vi "COD主界面（列队使用）.vi"() -> (8 "多列列表框":i32(listbox))   [LabVIEW 2016, in "斯坦道CODMn.lvlib"]
uses:
  <vilib>/Analysis/6fits.llb/Curve Fitting Criteria.ctl
  <vilib>/Utility/miscctls.llb/LVPointTypeDef.ctl
  <vilib>/Utility/config.llb/Read Key (I32).vi
  <vilib>/Utility/config.llb/Read Key (Double).vi
  <vilib>/Utility/config.llb/Read Key (Boolean).vi
  <vilib>/Utility/config.llb/Write Key (I32).vi
  <vilib>/Utility/config.llb/Write Key (Double).vi
  <vilib>/Utility/config.llb/Write Key (Boolean).vi
  <vilib>/Waveform/WDTFileIO.llb/Read Waveform from File.vi
  <vilib>/ptbypt/NI_PtbyPt.lvlib
  <vilib>/Utility/config.llb/NI_LVConfig.lvlib
  <vilib>/Analysis/NI_AALPro.lvlib
panel:
  in  "温度曲线":bool
  out "温度波形时间":timestamp
  in  "历史波形 2":bool
  out "时间-温度":u16[](array[numeric]) caption="数组"
  in  "关闭 4":bool
  out "时间温度曲线":u16[](graph)
  in  "加标回收量程：":enum32{"H", "L", "AUTO"}(ring)=enum."AUTO"
  in  "定时设置":cluster{"启动":bool, "控制命令":T1, "测量参数":T2}(xcontrol)
  out "氢氧化钠":dbl
  in  "序列号变更":bool
  out "模块版本号":string
  in  "更新程序":bool
  out "进样无液体告警":bool
  out "校准内容显示":string
  out "60分钟超时报警":bool
  in  "远程校准量程":enum16{"L", "H"}(ring)
  in  "远程自动校准浓度":dbl
  in  "仪器参数":bool
  out "CODMn序列号":string
  out "CODMn软件版本：":string
  in  "标样核查量程选择":enum32{"H", "L", "AUTO"}(ring)=enum."AUTO"
  in  "标样浓度":dbl
  in  "零点核查量程选择":enum32{"H", "L", "AUTO"}(ring)=enum."AUTO"
  in  "零点核查浓度":dbl
  out "序列号":string
  in  "采水泵排液时间/s:":i32
  in  "采水泵润洗时间/s:":i32
  in  "采水泵沉淀时间/s:":i32
  in  "采水泵进样时间/s:":i32
  in  "常规版/认证版":enum16{"常规版-酸性", "常规版-碱性", "认证版", "浮台版"}(ring)
  in  "释放串口":bool
  in  "打开串口":bool
  in  "保存参数":dbl[](array[numeric])
  out "报警数字":i16
  out "CODMn工作状态":T3(ring)
  out "ORP-K":string
  out "ORP-B":string
  out "ORP-A":string
  out "x = y?":bool
  out "稀释倍数解释":string
  in  "跨度量程选择":enum32{"H", "L", "AUTO"}(ring)=enum."AUTO"
  in  "跨度液浓度":dbl
  in  "水样：":dbl
  in  "蒸馏水：":dbl
  in  "标液：":dbl
  in  "零点核查样：":dbl
  in  "加标回收样：":dbl
  in  "草酸钠":dbl
  in  "高锰酸钾":dbl
  in  "硫酸":dbl
  out "量程解释说明":string
  in  "高切低阈值:":dbl
  in  "低切高阈值:":dbl
  in  "水样量程选择:":enum16{"L", "H", "自动切换测一次", "自动切换测两次"}(ring)
  in  "氢氧化钠：":dbl
  in  "标准液浓度":dbl
  in  "温度":dbl
  in  "恒温时间":dbl
  in  "当前量程：":enum16{"L", "H"}(ring)
  in  "CODMn零点核查选择":enum16{"零点核查走纯水管", "零点核查走零漂管"}(ring)
  in  "锁定按钮":bool
  in  "低量程稀释倍数:":i8=1
  in  "高量程稀释倍数:":i8=2
  in  "一键写入":bool
  in  "测量模式(公式)":u16(ring)=1 items=["水样测试"=1, "标样核查"=2, "零点核查"=3, "跨度核查"=4, "空白测试"=5, "平行样"=6, "加标回收"=7]
  out "基本量程(显示)":string
  out "测量模式(显示)":string
  out "数据时间":string
  out "断电排液标记":bool
  out "COM":string
  in  "启用5":bool
  in  "校准5":bool
  in  "泵滴定数5":dbl
  in  "浓度5":dbl
  in  "启用4":bool
  in  "校准4":bool
  in  "泵滴定数4":dbl
  in  "浓度4":dbl
  out "波形时间":timestamp
  in  "历史波形":bool
  out "滴定数-ORP值":u16[](array[numeric]) caption="数组"
  in  "关闭 3":bool
  in  "滴定曲线":bool
  out "ORP滴定曲线":u16[](graph)
  out "空白测试标记":bool
  out "跨度核查标记":bool
  in  "量程选择":enum16{"低量程", "高量程", "0-2量程"}(ring)
  in  "手动控制":bool
  in  "选用水样":enum16{"葡萄糖", "草酸钠"}(ring)
  in  "方程系数":cluster{"K":dbl, "b":dbl, "X^2":dbl} {"X^2" format="%#.6g"; "b" format="%#.6g"; "K" format="%#.6g"}
  out "多项式系数":dbl[](array[numeric])
  out "XY图":cluster{"X Values":dbl[], "Y Values":dbl[]}[](graph)
  in  "模型":enum32{"线性", "多项式"}(ring)
  out "启动时间":timestamp format="%<%Y/%m/%d %H:%M:%S>T"
  in  "关闭 2":bool
  out "r^2":dbl format="%.8g"
  out "拟合公式":string
  out "b":dbl format="%#.4g"
  out "K":dbl format="%#.4f"
  in  "启用3":bool
  in  "启用2":bool
  in  "启用1":bool
  in  "校准3":bool
  in  "校准2":bool
  in  "校准1":bool
  in  "泵滴定数3":dbl
  in  "泵滴定数2":dbl
  in  "泵滴定数1":dbl
  in  "浓度3":dbl
  in  "浓度2":dbl
  in  "浓度1":dbl
  in  "写入":bool
  out "零点核查标记":bool
  out "排液故障":bool
  out "进水样超量程":bool
  out "标样核查标记":bool
  out "平行样测量":bool
  out "加标回收测量":bool
  out "质控样测量":bool
  out "待机":bool
  out "校标错误":bool
  out "校零错误":bool
  out "测量错误":bool
  out "草酸钠报警":bool
  out "高锰酸钾报警":bool
  out "加热故障":bool
  out "温控器故障":bool
  out "ORP故障":bool
  out "排液标记":bool
  out "故障标记":bool
  out "校标标记":bool
  out "校零标记":bool
  out "通讯状态":bool
  out "水样测量":bool
  in  "读取":bool
  in  "返回":bool
  in  "校准配置":bool
  in  "零点泵计量数 2":dbl
  in  "标度泵计量数 2":dbl
  out "标度滴定值":dbl
  out "零点滴定值":dbl
  in  "保存":bool
  in  "关闭":bool
  out "仪器时间":timestamp format="%<%Y/%m/%d %H:%M:%S>T"
  out "秒":u16
  out "分":u16
  out "COD浓度（mg/L)":dbl format="%.2g"
  out "进样管":dbl
  out "高锰酸钾":dbl
  out "草酸钠":dbl
  out "硫酸":dbl
  out "实时ORP":dbl
  out "温度℃":dbl
  out "加热":bool
  out "搅拌":bool
  out "进硫酸":bool
  out "进加标回收样":bool
  out "进零点核查样":bool
  out "进标液":bool
  out "进蒸馏水":bool
  out "进水样":bool
  out "进草酸钠":bool
  out "进高锰酸钾":bool
  in  "启动":bool
  in  "故障清除":bool
  in  "参数配置":bool
  in  "停止":bool
  in  "单步启动":bool
  out "系统时间":timestamp
  in  "时间校准":bool
  out "模式（受控）":u16
  # "测试时长："
  # "注：遇到加热故障和排液故障时仪器不能正常启动，\n必须排查故障并点击报警清除按钮方可运行。"
  # "mg/L"
  # "基本参数设置"
  # "校零校标结果"
  # "泵计量参数设置"
  # "校零结果："
  # "校零滴定值："
  # "高锰酸钾："
  # "加热恒温温度(℃):"
  # "草酸钠："
  # "校标结果："
  # "标度滴定值："
  # "恒温时间(分钟):"
  # "零点泵计量值："
  # "硫酸："
  # "标准液浓度(mg/L):"
  # "标度泵计量值："
  # "跨度核查浓度："
  # "跨度核查量程："
  # "零点核查浓度："
  # "标样浓度："
  # "零点核查量程："
  # "标样核查量程："
  # "远程校准配置区"
  # "公式读取写入区"
  # "mg/L"
  # "是否启用"
  # "泵滴定数"
  # "浓度"
  # "辅\n助\n计\n算\n区"
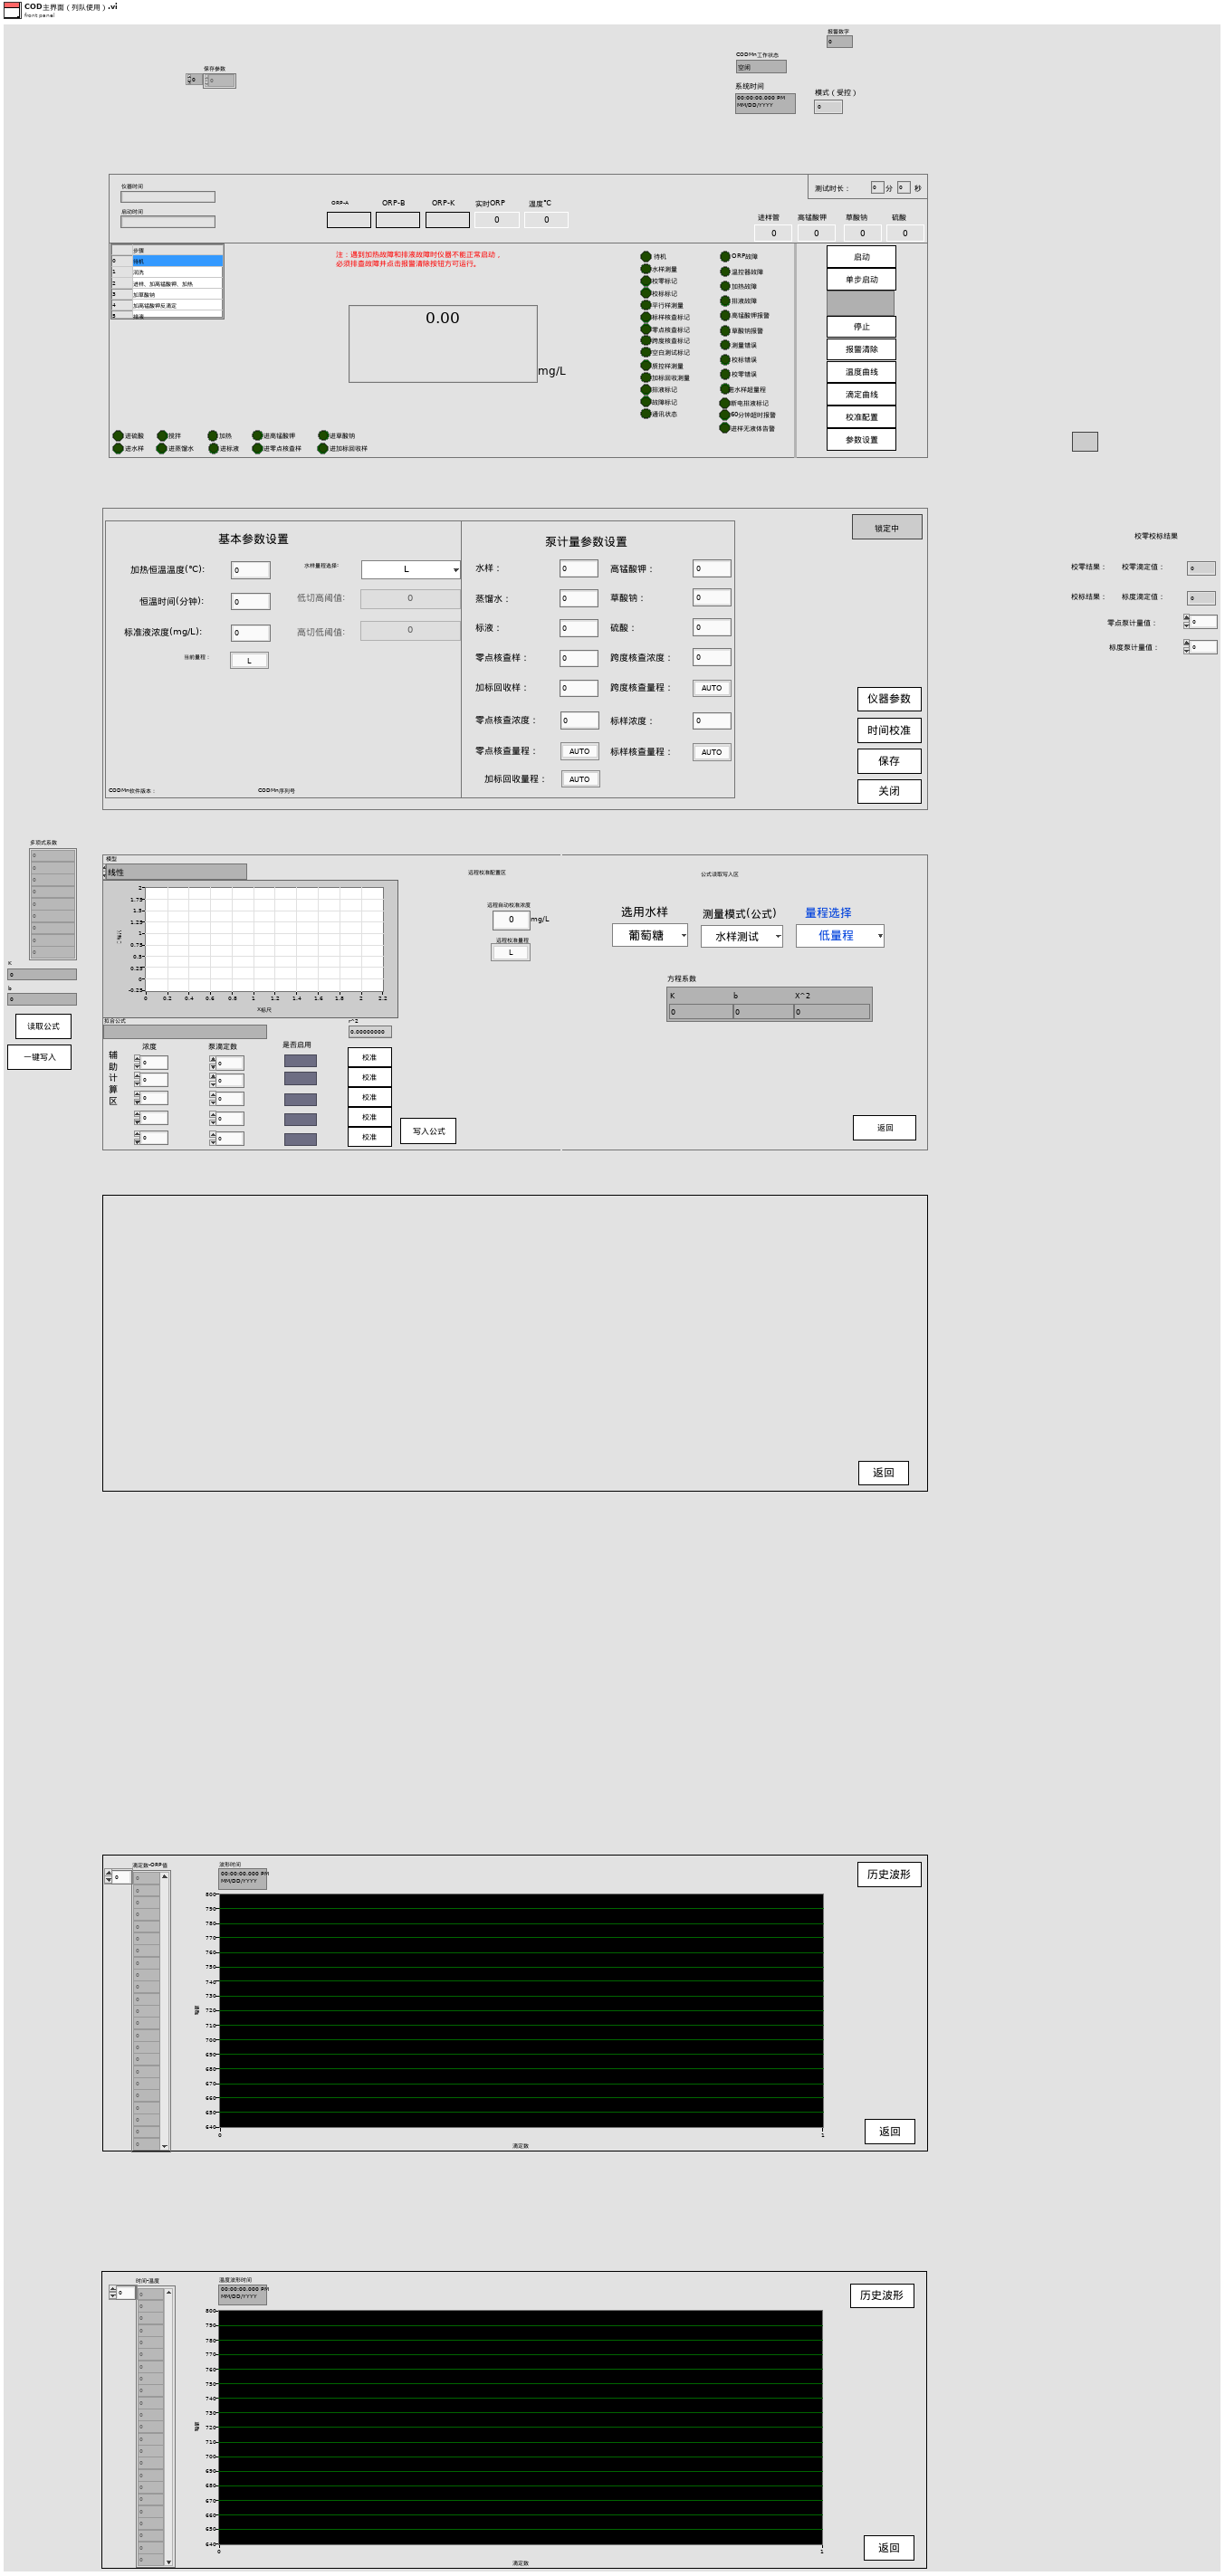
[diagram p1: front panel]
types:
  T1 = typedef "定时设置.xctl/国标控制命令.ctl" = enum16{"启动测量", "标样核查", "零点核查", "跨度核查", "空白测试", "平行样测试", "加标回收", "空白校准", "标样校准", "初始化（清洗）", "停止测试", "仪器重启", "校时", "模式设置", "测量间隔设置"}
  T2 = typedef "定时设置.xctl/测量参数.ctl" = u16
  T3 = enum16{"空闲", "水样测试", "标样核查", "零点核查", "跨度核查", "空白测试", "平行样测试", "质控样", "空白校准", "标样校准", "加标回收"}
  T4 = typedef "LVPointTypeDef.ctl" = cluster{"Horizontal":i16, "Vertical":i16}
  T5 = cluster{"Major":u16, "Minor":u16, "Fix":u16, "Build":u16}
  T6 = typedef "NI_LVConfig.lvlib/Config Data RefNum.ctl" = refnum<k1>
  T7 = cluster{"时间源选择":enum16{"系统时间源", "仪器时间源"}, "外部时间源":timestamp}
  T8 = enum32{"Bad", "Idle", "Run top level", "Running"}
  T9 = enum8{"Enabled", "Disabled", "Disabled and Grayed Out"}
  T10 = cluster{"时间":timestamp, "测量模式":string, "数据类型":string, "检测值":sgl, "单位":string, "数据标识":string, "因子编码":string, "标样参考值":sgl, "ORP-A":sgl, "ORP-B":sgl, "ORP-K":sgl, "COD滴定值":sgl, "高锰酸钾滴定数":sgl, "温度":sgl, "量程":sgl, "LastTime":timestamp, "序列号:":string}
  T11 = cluster{"因子编码":u32, "单位":u16, "标样参考值":sgl, "水样数据时间":timestamp, "水样实测值":sgl, "水样数据标识":string, "标样数据时间":timestamp, "标样实测值":sgl, "标样数据标识":string, "空白数据时间":timestamp, "空白实测值":sgl, "空白数据标识":string, "零点核查数据时间":timestamp, "零点核查实测值":sgl, "零点核查数据标识":string, "跨度核查数据时间":timestamp, "跨度核查实测值":sgl, "跨度核查数据标识":string, "加标回收数据时间":timestamp, "加标回收实测值":sgl, "加标回收数据标识":string, "平行样数据时间":timestamp, "平行样实测值":sgl, "平行样数据标识":string}
  T12 = cluster{"运行模式":enum16{"维护模式", "常规模式", "应急模式", "质控模式"}, "质控频次":enum16{"关闭", "每天", "星期一", "星期二", "星期三", "星期四", "星期五", "星期六", "星期日"}, "空白核查时间":u16, "跨度核查时间":u16, "24H周期设置":bool[]}
  T13 = cluster{"数组 2[0]":sgl, "数组 2[1]":sgl, "数组 2[2]":sgl, "数组 2[3]":sgl, "数组 2[4]":sgl, "数组 2[5]":sgl, "数组 2[6]":sgl, "数组 2[7]":sgl, "数组 2[8]":sgl, "数组 2[9]":sgl, "数组 2[10]":sgl, "数组 2[11]":sgl, "数组 2[12]":sgl, "数组 2[13]":sgl, "数组 2[14]":sgl, "数组 2[15]":sgl, "数组 2[16]":sgl, "数组 2[17]":sgl, "数组 2[18]":sgl, "数组 2[19]":sgl, "数组 2[20]":sgl, "数组 2[21]":sgl, "数组 2[22]":sgl, "数组 2[23]":sgl, "数组 2[24]":sgl, "数组 2[25]":sgl, "数组 2[26]":sgl, "数组 2[27]":sgl, "数组 2[28]":sgl, "数组 2[29]":sgl, "数组 2[30]":sgl, "数组 2[31]":sgl, "数组 2[32]":sgl, "数组 2[33]":sgl, "数组 2[34]":sgl, "数组 2[35]":sgl, "数组 2[36]":sgl, "数组 2[37]":sgl, "数组 2[38]":sgl, "数组 2[39]":sgl, "数组 2[40]":sgl, "数组 2[41]":sgl}
  T14 = cluster{"ORP故障":bool, "温控器故障":bool, "加热故障":bool, "高锰酸钾报警":bool, "草酸钠报警":bool, "测量错误":bool, "校零错误":bool, "校标错误":bool, " 进水样超量程":bool, "排液阀故障":bool, "60分钟超时报警":bool, "进样无液体报警":bool}
  T15 = cluster{"时间标识":timestamp, "参数":string, "日志信息":string, "流程参数":string}
  T16 = cluster{"测量量程":dbl, "测量精度":dbl, "测量间隔":dbl, "消解温度":dbl, "消解时长":dbl, "空白校准时间":timestamp, "曲线截距":dbl, "曲线斜率":dbl, "测量检出限":dbl, "测量信号值":dbl, "线性相关系数":dbl, "二次多项式系数":dbl, "标样校准时间":timestamp, "稀释倍数":dbl, "三项式系数":dbl, "空白标定系数":dbl, "量程系数":dbl, "F0/ORPA":dbl, "F1/ORPB":dbl, "F2/ORPK":dbl, "F3":dbl, "F4":dbl, "F5":dbl, "F6":dbl, "F7":dbl, "X0/滴定数":dbl, "量程":dbl}
  T17 = cluster{"确定":bool, "测量量程":dbl, "测量精度":dbl, "测量间隔":dbl, "消解温度":dbl, "消解时长":dbl, "空白校准时间":timestamp, "曲线截距":dbl, "曲线斜率":dbl, "测量检出限":dbl, "测量信号值":dbl, "线性相关系数":dbl, "二次多项式系数":dbl, "标样校准时间":timestamp, "稀释倍数":dbl, "三项式系数":dbl, "空白标定系数":dbl, "量程系数":dbl, "F0/ORPA":dbl, "F1/ORPB":dbl, "F2/ORPK":dbl, "F3":dbl, "F4":dbl, "F5":dbl, "F6":dbl, "F7":dbl, "X0/滴定数":dbl, "量程":dbl}
  T18 = enum16{"Left Button", "Center Button", "Right Button", "Window Close"}
  T19 = cluster{"时间标识":timestamp, "设备":string, "日志信息":string, "流程参数":string}
  T20 = typedef "NI_AALPro.lvlib/Curve Fitting Criteria.ctl" = u16
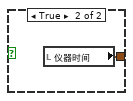
[diagram p2: hidden frame]
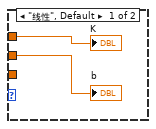
[diagram p8: hidden frame]
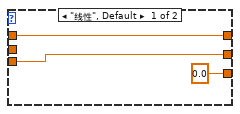
[diagram p10: hidden frame]
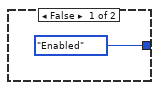
[diagram p11: hidden frame]
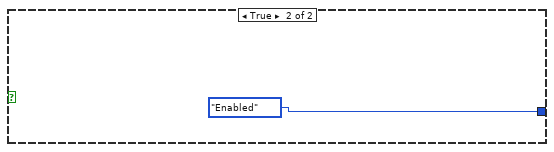
[diagram p12: hidden frame]
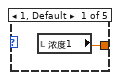
[diagram p17: hidden frame]
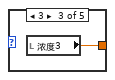
[diagram p18: hidden frame]
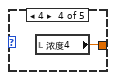
[diagram p19: hidden frame]
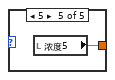
[diagram p20: hidden frame]
diagram:
  n1 = flat-sequence {
    tunnel: w3 -> [_]
    frame #0 {
      w29 = u16 1 items=["水样测试"=1, "标样核查"=2, "零点核查"=3, "跨度核查"=4, "空白测试"=5, "平行样"=6, "加标回收"=7] ("测量模式(公式)")
      n2 = vi-ref "斯坦道CODMn.lvlib:待机状态数据存储写入和切换量程(子VI).vi"() -> (w65:refnum<vi>)
      n3 = vi-ref "斯坦道CODMn.lvlib:日志报警状态存储 (子VI).vi"() -> (w58:refnum<vi>)
      n4 = vi-ref "斯坦道CODMn.lvlib:高锰酸钾-ORP滴定曲线(子VI).vi"() -> (w45:refnum<vi>)
      n5 = property class="VI"(reference=w58, error in=errorcluster {"status"=FALSE, "code"=0, "source"=""} ("错误输出")) -> ("Name"=w57:string)  [unwired: 2 out]
      n6 = property class="VI"(reference=w45, error in=errorcluster {"status"=FALSE, "code"=0, "source"=""} ("错误输出")) -> ("Name"=w46:string)  [unwired: 2 out]
      n7 = property class="VI"(reference=w65, error in=errorcluster {"status"=FALSE, "code"=0, "source"=""} ("错误输出")) -> ("Name"=w64:string)  [unwired: 2 out]
      n8 = Open VI Reference(type specifier VI Refnum (for type only)=refnum<vi> refnum, vi path=w57, options=128 ("选项")) -> (vi reference=w41:refnum<vi>, error out=w55:errorcluster)  [unwired: 3 in]
      n9 = Open VI Reference(type specifier VI Refnum (for type only)=refnum<vi> refnum, vi path=w46, options=128 ("选项")) -> (vi reference=w44:refnum<vi>, error out=w48:errorcluster)  [unwired: 3 in]
      n10 = call-by-ref "?"(reference=w41, error in=w55) -> (reference out=w53:refnum<vi>, error out=w54:errorcluster)  [unwired: 12 in]
      n11 = call-by-ref "?"(reference=w44, error in=w48) -> (reference out=w50:refnum<vi>, error out=w49:errorcluster)  [unwired: 12 in]
      n12 = Open VI Reference(type specifier VI Refnum (for type only)=refnum<vi> refnum, vi path=w64, options=128 ("选项")) -> (vi reference=w39:refnum<vi>, error out=w62:errorcluster)  [unwired: 3 in]
      n13 = Close Reference(reference=w53, error in (no error)=w54) -> ()  [unwired: 1 out]
      n14 = call-by-ref "?"(reference=w39, error in=w62) -> (reference out=w60:refnum<vi>, error out=w61:errorcluster)  [unwired: 12 in]
      n15 = Close Reference(reference=w50, error in (no error)=w49) -> ()  [unwired: 1 out]
      n16 = Close Reference(reference=w60, error in (no error)=w61) -> ()  [unwired: 1 out]
      n17 = vi-ref "斯坦道CODMn.lvlib:时间-温度曲线(子VI).vi"() -> (w24:refnum<vi>)
      n18 = vi-ref "斯坦道CODMn.lvlib:关键参数交互.vi"() -> (w36:refnum<vi>)
      n19 = property class="VI"(reference=w36, error in=errorcluster {"status"=FALSE, "code"=0, "source"=""} ("错误输出")) -> ("Name"=w35:string)  [unwired: 2 out]
      n20 = property class="VI"(reference=w24, error in=errorcluster {"status"=FALSE, "code"=0, "source"=""} ("错误输出")) -> ("Name"=w23:string)  [unwired: 2 out]
      n21 = Open VI Reference(type specifier VI Refnum (for type only)=refnum<vi> refnum, vi path=w35, options=128 ("选项")) -> (vi reference=w37:refnum<vi>, error out=w33:errorcluster)  [unwired: 3 in]
      n22 = call-by-ref "?"(reference=w37, error in=w33, "量程选择"=enum16{"低量程", "高量程", "0-2量程"}."低量程", "测量模式(公式)"=w29, "模型"=enum32{"线性", "多项式"}."线性") -> (reference out=w31:refnum<vi>, error out=w32:errorcluster)  [unwired: 9 in]
      n23 = Open VI Reference(type specifier VI Refnum (for type only)=refnum<vi> refnum, vi path=w23, options=128 ("选项")) -> (vi reference=w25:refnum<vi>, error out=w21:errorcluster)  [unwired: 3 in]
      n24 = call-by-ref "?"(reference=w25, error in=w21) -> (reference out=w19:refnum<vi>, error out=w20:errorcluster)  [unwired: 12 in]
      n25 = Close Reference(reference=w31, error in (no error)=w32) -> ()  [unwired: 1 out]
      n26 = Close Reference(reference=w19, error in (no error)=w20) -> ()  [unwired: 1 out]
    }
  }
  n27 = property on="定时设置" class="定时设置 (严格)"("引用参数"="CODMn") -> (error out=w1:errorcluster)  [unwired: 2 in, 1 out]
  n28 = flat-sequence {
    tunnel: [w68] -> w5
    tunnel: [errorcluster {"status"=FALSE, "code"=0, "source"=""} ("错误输出")] -> w3
    tunnel: [w70] -> w4
    frame #0 {
      w92 = "192.168.1.100" ("名称")
      n29 = global write "COD内部交互全局.vi" "量程切换次数"(u8 0 ("量程切换次数")) -> ()
      n30 = global write "COD内部交互全局.vi" "切换量程连续测两次"(FALSE ("切换量程连续测两次")) -> ()
      n31 = global read "COD内部交互全局.vi" "序列号:"() -> (w99:string)
      n32 = property on="窗格" class="Pane"("Origin"=T4 {"Horizontal"=0, "Vertical"=0} ("原点")) -> ()  [unwired: 2 in, 2 out]
      n33 = Empty String/Path?(string/path=w99) -> (empty?=w67:bool)
      n34 = case shown="真" w67 {
        tunnel: w99 -> [w114 _]
        tunnel: [w113 "data\\CODMnSet.ini" ("名称或相对路径")] -> w80
        frame False {
          # "与生产用上位机交互"
          n35 = Concatenate Strings("data\\" ("字符串"), "序列号" ("字符串"), w114, "Set.ini" ("名称或相对路径")) -> (w113:string)
        }
        frame True {
        }
      }
      n36 = String To IP(1:w92) -> (0:w85:u32)
      n37 = IP To String(2:w85) -> (0:w88:string)  [unwired: 1 in]
      n38 = Not Equal?(x=w92, y=w88) -> (x != y?=w93:bool)
      n39 = Concatenate Strings("\\\\" ("字符串"), w88) -> (w87:string)
      n40 = global write "CODMN外部API.vi" "ping"(w93) -> ()
      n41 = String To Path(string=w87) -> (path=w94:path)
      n42 = Build Path(base path=w94, name or relative path=w80) -> (appended path=w89:path)
      n43 = local write "量程选择"(enum16{"低量程", "高量程", "0-2量程"}."低量程" ("量程选择")) -> ()
      n44 = local write "选用水样"(enum16{"葡萄糖", "草酸钠"}."葡萄糖" ("选用水样")) -> ()
      n45 = global write "COD内部交互全局.vi" "配置文件ini"(w80) -> ()
      n46 = case shown="真" w93 {
        tunnel: w89 -> [w104 w108]
        tunnel: [w104 w107] -> w90
        tunnel: [FALSE w106] -> w91
        frame False {
        }
        frame True {
          n47 = call <vilib>:"Check if File or Folder Exists.vi"("path"=w108) -> ("file or folder exists?"=w106:bool, "dup path"=w107:path)  [unwired: 8 in, 1 out]
        }
      }
      n48 = control-ref of="本VI"() -> (w79:refnum<vi>)
      n49 = case shown="假" w91 {
        tunnel: w90 -> [_ w112]
        tunnel: [w110 w112] -> w71
        tunnel: w80 -> [w109 _]
        frame False {
          # "本地文件地址"
          n50 = call <vilib>:"Application Directory.vi"() -> ("Application Directory"=w111:path)
          n51 = Build Path(base path=w111, name or relative path=w109) -> (appended path=w110:path)
        }
        frame True {
          # "网络共享地址"
        }
      }
      n52 = property class="VI"(reference=w79) -> ("Library.Version"=w78:T5)  [unwired: 1 in, 2 out]
      n53 = Unbundle By Name(w78) -> ("Major"=w76:u16, "Minor"=w75:u16, "Fix"=w74:u16, "Build"=w73:u16)
      n54 = Format Into String(format string="模块版本号：%d.%d.%d.%d" ("格式字符串"), w76, w75, w74, w73) -> (resulting string=→"模块版本号":string)  [unwired: 2 in, 1 out]
      n55 = global write "CODMN外部API.vi" "配置文件 path"(w71) -> ()
      n56 = call <vilib>:"Open Config Data.vi"("configuration file path"=w71) -> ("error out"=w81:errorcluster, "refnum"=w82:T6)  [unwired: 8 in, 1 out]
      n57 = vi-ref "斯坦道CODMn.lvlib:CODMn断电保存全局变量.vi"() -> (w95:refnum<vi>)
      n58 = call <userlib>:"Read Panel from INI__ogtk.vi"("error in (no error)"=w81, "VI ref"=w95, "refnum"=w82) -> ("error out"=w83:errorcluster, "refnum out"=w84:T6)  [unwired: 7 in]
      n59 = call <vilib>:"Close Config Data.vi"("error in (no error)"=w83, "refnum"=w84) -> ("error out"=w69:errorcluster)  [unwired: 8 in, 1 out]
      n60 = call <vilib>:"Clear Errors.vi"("error in (no error)"=w69) -> ("error out"=w66:errorcluster)  [unwired: 5 in, 1 out]
      n61 = Read from Text File(file (use dialog)=w71, error in=w66) -> (text=w70:string, error out=w68:errorcluster)  [unwired: 2 in, 2 out]
      "稀释倍数解释" <- "稀释倍数解释：\n稀释倍数选择1，表示不稀释\n默认低量程系数倍数1，高量程系数倍数2\n则低量程为0~8，高量程为0~16" ("稀释倍数解释")
    }
  }
  n62 = while {
    tunnel: w1 -> [_]
    stop <- FALSE stop-if-true
    n63 = Wait (ms)(milliseconds to wait=u32 500 ("等待时间（毫秒）")) -> ()  [unwired: 1 out]
    n64 = global read "COD测量模式全局.vi" "CODMn工作状态"() -> (w125:T3)
    n65 = local read "通讯状态"() -> (w119:bool)
    n66 = case shown="假" w119 {
      tunnel: [w135 w136] -> w123
      frame False {
        n67 = Get Date/Time In Seconds() -> (seconds since 1Jan1904=w135:timestamp)
      }
      frame True {
        n68 = local read "仪器时间"() -> (w136:timestamp)
      }
    }
    n69 = vi-ref "斯坦道CODMn.lvlib:CODMn测量流程.vi"() -> (w132:refnum<vi>)
    n70 = Bundle By Name(cluster=T7 {"时间源选择"=enum."系统时间源", "外部时间源"=timestamp(0 s since 1904-01-01)} ("时间源"), "时间源选择"=enum16{"系统时间源", "仪器时间源"}."仪器时间源", "外部时间源"=w123) -> (w121:T7)
    n71 = property class="VI"(reference=w132) -> ("Exec.State"=w130:T8, "Name"=w131:string)  [unwired: 1 in, 2 out]
    n72 = Not Equal?(x=w125, y=T3."空闲") -> (x != y?=w120:bool)
    n73 = property on="定时设置" class="定时设置 (严格)"("仪器状态"=w120, "时间源"=w121) -> ()  [unwired: 2 in, 2 out]
    n74 = Unbundle By Name("定时设置") -> ("启动"=w128:bool, "控制命令"=w129:T1)
    n75 = case shown="真" w128 {
      tunnel: w131 -> [_ w139]
      tunnel: w129 -> [_ w138]
      tunnel: w130 -> [_ w137]
      frame False {
      }
      frame True {
        n76 = case shown="\"Idle\"" w137 {
          tunnel: w139 -> [_ w143]
          tunnel: w138 -> [_ w140]
          frame "Bad", Default {
          }
          frame "Idle" {
            n77 = Open VI Reference(type specifier VI Refnum (for type only)=refnum<vi> refnum, vi path=w143, options=128 ("选项")) -> (vi reference=w144:refnum<vi>, error out=w145:errorcluster)  [unwired: 3 in]
            n78 = call-by-ref "开始异步调用"(reference=w144, error in=w145, "控制命令"=w140) -> (reference out=w146:refnum<vi>, error out=w147:errorcluster)  [unwired: 11 in]
            n79 = Close Reference(reference=w146, error in (no error)=w147) -> ()  [unwired: 1 out]
          }
        }
      }
    }
  }
  n80 = Obtain Queue(name (unnamed)="CODMn" ("名称（未命名）"), element data type=cluster{"命令":string} {"命令"="启用模块"} ("元素")) -> (queue out=w15:refnum<queue>, error out=w14:errorcluster)  [unwired: 3 in, 1 out]
  n81 = while {
    tunnel: [w154] -> _
    shift-right: [w152] -> _
    shift-left: w4 -> [w151]
    tunnel: w5 -> [_]
    stop <- FALSE stop-if-true
    n82 = global read "CODMN外部API.vi" "配置文件 path"() -> (w148:path)
    n83 = Wait (ms)(milliseconds to wait=u32 1000 ("等待时间（毫秒）")) -> ()  [unwired: 1 out]
    n84 = Read from Text File(file (use dialog)=w148) -> (text=w152:string, error out=w149:errorcluster)  [unwired: 3 in, 2 out]
    n85 = Not Equal?(x=w152, y=w151) -> (x != y?=w150:bool)
    n86 = case shown="真" w150 {
      tunnel: [w156 w163] -> w154
      tunnel: w148 -> [_ w157]
      tunnel: w149 -> [w156 _]
      frame False {
      }
      frame True {
        # "文件发生改变进行更新，远端和本地都更新"
        n87 = vi-ref "斯坦道CODMn.lvlib:CODMn断电保存全局变量.vi"() -> (w158:refnum<vi>)
        n88 = call <vilib>:"Open Config Data.vi"("configuration file path"=w157) -> ("error out"=w162:errorcluster, "refnum"=w161:T6)  [unwired: 8 in, 1 out]
        n89 = call <userlib>:"Read Panel from INI__ogtk.vi"("error in (no error)"=w162, "VI ref"=w158, "refnum"=w161) -> ("error out"=w160:errorcluster, "refnum out"=w159:T6)  [unwired: 7 in]
        n90 = call <vilib>:"Close Config Data.vi"("error in (no error)"=w160, "refnum"=w159) -> ("error out"=w163:errorcluster)  [unwired: 8 in, 1 out]
      }
    }
  }
  n91 = vi-ref "CODMn通讯.vi"() -> (w6:refnum<vi>)
  n92 = while {
    tunnel: w5 -> [_]
    stop <- FALSE stop-if-true
    # "赋值循环"
    n93 = flat-sequence {
      frame #0 {
        # "测量数据区"
        n94 = global read "COD内部交互全局.vi" "data"() -> (w408:T10)
        n95 = global read "COD测量模式全局.vi" "测量模式文字实时"() -> (w394:string)
        "测量模式(显示)" <- w394
        n96 = global read "CODMn断电保存全局变量.vi" "测量数据区"() -> (w403:T11)
        n97 = Unbundle By Name(w408) -> ("时间"=w407:timestamp, "检测值"=w406:sgl, "数据标识"=w405:string)
        n98 = case shown="\"水样测试\"" w394 {
          tunnel: w403 -> [w409 w414 w419 w424 w429 w434 w439 w444 w449 w454]
          tunnel: [w409 w413 w418 w420 w428 w433 w438 w443 w445 w453] -> w404
          tunnel: w407 -> [_ w412 w417 w423 w427 w432 w437 w442 w448 w452]
          tunnel: w406 -> [_ w411 w416 w422 w426 w431 w436 w441 w447 w451]
          tunnel: w405 -> [_ w410 w415 w421 w425 w430 w435 w440 w446 w450]
          frame "", Default {
          }
          frame "水样测试" {
            n99 = Bundle By Name(cluster=w414, "水样数据时间"=w412, "水样实测值"=w411, "水样数据标识"=w410) -> (w413:T11)
          }
          frame "标样核查" {
            n100 = Bundle By Name(cluster=w419, "标样数据时间"=w417, "标样实测值"=w416, "标样数据标识"=w415) -> (w418:T11)
          }
          frame "跨度核查" {
            n101 = Bundle By Name(cluster=w424, "跨度核查数据时间"=w423, "跨度核查实测值"=w422, "跨度核查数据标识"=w421) -> (w420:T11)
          }
          frame "零点核查" {
            n102 = Bundle By Name(cluster=w429, "零点核查数据时间"=w427, "零点核查实测值"=w426, "零点核查数据标识"=w425) -> (w428:T11)
          }
          frame "空白测试" {
            n103 = Bundle By Name(cluster=w434, "空白数据时间"=w432, "空白实测值"=w431, "空白数据标识"=w430) -> (w433:T11)
          }
          frame "加标回收" {
            n104 = Bundle By Name(cluster=w439, "加标回收数据时间"=w437, "加标回收实测值"=w436, "加标回收数据标识"=w435) -> (w438:T11)
          }
          frame "平行样" {
            n105 = Bundle By Name(cluster=w444, "平行样数据时间"=w442, "平行样实测值"=w441, "平行样数据标识"=w440) -> (w443:T11)
          }
          frame "校零" {
            n106 = Bundle By Name(cluster=w449, "空白数据时间"=w448, "空白实测值"=w447, "空白数据标识"=w446) -> (w445:T11)
          }
          frame "校标" {
            n107 = Bundle By Name(cluster=w454, "标样数据时间"=w452, "标样实测值"=w451, "标样数据标识"=w450) -> (w453:T11)
          }
        }
        n108 = Unbundle By Name(w403) -> ("水样实测值"=w400:sgl)
        n109 = feedback-in #1(w403) -> ()
        n110 = feedback #1(w403) -> (w402:T11)
        n111 = global read "CODMn断电保存全局变量.vi" "水样测试量程"() -> (w396:enum16{"L", "H"})
        n112 = Unbundle By Name(w402) -> ("水样实测值"=w401:sgl)
        n113 = feedback #2(w396) -> (w397:enum16{"L", "H"})
        n114 = feedback-in #2(w396) -> ()
        n115 = Not Equal?(x=w397, y=w396) -> (x != y?=w395:bool)
        n116 = Not Equal?(x=w400, y=w401) -> (x != y?=w399:bool)
        n117 = global write "CODMn断电保存全局变量.vi" "测量数据区"(w404) -> ()
        n118 = Or(x=w399, y=w395) -> (x .or. y?=w398:bool)
        n119 = case shown="真" w398 {
          frame False {
          }
          frame True {
            # "水样值发送改变存储本地"
            n120 = call "配置文件保存.vi"() -> ()  [unwired: 12 in]
          }
        }
      }
    }
    n121 = flat-sequence {
      frame #0 {
        # "局部变量给内部交互用全局变量"
        n122 = local read "COD浓度（mg/L)"() -> (w196:dbl)
        n123 = local read "CODMn工作状态"() -> (w199:T3)
        n124 = local read "多列列表框"() -> (w197:i32)
        n125 = local read "标准液浓度"() -> (w195:dbl)
        n126 = local read "温度℃"() -> (w190:dbl)
        n127 = local read "高锰酸钾报警"() -> (w193:bool)
        n128 = local read "断电排液标记"() -> (w192:bool)
        n129 = local read "实时ORP"() -> (w189:dbl)
        n130 = local read "故障标记"() -> (w198:bool)
        n131 = local read "高锰酸钾"() -> (w191:dbl)
        n132 = local read "待机"() -> (w194:bool)
        n133 = global write "COD内部交互全局.vi" "实时温度"(w190) -> ()
        n134 = global write "运行时序全局变量.vi" "多列列表框"(w197) -> ()
        n135 = global write "COD内部交互全局.vi" "故障标记"(w198) -> ()
        n136 = global write "COD内部交互全局.vi" "ORP显示"(w189) -> ()
        n137 = global write "COD浓度全局变量.vi" "标准液浓度"(w195) -> ()
        n138 = global write "COD内部交互全局.vi" "高锰酸钾"(w191) -> ()
        n139 = global write "COD内部交互全局.vi" "待机"(w194) -> ()
        n140 = global write "COD测量模式全局.vi" "CODMn工作状态"(w199) -> ()
        n141 = global write "COD内部交互全局.vi" "高锰酸钾报警"(w193) -> ()
        n142 = global write "COD内部交互全局.vi" "断电排液标记"(w192) -> ()
        n143 = global write "COD浓度全局变量.vi" "COD浓度（mg/L)"(w196) -> ()
      }
    }
    n144 = flat-sequence {
      frame #0 {
        # "断电保存全局给局部变量"
        n145 = global read "CODMn断电保存全局变量.vi" "高切低阈值:"() -> (w471:dbl)
        n146 = global read "CODMn断电保存全局变量.vi" "低切高阈值:"() -> (w470:dbl)
        n147 = global read "CODMn断电保存全局变量.vi" "跨度液浓度"() -> (w468:dbl)
        n148 = global read "COD内部交互全局.vi" "波形时间"() -> (→"波形时间":timestamp)
        n149 = global read "CODMn断电保存全局变量.vi" "启动时间"() -> (→"启动时间":timestamp)
        n150 = global read "CODMn断电保存全局变量.vi" "标样浓度"() -> (w466:dbl)
        n151 = global read "CODMn断电保存全局变量.vi" "CODMn跨度量程选择"() -> (w472:enum32{"H", "L", "AUTO"})
        n152 = global read "CODMn断电保存全局变量.vi" "标样核查量程选择"() -> (w463:enum32{"H", "L", "AUTO"})
        n153 = global read "CODMn断电保存全局变量.vi" "零点核查量程选择"() -> (w465:enum32{"H", "L", "AUTO"})
        n154 = global read "CODMn断电保存全局变量.vi" "加标回收量程选择"() -> (w458:enum32{"H", "L", "AUTO"})
        n155 = global read "COD内部交互全局.vi" "滴定数-ORP值"() -> (→"滴定数-ORP值":u16[])
        n156 = global read "CODMn断电保存全局变量.vi" "常规版/认证版"() -> (w467:enum16{"常规版-酸性", "常规版-碱性", "认证版", "浮台版"})
        n157 = global read "CODMn断电保存全局变量.vi" "自动切换量程:"() -> (w469:enum16{"L", "H", "自动切换测一次", "自动切换测两次"})
        n158 = global read "CODMn断电保存全局变量.vi" "零点核查浓度"() -> (w464:dbl)
        n159 = global read "CODMn断电保存全局变量.vi" "测量模式(公式)"() -> (w473:u16)
        n160 = local write "高切低阈值:"(w471) -> ()
        n161 = local write "跨度液浓度"(w468) -> ()
        n162 = local write "低切高阈值:"(w470) -> ()
        n163 = global read "COD内部交互全局.vi" "ORP滴定曲线"() -> (→"ORP滴定曲线":u16[])
        n164 = local write "标样浓度"(w466) -> ()
        n165 = local write "标样核查量程选择"(w463) -> ()
        n166 = local write "水样量程选择:"(w469) -> ()
        n167 = local write "常规版/认证版"(w467) -> ()
        n168 = local write "零点核查浓度"(w464) -> ()
        n169 = local write "零点核查量程选择"(w465) -> ()
        n170 = local write "加标回收量程："(w458) -> ()
        n171 = local write "测量模式(公式)"(w473) -> ()
        n172 = local write "跨度量程选择"(w472) -> ()
        n173 = global read "COD内部交互全局.vi" "温度波形时间"() -> (→"温度波形时间":timestamp)
        n174 = global read "COD内部交互全局.vi" "时间温度曲线"() -> (→"时间温度曲线":u16[])
        n175 = global read "COD内部交互全局.vi" "时间-温度"() -> (→"时间-温度":u16[])
      }
    }
    n176 = flat-sequence {
      frame #0 {
        # "保存参数赋值"
        n177 = Multiply(x="温度", y=10.0) -> (x*y=w174:dbl)
        n178 = Multiply(x="标准液浓度", y=100.0) -> (x*y=w171:dbl)
        n179 = Build Array(w174, "恒温时间", w171, "氢氧化钠：", "当前量程：", "水样：", "蒸馏水：", "标液：", "零点核查样：", "加标回收样：", "高锰酸钾", "草酸钠", "硫酸", "零点泵计量数 2", "标度泵计量数 2", "高量程稀释倍数:", "低量程稀释倍数:", "CODMn零点核查选择") -> (w168:dbl[])
        n180 = local write "保存参数"(w168) -> ()
      }
    }
    n181 = flat-sequence {
      frame #0 {
        # "显示量程说明"
        n182 = global read "COD内部交互全局.vi" "通讯状态"() -> (→"通讯状态":bool)
        n183 = global read "CODMn断电保存全局变量.vi" "MB通信方式选择"() -> (w474:enum16{"串口", "TCP"})
        n184 = local read "低量程稀释倍数:"() -> (w488:i8)
        n185 = local read "高量程稀释倍数:"() -> (w478:i8)
        n186 = case shown="\"TCP\"" w474 {
          tunnel: [w491 w492] -> w479
          frame "串口", Default {
            n187 = global read "CODMn断电保存全局变量.vi" "VISA resource name"() -> (w491:refnum<visa-resource-name>)
          }
          frame "TCP" {
            n188 = global read "CODMn断电保存全局变量.vi" "IP"() -> (w492:string)
          }
        }
        "COM" <- w479
        n189 = Multiply(x=w488, y=i8 8) -> (x*y=w480:i8)
        n190 = Multiply(x=w478, y=i8 8) -> (x*y=w476:i8)
        n191 = Number To Decimal String(number=w480) -> (decimal integer string=w485:string)  [unwired: 1 in]
        n192 = Number To Decimal String(number=w476) -> (decimal integer string=w483:string)  [unwired: 1 in]
        n193 = Concatenate Strings("L低量程范围:0~" ("量程解释说明"), w485, "(mg/L)\n\nH高量程范围:" ("量程解释说明"), "0" ("字符串"), "~" ("量程解释说明"), w483, "(mg/L)" ("量程解释说明")) -> (→"量程解释说明":string)
      }
    }
    n194 = flat-sequence {
      frame #0 {
        # "参数赋值（只在读取参数时候改变一次）"
        n195 = global read "COD内部交互全局.vi" "读取浮台参数显示"() -> (w201:bool)
        n196 = global read "COD内部交互全局.vi" "读取浮台参数"() -> (w200:u16[])
        n197 = global read "COD内部交互全局.vi" "读取参数显示"() -> (w202:bool)
        n198 = global read "COD内部交互全局.vi" "读取参数"() -> (w203:u16[])
        n199 = case shown="真" w201 {
          tunnel: w200 -> [_ w209]
          frame False {
          }
          frame True {
            n200 = Index Array(array=w209) -> (element #1=w208:u16, element #2=w207:u16, element #3=w206:u16, element #4=w205:u16)  [unwired: 4 in]
            n201 = global write "COD内部交互全局.vi" "读取浮台参数显示"(FALSE ("读取参数显示")) -> ()
            n202 = local write "采水泵进样时间/s:"(w208) -> ()
            n203 = local write "采水泵润洗时间/s:"(w207) -> ()
            n204 = local write "采水泵沉淀时间/s:"(w206) -> ()
            n205 = local write "采水泵排液时间/s:"(w205) -> ()
          }
        }
        n206 = case shown="真" w202 {
          tunnel: w203 -> [_ w227]
          frame False {
          }
          frame True {
            n207 = Index Array(array=w227) -> (element #1=w236:u16, element #2=w248:u16, element #3=w232:u16, element #4=w210:u16, element #5=w235:u16, element #6=w234:u16, element #7=w247:u16, element #8=w246:u16, element #9=w245:u16, element #10=w244:u16, element #11=w243:u16, element #12=w242:u16, element #13=w241:u16, element #14=w240:u16, element #15=w239:u16, element #16=w230:u16, element #17=w229:u16, element #18=w228:u16, element #19=w225:u16, element #20=w224:u16, element #21=w223:u16, element #22=w222:u16, element #23=w221:u16, element #27=w217:u16, element #28=w216:u16, element #29=w215:u16, element #30=w214:u16, element #31=w213:u16)  [unwired: 31 in, 3 out]
            n208 = global write "COD内部交互全局.vi" "读取参数显示"(FALSE ("读取参数显示")) -> ()
            n209 = local write "水样："(w234) -> ()
            n210 = local write "标液："(w246) -> ()
            n211 = local write "硫酸"(w241) -> ()
            n212 = local write "零点核查样："(w245) -> ()
            n213 = local write "加标回收样："(w244) -> ()
            n214 = local write "当前量程："(w235) -> ()
            n215 = local write "蒸馏水："(w247) -> ()
            n216 = local write "恒温时间"(w248) -> ()
            n217 = local write "高锰酸钾"(w243) -> ()
            n218 = local write "草酸钠"(w242) -> ()
            n219 = local write "零点泵计量数 2"(w240) -> ()
            n220 = local write "标度泵计量数 2"(w239) -> ()
            n221 = local write "高量程稀释倍数:"(w230) -> ()
            n222 = local write "低量程稀释倍数:"(w229) -> ()
            n223 = local write "CODMn零点核查选择"(w228) -> ()
            n224 = Build Array(w225, w224, w223, w222, w221) -> (w220:u16[])
            n225 = Build Array(w217, w216, w215, w214, w213) -> (w212:u16[])
            n226 = Divide(x=w236, y=u16 10) -> (x/y=w237:dbl)
            n227 = Divide(x=w232, y=u16 100) -> (x/y=w231:dbl)
            n228 = local write "氢氧化钠："(w210) -> ()
            n229 = local write "温度"(w237) -> ()
            n230 = local write "标准液浓度"(w231) -> ()
            n231 = call "HexToString.vi"("数组"=w212) -> ("字符串"=w211:string)  [unwired: 10 in]
            "CODMn序列号" <- w211
            "序列号" <- w211
            n232 = call "FATEK_HexToString.vi"("数组"=w220) -> ("STRING"=w219:string[])  [unwired: 10 in]
            n233 = Index Array(array=w219) -> (element=→"CODMn软件版本：":string)  [unwired: 1 in]
            n234 = global write "COD内部交互全局.vi" "序列号:"(w211) -> ()
          }
        }
      }
    }
    n235 = flat-sequence {
      frame #0 {
        # "权限隐藏和显示功能"
        n236 = local read "x = y?"() -> (w497:bool)
        n237 = global read "CODMn断电保存全局变量.vi" "CODMn系统周期测试?"() -> (w494:bool)
        n238 = global read "CODMn断电保存全局变量.vi" "运行周期"() -> (w495:T12)
        n239 = property on="更新程序" class="Bool (严格)"("Visible"=w497) -> ()  [unwired: 2 in, 2 out]
        n240 = property on="释放串口" class="Bool"("Visible"=w497) -> ()  [unwired: 2 in, 2 out]
        n241 = property on="打开串口" class="Bool"("Visible"=w497) -> ()  [unwired: 2 in, 2 out]
        n242 = case shown="假" w494 {
          tunnel: w495 -> [_ w521]
          tunnel: [T9."Enabled" ("禁用") w519] -> w493
          frame False {
          }
          frame True {
            n243 = Unbundle By Name(w521) -> ("运行模式"=w520:enum16{"维护模式", "常规模式", "应急模式", "质控模式"})
            n244 = case shown="\"维护模式\", 默认" w520 {
              tunnel: [T9."Enabled" ("禁用") T9."Disabled and Grayed Out" ("禁用") T9."Disabled and Grayed Out" ("禁用") T9."Disabled and Grayed Out" ("禁用")] -> w519
              frame "维护模式", Default {
              }
              frame "常规模式" {
              }
              frame "应急模式" {
              }
              frame "质控模式" {
              }
            }
          }
        }
        n245 = property on="序列号变更" class="Bool"("Visible"=w497) -> ()  [unwired: 2 in, 2 out]
        n246 = property on="常规版/认证版" class="Enum (严格)"("Visible"=w497) -> ()  [unwired: 2 in, 2 out]
        n247 = property on="CODMn零点核查选择" class="Enum (严格)"("Visible"=w497) -> ()  [unwired: 2 in, 2 out]
        n248 = property on="低量程稀释倍数:" class="DigNum (严格)"("Visible"=w497) -> ()  [unwired: 2 in, 2 out]
        n249 = property on="稀释倍数解释" class="Str"("Visible"=w497) -> ()  [unwired: 2 in, 2 out]
        n250 = property on="高量程稀释倍数:" class="DigNum (严格)"("Visible"=w497) -> ()  [unwired: 2 in, 2 out]
        n251 = control-ref of="水样："() -> (w507:refnum<vi>)
        n252 = control-ref of="蒸馏水："() -> (w506:refnum<vi>)
        n253 = control-ref of="标液："() -> (w505:refnum<vi>)
        n254 = control-ref of="零点核查样："() -> (w504:refnum<vi>)
        n255 = control-ref of="加标回收样："() -> (w503:refnum<vi>)
        n256 = local read "水样量程选择:"() -> (w514:enum16{"L", "H", "自动切换测一次", "自动切换测两次"})
        n257 = control-ref of="量程解释说明"() -> (w501:refnum<vi>)
        n258 = control-ref of="氢氧化钠："() -> (w502:refnum<vi>)
        n259 = property on="定时设置" class="定时设置 (严格)"("DisabledEnum"=w493) -> ()  [unwired: 2 in, 2 out]
        n260 = local read "常规版/认证版"() -> (w512:enum16{"常规版-酸性", "常规版-碱性", "认证版", "浮台版"})
        n261 = Not Equal To 0?(x=w514) -> (x != 0?=w513:bool)
        n262 = control-ref of="进样管"() -> (w499:refnum<vi>)
        n263 = case shown="\"浮台版\"" w512 {
          tunnel: [T9."Enabled" ("禁用") T9."Enabled" ("禁用") T9."Disabled and Grayed Out" ("禁用") T9."Enabled" ("禁用")] -> w511
          tunnel: [i32[] [2] ("禁用项[]") i32[] [2] ("禁用项[]") i32[] [] ("禁用项[]") i32[] [2] ("禁用项[]")] -> w510
          tunnel: [w529 w534 T9."Disabled and Grayed Out" ("禁用") w545] -> w509
          tunnel: [w528 FALSE FALSE TRUE] -> w508
          tunnel: [w529 w534 T9."Disabled and Grayed Out" ("禁用") w545] -> w498
          tunnel: [w528 TRUE FALSE FALSE] -> w496
          frame "常规版-酸性", Default {
            w528 = FALSE
            w529 = T9."Enabled" ("禁用")
          }
          frame "常规版-碱性" {
            w534 = T9."Enabled" ("禁用")
          }
          frame "认证版" {
            w540 = u16 1 items=["水样测试"=1, "标样核查"=2, "零点核查"=3, "跨度核查"=4, "空白测试"=5, "平行样"=6, "加标回收"=7] ("测量模式(公式)")
            n264 = global write "CODMn断电保存全局变量.vi" "测量模式(公式)"(w540) -> ()
          }
          frame "浮台版" {
            w545 = T9."Enabled" ("禁用")
          }
        }
        n265 = Build Array(w507, w506, w505, w504, w503, w501, w502, w499) -> (w500:refnum<vi>[])
        n266 = Select(t=T9."Enabled" ("禁用"), s=w513, f=T9."Disabled and Grayed Out" ("禁用")) -> (s? t:f=w515:T9)
        n267 = for {
          tunnel: w500 -> [w527] mode=indexing
          tunnel: w498 -> [w526]
          n268 = property class="Ctl"(reference=w527, "DisabledEnum"=w526) -> ()  [unwired: 1 in, 2 out]
        }
        n269 = property on="低切高阈值:" class="DigNum (严格)"("DisabledEnum"=w515) -> ()  [unwired: 2 in, 2 out]
        n270 = property on="高切低阈值:" class="DigNum (严格)"("DisabledEnum"=w515) -> ()  [unwired: 2 in, 2 out]
        n271 = property on="采水泵润洗时间/s:" class="DigNum (严格)"("Visible"=w508) -> ()  [unwired: 2 in, 2 out]
        n272 = property on="采水泵沉淀时间/s:" class="DigNum (严格)"("Visible"=w508) -> ()  [unwired: 2 in, 2 out]
        n273 = property on="采水泵排液时间/s:" class="DigNum (严格)"("Visible"=w508) -> ()  [unwired: 2 in, 2 out]
        n274 = property on="采水泵进样时间/s:" class="DigNum (严格)"("Visible"=w508) -> ()  [unwired: 2 in, 2 out]
        n275 = property on="一键写入" class="Bool (严格)"("DisabledEnum"=w509) -> ()  [unwired: 2 in, 2 out]
        n276 = property on="量程选择" class="Enum (严格)"("Disabled Items []"=w510) -> ()  [unwired: 2 in, 2 out]
        n277 = property on="测量模式(公式)" class="Ring (严格)"("DisabledEnum"=w511) -> ()  [unwired: 2 in, 2 out]
        n278 = property on="氢氧化钠：" class="DigNum (严格)"("Visible"=w496) -> ()  [unwired: 2 in, 2 out]
        n279 = property on="氢氧化钠" class="DigNum (严格)"("Visible"=w496) -> ()  [unwired: 2 in, 2 out]
      }
    }
    n280 = flat-sequence {
      frame #0 {
        # "公式读取显示（只在读取公式的时候改变一次）"
        n281 = global read "COD内部交互全局.vi" "读取公式显示"() -> (w249:bool)
        n282 = case shown="真" w249 {
          frame False {
          }
          frame True {
            n283 = global write "COD内部交互全局.vi" "读取公式显示"(FALSE ("读取参数显示")) -> ()
            n284 = global read "COD内部交互全局.vi" "读取公式"() -> (w259:u16[])
            n285 = Array Subset(array=w259, index=10 ("索引"), length=84 ("长度")) -> (w254:u16[])
            n286 = One Button Dialog(message="公式读取成功！" ("消息")) -> ()  [unwired: 1 in, 1 out]
            n287 = local read "测量模式(公式)"() -> (w257:u16)
            n288 = call "浮点CDAB转换COD.vi"("数组"=w254) -> ("数组 2"=w255:sgl[])  [unwired: 10 in]
            n289 = Array To Cluster(array=w255) -> (cluster=w258:T13)
            n290 = case shown="6" w257 {
              tunnel: [cluster{"X":dbl, "b":dbl, "X^2":dbl} {"X"=999.0, "b"=999.0, "X^2"=999.0} ("方程系数") w262 w281 w300 w319 w338 w357 w376] -> w256
              tunnel: w258 -> [_ w261 w280 w299 w318 w337 w356 w375]
              frame 0, Default {
              }
              frame 1 {
                n291 = local read "量程选择"() -> (w264:enum16{"低量程", "高量程", "0-2量程"})
                n292 = case shown="\"低量程\", 默认" w264 {
                  tunnel: w261 -> [w271 w275 w279]
                  tunnel: [w270 w274 w278] -> w267
                  tunnel: [w269 w273 w277] -> w266
                  tunnel: [w268 w272 w276] -> w265
                  frame "低量程", Default {
                    n293 = Unbundle By Name(w271) -> ("数组 2[0]"=w270:sgl, "数组 2[1]"=w269:sgl, "数组 2[2]"=w268:sgl)
                  }
                  frame "高量程" {
                    n294 = Unbundle By Name(w275) -> ("数组 2[3]"=w274:sgl, "数组 2[4]"=w273:sgl, "数组 2[5]"=w272:sgl)
                  }
                  frame "0-2量程" {
                    n295 = Unbundle By Name(w279) -> ("数组 2[6]"=w278:sgl, "数组 2[7]"=w277:sgl, "数组 2[8]"=w276:sgl)
                  }
                }
                n296 = Bundle By Name(cluster=cluster{"X":dbl, "b":dbl, "X^2":dbl} {"X"=0.0, "b"=0.0, "X^2"=0.0} ("方程系数"), "X"=w267, "b"=w266, "X^2"=w265) -> (w262:cluster{"X":dbl, "b":dbl, "X^2":dbl})
              }
              frame 2 {
                n297 = local read "量程选择"() -> (w283:enum16{"低量程", "高量程", "0-2量程"})
                n298 = case shown="\"高量程\"" w283 {
                  tunnel: w280 -> [w290 w294 w298]
                  tunnel: [w289 w293 w297] -> w286
                  tunnel: [w288 w292 w296] -> w285
                  tunnel: [w287 w291 w295] -> w284
                  frame "低量程", Default {
                    n299 = Unbundle By Name(w290) -> ("数组 2[6]"=w289:sgl, "数组 2[7]"=w288:sgl, "数组 2[8]"=w287:sgl)
                  }
                  frame "高量程" {
                    n300 = Unbundle By Name(w294) -> ("数组 2[9]"=w293:sgl, "数组 2[10]"=w292:sgl, "数组 2[11]"=w291:sgl)
                  }
                  frame "0-2量程" {
                    n301 = Unbundle By Name(w298) -> ("数组 2[6]"=w297:sgl, "数组 2[7]"=w296:sgl, "数组 2[8]"=w295:sgl)
                  }
                }
                n302 = Bundle By Name(cluster=cluster{"X":dbl, "b":dbl, "X^2":dbl} {"X"=0.0, "b"=0.0, "X^2"=0.0} ("方程系数"), "X"=w286, "b"=w285, "X^2"=w284) -> (w281:cluster{"X":dbl, "b":dbl, "X^2":dbl})
              }
              frame 3 {
                n303 = local read "量程选择"() -> (w302:enum16{"低量程", "高量程", "0-2量程"})
                n304 = case shown="\"高量程\"" w302 {
                  tunnel: w299 -> [w309 w313 w317]
                  tunnel: [w308 w312 w316] -> w305
                  tunnel: [w307 w311 w315] -> w304
                  tunnel: [w306 w310 w314] -> w303
                  frame "低量程", Default {
                    n305 = Unbundle By Name(w309) -> ("数组 2[12]"=w308:sgl, "数组 2[13]"=w307:sgl, "数组 2[14]"=w306:sgl)
                  }
                  frame "高量程" {
                    n306 = Unbundle By Name(w313) -> ("数组 2[15]"=w312:sgl, "数组 2[16]"=w311:sgl, "数组 2[17]"=w310:sgl)
                  }
                  frame "0-2量程" {
                    n307 = Unbundle By Name(w317) -> ("数组 2[6]"=w316:sgl, "数组 2[7]"=w315:sgl, "数组 2[8]"=w314:sgl)
                  }
                }
                n308 = Bundle By Name(cluster=cluster{"X":dbl, "b":dbl, "X^2":dbl} {"X"=0.0, "b"=0.0, "X^2"=0.0} ("方程系数"), "X"=w305, "b"=w304, "X^2"=w303) -> (w300:cluster{"X":dbl, "b":dbl, "X^2":dbl})
              }
              frame 4 {
                n309 = local read "量程选择"() -> (w321:enum16{"低量程", "高量程", "0-2量程"})
                n310 = case shown="\"高量程\"" w321 {
                  tunnel: w318 -> [w328 w332 w336]
                  tunnel: [w327 w331 w335] -> w324
                  tunnel: [w326 w330 w334] -> w323
                  tunnel: [w325 w329 w333] -> w322
                  frame "低量程", Default {
                    n311 = Unbundle By Name(w328) -> ("数组 2[18]"=w327:sgl, "数组 2[19]"=w326:sgl, "数组 2[20]"=w325:sgl)
                  }
                  frame "高量程" {
                    n312 = Unbundle By Name(w332) -> ("数组 2[21]"=w331:sgl, "数组 2[22]"=w330:sgl, "数组 2[23]"=w329:sgl)
                  }
                  frame "0-2量程" {
                    n313 = Unbundle By Name(w336) -> ("数组 2[6]"=w335:sgl, "数组 2[7]"=w334:sgl, "数组 2[8]"=w333:sgl)
                  }
                }
                n314 = Bundle By Name(cluster=cluster{"X":dbl, "b":dbl, "X^2":dbl} {"X"=0.0, "b"=0.0, "X^2"=0.0} ("方程系数"), "X"=w324, "b"=w323, "X^2"=w322) -> (w319:cluster{"X":dbl, "b":dbl, "X^2":dbl})
              }
              frame 5 {
                n315 = local read "量程选择"() -> (w340:enum16{"低量程", "高量程", "0-2量程"})
                n316 = case shown="\"高量程\"" w340 {
                  tunnel: w337 -> [w347 w351 w355]
                  tunnel: [w346 w350 w354] -> w343
                  tunnel: [w345 w349 w353] -> w342
                  tunnel: [w344 w348 w352] -> w341
                  frame "低量程", Default {
                    n317 = Unbundle By Name(w347) -> ("数组 2[24]"=w346:sgl, "数组 2[25]"=w345:sgl, "数组 2[26]"=w344:sgl)
                  }
                  frame "高量程" {
                    n318 = Unbundle By Name(w351) -> ("数组 2[27]"=w350:sgl, "数组 2[28]"=w349:sgl, "数组 2[29]"=w348:sgl)
                  }
                  frame "0-2量程" {
                    n319 = Unbundle By Name(w355) -> ("数组 2[6]"=w354:sgl, "数组 2[7]"=w353:sgl, "数组 2[8]"=w352:sgl)
                  }
                }
                n320 = Bundle By Name(cluster=cluster{"X":dbl, "b":dbl, "X^2":dbl} {"X"=0.0, "b"=0.0, "X^2"=0.0} ("方程系数"), "X"=w343, "b"=w342, "X^2"=w341) -> (w338:cluster{"X":dbl, "b":dbl, "X^2":dbl})
              }
              frame 6 {
                n321 = local read "量程选择"() -> (w359:enum16{"低量程", "高量程", "0-2量程"})
                n322 = case shown="\"高量程\"" w359 {
                  tunnel: w356 -> [w366 w370 w374]
                  tunnel: [w365 w369 w373] -> w362
                  tunnel: [w364 w368 w372] -> w361
                  tunnel: [w363 w367 w371] -> w360
                  frame "低量程", Default {
                    n323 = Unbundle By Name(w366) -> ("数组 2[30]"=w365:sgl, "数组 2[31]"=w364:sgl, "数组 2[32]"=w363:sgl)
                  }
                  frame "高量程" {
                    n324 = Unbundle By Name(w370) -> ("数组 2[33]"=w369:sgl, "数组 2[34]"=w368:sgl, "数组 2[35]"=w367:sgl)
                  }
                  frame "0-2量程" {
                    n325 = Unbundle By Name(w374) -> ("数组 2[6]"=w373:sgl, "数组 2[7]"=w372:sgl, "数组 2[8]"=w371:sgl)
                  }
                }
                n326 = Bundle By Name(cluster=cluster{"X":dbl, "b":dbl, "X^2":dbl} {"X"=0.0, "b"=0.0, "X^2"=0.0} ("方程系数"), "X"=w362, "b"=w361, "X^2"=w360) -> (w357:cluster{"X":dbl, "b":dbl, "X^2":dbl})
              }
              frame 7 {
                n327 = local read "量程选择"() -> (w378:enum16{"低量程", "高量程", "0-2量程"})
                n328 = case shown="\"高量程\"" w378 {
                  tunnel: w375 -> [w385 w389 w393]
                  tunnel: [w384 w388 w392] -> w381
                  tunnel: [w383 w387 w391] -> w380
                  tunnel: [w382 w386 w390] -> w379
                  frame "低量程", Default {
                    n329 = Unbundle By Name(w385) -> ("数组 2[36]"=w384:sgl, "数组 2[37]"=w383:sgl, "数组 2[38]"=w382:sgl)
                  }
                  frame "高量程" {
                    n330 = Unbundle By Name(w389) -> ("数组 2[39]"=w388:sgl, "数组 2[40]"=w387:sgl, "数组 2[41]"=w386:sgl)
                  }
                  frame "0-2量程" {
                    n331 = Unbundle By Name(w393) -> ("数组 2[6]"=w392:sgl, "数组 2[7]"=w391:sgl, "数组 2[8]"=w390:sgl)
                  }
                }
                n332 = Bundle By Name(cluster=cluster{"X":dbl, "b":dbl, "X^2":dbl} {"X"=0.0, "b"=0.0, "X^2"=0.0} ("方程系数"), "X"=w381, "b"=w380, "X^2"=w379) -> (w376:cluster{"X":dbl, "b":dbl, "X^2":dbl})
              }
            }
            n333 = local write "方程系数"(w256) -> ()
          }
        }
      }
    }
    n334 = Wait (ms)(milliseconds to wait=u32 1000 ("等待时间（毫秒）")) -> ()  [unwired: 1 out]
  }
  n335 = while {
    tunnel: w15 -> [w558]
    tunnel: w14 -> [w557]
    tunnel: w5 -> [_]
    stop <- FALSE stop-if-true
    # "主循环界面显示"
    n336 = flat-sequence {
      frame #0 {
        # "A，B，K"
        # "CODMn读取状态"
        n337 = global read "COD内部交互全局.vi" "ORP、时间"() -> (w687:u16[])
        n338 = To Word Integer(number=w687) -> (16bit integer=w708:i16[])
        n339 = Split 1D Array(array=w708, index=3 ("索引")) -> (first subarray=w689:i16[], second subarray=w707:i16[])
        n340 = Index Array(array=w689) -> (element #1=w693:i16, element #2=w692:i16, element #3=w691:i16)  [unwired: 3 in]
        n341 = Index Array(array=w707) -> (element #1=w702:i16, element #2=w706:i16, element #3=w705:i16, element #4=w704:i16)  [unwired: 4 in]
        n342 = To Single Precision Float(number=w704) -> (single precision float=w695:sgl)
        n343 = Build Array(w693, w692, w691) -> (w690:i16[])
        n344 = To Single Precision Float(number=w702) -> (single precision float=w701:sgl)
        n345 = To Single Precision Float(number=w706) -> (single precision float=w700:sgl)
        n346 = To Single Precision Float(number=w705) -> (single precision float=w696:sgl)
        n347 = call "HexToDate.vi"("数组"=w690) -> ("DATE"=w694:timestamp[])  [unwired: 10 in]
        n348 = Number To Decimal String(number=w700) -> (decimal integer string=→"ORP-A":string)  [unwired: 1 in]
        n349 = Number To Decimal String(number=w696) -> (decimal integer string=→"ORP-B":string)  [unwired: 1 in]
        n350 = Number To Decimal String(number=w695) -> (decimal integer string=→"ORP-K":string)  [unwired: 1 in]
        n351 = Divide(x=w701, y=sgl 100.0) -> (x/y=→"COD浓度（mg/L)":sgl)
        n352 = Index Array(array=w694) -> (element=w688:timestamp)  [unwired: 1 in]
        n353 = Format Date/Time String(seconds (now)=w688) -> (date/time string=→"数据时间":string)  [unwired: 2 in]
      }
    }
    n354 = flat-sequence {
      frame #0 {
        # "测量状态显示"
        n355 = global read "COD内部交互全局.vi" "测量状态"() -> (w607:u16[])
        n356 = To Word Integer(number=w607) -> (16bit integer=w617:i16[])
        n357 = Index Array(array=w617, index #1=0 ("索引"), index #4=3 ("索引"), index #14=13 ("索引"), index #15=14 ("索引"), index #21=20 ("索引"), index #32=31 ("索引")) -> (element #1=w621:i16, element #2=w620:i16, element #3=w619:i16, element #4=w603:i16, element #5=→"模式（受控）":i16, element #6=→"进样管":i16, element #7=→"高锰酸钾":i16, element #8=→"草酸钠":i16, element #9=→"硫酸":i16, element #10=w616:i16, element #11=w636:i16, element #12=w612:i16, element #13=→"报警数字":i16, element #14=w642:i16, element #15=w627:i16, element #16=→"多列列表框":i16, element #20=→"氢氧化钠":i16, element #21=w600:i16, element #33=→"分":i16, element #34=→"秒":i16)  [unwired: 28 in, 14 out]
        "CODMn工作状态" <- w603
        n358 = global write "COD内部交互全局.vi" "基本量程实时读取"(w600) -> ()
        n359 = Build Array(w621, w620, w619) -> (w622:i16[])
        n360 = To Single Precision Float(number=w616) -> (single precision float=→"实时ORP":sgl)
        n361 = Number To Decimal String(number=w600) -> (decimal integer string=→"基本量程(显示)":string)  [unwired: 1 in]
        n362 = Equal?(x=w612, y=u16 1) -> (x = y?=→"排液标记":bool)
        n363 = Equal?(x=w612, y=u16 2) -> (x = y?=→"断电排液标记":bool)
        n364 = Divide(x=w636, y=u16 10) -> (x/y=→"温度℃":dbl)
        n365 = Divide(x=w642, y=u16 1000) -> (x/y=→"零点滴定值":dbl)
        n366 = Divide(x=w627, y=u16 1000) -> (x/y=→"标度滴定值":dbl)
        n367 = Equal?(x=w603, y=T3."水样测试" ("CODMn工作状态")) -> (x = y?=w601:bool)
        n368 = call "HexToDate.vi"("数组"=w622) -> ("DATE"=w618:timestamp[])  [unwired: 10 in]
        n369 = case shown="真" w601 {
          tunnel: w600 -> [_ w645]
          frame False {
          }
          frame True {
            n370 = global write "CODMn断电保存全局变量.vi" "水样测试量程"(w645) -> ()
          }
        }
        n371 = Index Array(array=w618) -> (element=→"仪器时间":timestamp)  [unwired: 1 in]
      }
    }
    n372 = flat-sequence {
      frame #0 {
        # "报警状态显示"
        n373 = global read "COD内部交互全局.vi" "报警点位"() -> (w660:bool[])
        n374 = Index Array(array=w660, index #1=0 ("索引")) -> (element #1=w657:bool, element #2=w656:bool, element #3=w655:bool, element #4=w654:bool, element #5=w653:bool, element #6=w652:bool, element #7=w651:bool, element #8=w650:bool, element #9=w649:bool, element #11=w648:bool, element #13=w647:bool, element #14=w646:bool)  [unwired: 13 in, 2 out]
        "ORP故障" <- w657
        "温控器故障" <- w656
        "加热故障" <- w649
        "高锰酸钾报警" <- w651
        "草酸钠报警" <- w650
        "测量错误" <- w655
        "校零错误" <- w654
        "校标错误" <- w653
        "进水样超量程" <- w652
        "排液故障" <- w648
        "60分钟超时报警" <- w647
        "进样无液体告警" <- w646
        n375 = Compound Arithmetic op=OR ("复合运算")(w657, w656, w649, w651, w650, w655, w653, w654, w652, w648, w647) -> (→"故障标记":bool)
        n376 = Bundle By Name(cluster=T14 {"ORP故障"=FALSE, "温控器故障"=FALSE, "加热故障"=FALSE, "高锰酸钾报警"=FALSE, "草酸钠报警"=FALSE, "测量错误"=FALSE, "校零错误"=FALSE, "校标错误"=FALSE, " 进水样超量程"=FALSE, "排液阀故障"=FALSE, "60分钟超时报警"=FALSE, "进样无液体报警"=FALSE} ("报警簇"), "ORP故障"=w657, "温控器故障"=w656, "加热故障"=w649, "高锰酸钾报警"=w651, "草酸钠报警"=w650, "测量错误"=w655, "校零错误"=w654, "校标错误"=w653, "进水样超量程"=w652, "排液阀故障"=w648, "60分钟超时报警"=w647, "进样无液体报警"=w646) -> (w658:T14)
        n377 = global write "COD内部交互全局.vi" "报警簇"(w658) -> ()
      }
    }
    n378 = flat-sequence {
      frame #0 {
        # "CODMn读取状态"
        n379 = global read "COD内部交互全局.vi" "温度"() -> (w684:bool[])
        n380 = global read "COD内部交互全局.vi" "M输出点"() -> (w683:bool[])
        n381 = Index Array(array=w684) -> (element=→"加热":bool)  [unwired: 1 in]
        n382 = Index Array(array=w683) -> (element #1=→"搅拌":bool, element #4=→"进水样":bool, element #5=→"进蒸馏水":bool, element #6=→"进标液":bool, element #7=→"进零点核查样":bool, element #8=→"进加标回收样":bool, element #9=→"进高锰酸钾":bool, element #10=→"进草酸钠":bool, element #11=→"进硫酸":bool)  [unwired: 11 in, 2 out]
      }
    }
    n383 = flat-sequence {
      frame #0 {
        # "工作状态显示"
        n384 = local read "CODMn工作状态"() -> (w568:T3)
        n385 = case shown="\"标样校准\"" w568 {
          tunnel: [_ u16 0 ("y") u16 1 ("y") u16 2 ("y") u16 3 ("y") u16 4 ("y") u16 6 ("y") _ u16 7 ("y") u16 8 ("y") u16 5 ("y")] -> w567
          frame "空闲", Default {
          }
          frame "水样测试" {
          }
          frame "标样核查" {
          }
          frame "零点核查" {
          }
          frame "跨度核查" {
          }
          frame "空白测试" {
          }
          frame "平行样测试" {
          }
          frame "质控样" {
          }
          frame "空白校准" {
          }
          frame "标样校准" {
          }
          frame "加标回收" {
          }
        }
        n386 = Equal?(x=w568, y=u16 8) -> (x = y?=→"校零标记":bool)
        n387 = Equal?(x=w568, y=u16 4) -> (x = y?=→"跨度核查标记":bool)
        n388 = Equal?(x=w568, y=u16 0) -> (x = y?=→"待机":bool)
        n389 = Equal?(x=w568, y=u16 3) -> (x = y?=→"零点核查标记":bool)
        n390 = Equal?(x=w568, y=u16 7) -> (x = y?=→"质控样测量":bool)
        n391 = Equal?(x=w568, y=u16 1) -> (x = y?=→"水样测量":bool)
        n392 = Equal?(x=w568, y=u16 2) -> (x = y?=→"标样核查标记":bool)
        n393 = Equal?(x=w568, y=u16 6) -> (x = y?=→"平行样测量":bool)
        n394 = Equal?(x=w568, y=u16 9) -> (x = y?=→"校标标记":bool)
        n395 = Equal?(x=w568, y=u16 5) -> (x = y?=→"空白测试标记":bool)
        n396 = Equal?(x=w568, y=u16 10) -> (x = y?=→"加标回收测量":bool)
        n397 = global write "COD内部交互全局.vi" "测量模式数字"(w567) -> ()
      }
    }
    n398 = Get Date/Time In Seconds() -> (seconds since 1Jan1904=→"系统时间":timestamp)
    n399 = First Call?() -> (First Call?: T/F=w556:bool)
    n400 = Wait (ms)(milliseconds to wait=u32 1000 ("等待时间（毫秒）")) -> ()  [unwired: 1 out]
    n401 = case shown="真" w556 {
      tunnel: w558 -> [w664 w669]
      tunnel: w557 -> [w663 w668]
      tunnel: [w664 w667] -> w554
      tunnel: [w663 w666] -> w553
      frame False {
      }
      frame True {
        n402 = Bundle By Name(cluster=cluster{"命令":string} {"命令"=""} ("元素"), "命令"="CODMn读取参数" ("名称（未命名）")) -> (w672:cluster{"命令":string})
        n403 = Enqueue Element(queue=w669, element=w672, timeout in ms (-1)=1000 ("超时毫秒(-1)"), error in (no error)=w668) -> (queue out=w667:refnum<queue>, error out=w666:errorcluster)  [unwired: 1 out]
      }
    }
    n404 = Get Queue Status(queue=w554, error in (no error)=w553) -> (queue out=w550:refnum<queue>, error out=w549:errorcluster, # elements in queue=w552:i32)  [unwired: 1 in, 5 out]
    n405 = Equal To 0?(x=w552) -> (x = 0?=w551:bool)
    n406 = case shown="真" w551 {
      tunnel: w550 -> [_ w562]
      tunnel: w549 -> [_ w561]
      frame False {
      }
      frame True {
        n407 = Bundle By Name(cluster=cluster{"命令":string} {"命令"=""} ("元素"), "命令"="CODMn读取" ("名称（未命名）")) -> (w564:cluster{"命令":string})
        n408 = Enqueue Element(queue=w562, element=w564, timeout in ms (-1)=1000 ("超时毫秒(-1)"), error in (no error)=w561) -> ()  [unwired: 3 out]
      }
    }
  }
  n409 = while {
    tunnel: w15 -> [w711]
    tunnel: w14 -> [w710]
    stop <- FALSE stop-if-true
    # "主线事件"
    n410 = event shown="[27] \"滴定曲线\", \"温度曲线\": 值改变" {
      selector: _ -> [_ _ _ _ _ _ _ _ _ _ _ _ _ _ _ _ _ _ _ _ _ _ _ _ _ _ _ _ _ _ _ _ _ _]
      dyn-events: _ -> [_ _ _ _ _ _ _ _ _ _ _ _ _ _ _ _ _ _ _ _ _ _ _ _ _ _ _ _ _ _ _ _ _ _]
      timeout: _ -> [_ _ _ _ _ _ _ _ _ _ _ _ _ _ _ _ _ _ _ _ _ _ _ _ _ _ _ _ _ _ _ _ _ _]
      tunnel: w711 -> [_ _ _ _ _ w802 _ _ w835 w940 w1037 _ _ _ _ _ _ _ w1246 _ w1263 _ _ _ w1475 _ _ _ _ w1916 w1923 w1945 w1988 _]
      tunnel: w710 -> [_ _ _ _ _ w801 _ _ w834 w939 w1036 _ _ _ _ _ _ _ w1245 _ w1260 _ _ _ w1474 _ _ _ _ w1915 w1922 w1944 w1987 _]
      event "单步启动": Value Change {
        n411 = event-data() -> ()  [unwired: 1 in, 6 out]
        n412 = call "CODMn手动控制框.vi"() -> ()  [unwired: 12 in]
      }
      event "启动": Mouse Down {
        n413 = event-data() -> ()  [unwired: 1 in, 8 out]
        n414 = global read "COD内部交互全局.vi" "基本量程实时读取"() -> (w715:enum16{"L", "H", "AUTO"})
        n415 = call "启动测量模式选择对话框.vi"("量程选择"=w715) -> ("标样浓度输出"=w713:dbl, "量程选择输出"=w714:enum16{"L", "H", "AUTO"}, "启动选择输出"=w719:u16)  [unwired: 8 in]
        n416 = Not Equal?(x=w719, y=u16 8) -> (x != y?=w716:bool)
        n417 = Not Equal?(x=w719, y=u16 7) -> (x != y?=w717:bool)
        n418 = And(x=w717, y=w716) -> (x .and. y?=w721:bool)
        n419 = case shown="真" w721 {
          tunnel: w719 -> [_ w736]
          tunnel: w714 -> [_ w727]
          tunnel: w713 -> [_ w726]
          frame False {
            n420 = One Button Dialog(message="请到校准配置里面进行校准操作！" ("消息")) -> ()  [unwired: 1 in, 1 out]
          }
          frame True {
            n421 = Not Equal?(x=w736, y=u16 9) -> (x != y?=w731:bool)
            n422 = case shown="\"H\"" w727 {
              tunnel: [w737 w741 errorcluster {"status"=FALSE, "code"=0, "source"=""} ("error out")] -> w725
              frame "L", Default {
                n423 = call "CODMnMB_api.vi"("STEP"=enum16{"open", "read", "write", "close"}."write", "values"=u16[] [0], "starting address"=u16 4276) -> ("error out"=w737:errorcluster)  [unwired: 6 in, 2 out]
              }
              frame "H" {
                n424 = call "CODMnMB_api.vi"("STEP"=enum16{"open", "read", "write", "close"}."write", "values"=u16[] [1], "starting address"=u16 4276) -> ("error out"=w741:errorcluster)  [unwired: 6 in, 2 out]
              }
              frame "AUTO" {
              }
            }
            n425 = global write "CODMN外部API.vi" "手动启动CODMn"(w731) -> ()
            n426 = call "单步测试一键复位.vi"("Error in"=w725) -> ("error out"=w724:errorcluster)  [unwired: 10 in]
            n427 = call <vilib>:"Clear Errors.vi"("error in (no error)"=w724) -> ("error out"=w723:errorcluster)  [unwired: 5 in, 1 out]
            n428 = case shown="0" w736 {
              tunnel: [u16 4608 ("address") u16 4608 ("address") u16 4608 ("address") u16 4608 ("address") u16 4608 ("address") u16 4608 ("address") u16 4608 ("address") u16 4608 ("address") u16 4608 ("address") u16 4608 ("address")] -> w729
              tunnel: [u16 1 ("address") u16 2 ("address") u16 3 ("address") u16 4 ("address") u16 5 ("address") u16 7 ("address") u16 6 ("address") u16 8 ("address") u16 9 ("address") u16 0 ("address")] -> w733
              tunnel: w726 -> [_ w749 _ _ _ _ _ _ _ _]
              frame 0 {
              }
              frame 1 {
                n429 = property on="标样浓度" class="DigNum (严格)"("Val(Sgnl)"=w749) -> ()  [unwired: 2 in, 2 out]
              }
              frame 2 {
              }
              frame 3 {
              }
              frame 4 {
              }
              frame 5 {
              }
              frame 6 {
              }
              frame 7 {
              }
              frame 8 {
              }
              frame 9, Default {
              }
            }
            n430 = Insert Into Array(array=u16[] [] ("values"), index=0 ("索引"), new element=w733) -> (w728:u16[])
            n431 = call "CODMnMB_api.vi"("STEP"=enum16{"open", "read", "write", "close"}."write", "Error in"=w723, "values"=w728, "starting address"=w729) -> ()  [unwired: 5 in, 3 out]
          }
        }
      }
      event "停止": Value Change {
        n432 = event-data() -> ()  [unwired: 1 in, 6 out]
        n433 = Two Button Dialog(message="确认是否停止？" ("消息"), 1:"否" ("F按钮名称（“取消”）"), 2:"是" ("T按钮名称（“确定”）")) -> (T button?=w769:bool)
        n434 = case shown="真" w769 {
          frame False {
          }
          frame True {
            n435 = Obtain Notifier(name (unnamed)="CODMn" ("名称（未命名）"), notification data type=FALSE) -> (notifier out=w775:refnum<notifier>, error out=w773:errorcluster)  [unwired: 2 in, 1 out]
            n436 = Send Notification(notification=TRUE ("通知"), notifier=w775, error in (no error)=w773) -> (notifier out=w772:refnum<notifier>, error out=w771:errorcluster)
            n437 = Release Notifier(notifier=w772, error in (no error)=w771) -> ()  [unwired: 1 in, 3 out]
            n438 = call "CODMnMB_api.vi"("STEP"=enum16{"open", "read", "write", "close"}."write", "values"=u16[] [11], "starting address"=u16 4608) -> ()  [unwired: 6 in, 3 out]
          }
        }
      }
      event "手动控制": Value Change {
        n439 = event-data() -> ()  [unwired: 1 in, 6 out]
        n440 = call "数字密码键盘.vi"() -> ("NewNumber"=w781:sgl)  [unwired: 1 in]
        n441 = Equal?(x=w781, y=8.0) -> (x = y?=w782:bool)
        n442 = case shown="假" w782 {
          frame False {
            n443 = call "窗口弹出对话框(子VI).vi"("消息"="密码错误") -> ()  [unwired: 10 in, 1 out]
          }
          frame True {
          }
        }
      }
      event "锁定按钮": Mouse Down {
        n444 = event-data() -> ("CtlRef"=w787:refnum<vi>)  [unwired: 1 in, 7 out]
        n445 = property class="Bool (严格)"(reference=w787) -> ("Value"=w786:bool)  [unwired: 1 in, 2 out]
        n446 = case shown="真" w786 {
          selector: w786 -> [w788 _]
          tunnel: [w788 w792] -> w785
          frame False {
          }
          frame True {
            n447 = call "数字密码键盘.vi"() -> ("NewNumber"=w789:sgl)  [unwired: 1 in]
            n448 = Equal?(x=w789, y=23506.0) -> (x = y?=w793:bool)
            n449 = Equal?(x=w789, y=8.0) -> (x = y?=w790:bool)
            n450 = Or(x=w793, y=w790) -> (x .or. y?=w792:bool)
            n451 = case shown="假" w792 {
              selector: w792 -> [w796 _]
              frame False {
                n452 = local write "锁定按钮"(w796) -> ()
                n453 = One Button Dialog(message="密码错误!" ("消息")) -> ()  [unwired: 1 in, 1 out]
              }
              frame True {
                n454 = One Button Dialog(message="解锁成功!" ("消息")) -> ()  [unwired: 1 in, 1 out]
              }
            }
          }
        }
        "x = y?" <- w785
      }
      event "参数配置": Value Change {
        (unwired) u16 20 ("number of holding registers")
        (unwired) u16 4272 ("starting address")
        n455 = event-data() -> ()  [unwired: 1 in, 6 out]
        n456 = global read "CODMN外部API.vi" "ping"() -> (w800:bool)
        n457 = property on="窗格" class="Pane"("Origin"=T4 {"Horizontal"=0, "Vertical"=650} ("原点")) -> ()  [unwired: 2 in, 2 out]
        n458 = case shown="假" w800 {
          tunnel: [w812 w815] -> w799
          frame False {
            n459 = global read "COD内部交互全局.vi" "配置文件ini"() -> (w814:string)
            n460 = call <vilib>:"Application Directory.vi"() -> ("Application Directory"=w813:path)
            n461 = Build Path(base path=w813, name or relative path=w814) -> (appended path=w812:path)
          }
          frame True {
            n462 = global read "CODMN外部API.vi" "配置文件 path"() -> (w815:path)
          }
        }
        n463 = Bundle By Name(cluster=cluster{"命令":string} {"命令"=""} ("元素"), "命令"="CODMn读取参数" ("名称（未命名）")) -> (w803:cluster{"命令":string})
        n464 = call <vilib>:"Open Config Data.vi"("configuration file path"=w799) -> ("error out"=w809:errorcluster, "refnum"=w806:T6)  [unwired: 8 in, 1 out]
        n465 = Enqueue Element(queue=w802, element=w803, error in (no error)=w801) -> ()  [unwired: 1 in, 3 out]
        n466 = vi-ref "斯坦道CODMn.lvlib:CODMn断电保存全局变量.vi"() -> (w807:refnum<vi>)
        n467 = call <userlib>:"Read Panel from INI__ogtk.vi"("error in (no error)"=w809, "VI ref"=w807, "refnum"=w806) -> ("error out"=w810:errorcluster, "refnum out"=w808:T6)  [unwired: 7 in]
        n468 = call <vilib>:"Close Config Data.vi"("error in (no error)"=w810, "refnum"=w808) -> ("error out"=w798:errorcluster)  [unwired: 8 in, 1 out]
        n469 = call <vilib>:"Clear Errors.vi"("error in (no error)"=w798) -> ()  [unwired: 5 in, 2 out]
      }
      event "保存": Mouse Down {
        n470 = event-data() -> ()  [unwired: 1 in, 8 out]
        n471 = local read "通讯状态"() -> (w816:bool)
        n472 = Two Button Dialog(message="确定保存参数，保存参数将会替换原有参数！" ("消息")) -> (T button?=w818:bool)  [unwired: 2 in]
        n473 = case shown="真" w818 {
          tunnel: w816 -> [_ w819]
          frame False {
          }
          frame True {
            n474 = case shown="真" w819 {
              frame False {
                n475 = One Button Dialog(message="保存失败，当前无通讯！" ("消息")) -> ()  [unwired: 1 in, 1 out]
              }
              frame True {
                n476 = One Button Dialog(message="参数保存成功！" ("消息")) -> ()  [unwired: 1 in, 1 out]
                n477 = Build Array("采水泵进样时间/s:", "采水泵润洗时间/s:", "采水泵沉淀时间/s:", "采水泵排液时间/s:") -> (w822:i32[])
                n478 = call "CODMnMB_api.vi"("STEP"=enum16{"open", "read", "write", "close"}."write", "values"="保存参数", "starting address"=u16 4272) -> ("error out"=w828:errorcluster)  [unwired: 6 in, 2 out]
                n479 = call "CODMnMB_api.vi"("STEP"=enum16{"open", "read", "write", "close"}."write", "Error in"=w828, "values"=w822, "starting address"=u16 5596) -> ()  [unwired: 5 in, 3 out]
              }
            }
          }
        }
      }
      event "常规版/认证版": Value Change {
        n480 = event-data() -> ()  [unwired: 1 in, 6 out]
        n481 = flat-sequence {
          frame #0 {
            n482 = global write "CODMn断电保存全局变量.vi" "常规版/认证版"("常规版/认证版") -> ()
          }
          frame #1 {
            n483 = call "配置文件保存.vi"() -> ()  [unwired: 12 in]
          }
        }
      }
      event "校准配置": Value Change {
        w848 = "量程选择" ("section")
        n484 = event-data() -> ()  [unwired: 1 in, 6 out]
        n485 = global read "CODMN外部API.vi" "ping"() -> (w852:bool)
        n486 = property on="窗格" class="Pane"("Origin"=T4 {"Horizontal"=0, "Vertical"=1300} ("原点")) -> ()  [unwired: 2 in, 2 out]
        n487 = case shown="假" w852 {
          tunnel: [w930 w933] -> w851
          frame False {
            n488 = global read "COD内部交互全局.vi" "配置文件ini"() -> (w932:string)
            n489 = call <vilib>:"Application Directory.vi"() -> ("Application Directory"=w931:path)
            n490 = Build Path(base path=w931, name or relative path=w932) -> (appended path=w930:path)
          }
          frame True {
            n491 = global read "CODMN外部API.vi" "配置文件 path"() -> (w933:path)
          }
        }
        n492 = Bundle By Name(cluster=cluster{"命令":string} {"命令"=""} ("元素"), "命令"="CODMn读取公式" ("名称（未命名）")) -> (w836:cluster{"命令":string})
        n493 = Enqueue Element(queue=w835, element=w836, error in (no error)=w834) -> ()  [unwired: 1 in, 3 out]
        n494 = call <vilib>:"Open Config Data.vi"("configuration file path"=w851) -> ("error out"=w869:errorcluster, "refnum"=w870:T6)  [unwired: 8 in, 1 out]
        n495 = call-poly <vilib>:"Read Key.vi"("section"="CODMn模型选择" ("key"), "error in (no error)"=w869, "key"="线性和多项式", "refnum"=w870) -> ("error out"=w866:errorcluster, "value"=w868:i32, "refnum out"=w867:T6)  [unwired: 4 in, 1 out]
        n496 = local write "模型"(w868) -> ()
        n497 = call-poly <vilib>:"Read Key.vi"("section"="标线选择", "error in (no error)"=w866, "key"="选用水样", "refnum"=w867) -> ("error out"=w849:errorcluster, "value"=w853:i32, "refnum out"=w850:T6)  [unwired: 4 in, 1 out]
        n498 = local write "选用水样"(w853) -> ()
        n499 = case shown="0, 默认" w853 {
          tunnel: ["葡萄糖标线" ("section") "草酸钠标线" ("section")] -> w875
          frame 0, Default {
          }
          frame 1 {
          }
        }
        n500 = call-poly <vilib>:"Read Key.vi"("section"=w848, "error in (no error)"=w849, "key"=w848, "refnum"=w850) -> ("error out"=w846:errorcluster, "value"=w845:i32, "refnum out"=w847:T6)  [unwired: 4 in, 1 out]
        n501 = local write "量程选择"(w845) -> ()
        n502 = case shown="2" w845 {
          tunnel: ["低量程" "高量程" "0-2量程"] -> w874
          frame 0, Default {
          }
          frame 1 {
          }
          frame 2 {
          }
        }
        n503 = Concatenate Strings(w875, w874) -> (w873:string)
        n504 = call-poly <vilib>:"Read Key.vi"("section"=w873, "error in (no error)"=w846, "key"="浓度1", "refnum"=w847) -> ("error out"=w900:errorcluster, "value"=w898:dbl, "refnum out"=w899:T6)  [unwired: 4 in, 1 out]
        n505 = local write "浓度1"(w898) -> ()
        n506 = call-poly <vilib>:"Read Key.vi"("section"=w873, "error in (no error)"=w900, "key"="浓度2", "refnum"=w899) -> ("error out"=w914:errorcluster, "value"=w901:dbl, "refnum out"=w913:T6)  [unwired: 4 in, 1 out]
        n507 = local write "浓度2"(w901) -> ()
        n508 = call-poly <vilib>:"Read Key.vi"("section"=w873, "error in (no error)"=w914, "key"="浓度3", "refnum"=w913) -> ("error out"=w915:errorcluster, "value"=w903:dbl, "refnum out"=w912:T6)  [unwired: 4 in, 1 out]
        n509 = local write "浓度3"(w903) -> ()
        n510 = call-poly <vilib>:"Read Key.vi"("section"=w873, "error in (no error)"=w915, "key"="泵滴定数1", "refnum"=w912) -> ("error out"=w916:errorcluster, "value"=w905:dbl, "refnum out"=w911:T6)  [unwired: 4 in, 1 out]
        n511 = local write "泵滴定数1"(w905) -> ()
        n512 = call-poly <vilib>:"Read Key.vi"("section"=w873, "error in (no error)"=w916, "key"="泵滴定数2", "refnum"=w911) -> ("error out"=w910:errorcluster, "value"=w908:dbl, "refnum out"=w917:T6)  [unwired: 4 in, 1 out]
        n513 = local write "泵滴定数2"(w908) -> ()
        n514 = call-poly <vilib>:"Read Key.vi"("section"=w873, "error in (no error)"=w910, "key"="泵滴定数3", "refnum"=w917) -> ("error out"=w922:errorcluster, "value"=w921:dbl, "refnum out"=w918:T6)  [unwired: 4 in, 1 out]
        n515 = local write "泵滴定数3"(w921) -> ()
        n516 = call-poly <vilib>:"Read Key.vi"("section"=w873, "error in (no error)"=w922, "key"="浓度4", "refnum"=w918) -> ("error out"=w923:errorcluster, "value"=w859:dbl, "refnum out"=w919:T6)  [unwired: 4 in, 1 out]
        n517 = local write "浓度4"(w859) -> ()
        n518 = call-poly <vilib>:"Read Key.vi"("section"=w873, "error in (no error)"=w923, "key"="浓度5", "refnum"=w919) -> ("error out"=w864:errorcluster, "value"=w858:dbl, "refnum out"=w865:T6)  [unwired: 4 in, 1 out]
        n519 = local write "浓度5"(w858) -> ()
        n520 = call-poly <vilib>:"Read Key.vi"("section"=w873, "error in (no error)"=w864, "key"="泵滴定数4", "refnum"=w865) -> ("error out"=w924:errorcluster, "value"=w857:dbl, "refnum out"=w920:T6)  [unwired: 4 in, 1 out]
        n521 = local write "泵滴定数4"(w857) -> ()
        n522 = call-poly <vilib>:"Read Key.vi"("section"=w873, "error in (no error)"=w924, "key"="泵滴定数5", "refnum"=w920) -> ("error out"=w862:errorcluster, "value"=w856:dbl, "refnum out"=w863:T6)  [unwired: 4 in, 1 out]
        n523 = local write "泵滴定数5"(w856) -> ()
        n524 = call-poly <vilib>:"Read Key.vi"("section"=w873, "error in (no error)"=w862, "key"="当前选用的校准", "refnum"=w863) -> ("error out"=w894:errorcluster, "refnum out"=w895:T6)  [unwired: 4 in, 2 out]
        n525 = call-poly <vilib>:"Read Key.vi"("section"=w873, "error in (no error)"=w894, "key"="启用1", "refnum"=w895) -> ("error out"=w891:errorcluster, "value"=w880:bool, "refnum out"=w892:T6)  [unwired: 4 in, 1 out]
        n526 = local write "启用1"(w880) -> ()
        n527 = call-poly <vilib>:"Read Key.vi"("section"=w873, "error in (no error)"=w891, "key"="启用2", "refnum"=w892) -> ("error out"=w889:errorcluster, "value"=w879:bool, "refnum out"=w890:T6)  [unwired: 4 in, 1 out]
        n528 = local write "启用2"(w879) -> ()
        n529 = call-poly <vilib>:"Read Key.vi"("section"=w873, "error in (no error)"=w889, "key"="启用3", "refnum"=w890) -> ("error out"=w887:errorcluster, "value"=w878:bool, "refnum out"=w888:T6)  [unwired: 4 in, 1 out]
        n530 = local write "启用3"(w878) -> ()
        n531 = call-poly <vilib>:"Read Key.vi"("section"=w873, "error in (no error)"=w887, "key"="启用4", "refnum"=w888) -> ("error out"=w885:errorcluster, "value"=w855:bool, "refnum out"=w886:T6)  [unwired: 4 in, 1 out]
        n532 = local write "启用4"(w855) -> ()
        n533 = call-poly <vilib>:"Read Key.vi"("section"=w873, "error in (no error)"=w885, "key"="启用5", "refnum"=w886) -> ("error out"=w860:errorcluster, "value"=w854:bool, "refnum out"=w861:T6)  [unwired: 4 in, 1 out]
        n534 = local write "启用5"(w854) -> ()
        n535 = call <vilib>:"Close Config Data.vi"("error in (no error)"=w860, "refnum"=w861) -> ("error out"=w839:errorcluster, "file path"=w840:path)  [unwired: 8 in]
        n536 = Open/Create/Replace File(file path (use dialog)=w840, error in=w839) -> (refnum out=w842:refnum<file>, error out=w841:errorcluster)  [unwired: 4 in, 1 out]
        n537 = Flush File(refnum=w842, error in=w841) -> (refnum out=w843:refnum<file>, error out=w844:errorcluster)
        n538 = Close File(refnum=w843, error in=w844) -> ()  [unwired: 2 out]
      }
      event "选用水样": Value Change {
        (unwired) "浓度6" ("key")
        n539 = event-data() -> ()  [unwired: 1 in, 6 out]
        n540 = local read "量程选择"() -> (w972:enum16{"低量程", "高量程", "0-2量程"})
        n541 = property on="窗格" class="Pane"("Origin"=T4 {"Horizontal"=0, "Vertical"=1300} ("原点")) -> ()  [unwired: 2 in, 2 out]
        n542 = case shown="\"葡萄糖\", 默认" "选用水样" {
          tunnel: ["葡萄糖标线" ("section") "草酸钠标线" ("section")] -> w974
          frame "葡萄糖", Default {
          }
          frame "草酸钠" {
          }
        }
        n543 = global read "CODMN外部API.vi" "ping"() -> (w958:bool)
        n544 = case shown="\"0-2量程\"" w972 {
          tunnel: ["低量程" "高量程" "0-2量程"] -> w973
          frame "低量程", Default {
          }
          frame "高量程" {
          }
          frame "0-2量程" {
          }
        }
        n545 = case shown="假" w958 {
          tunnel: [w1027 w1030] -> w957
          frame False {
            n546 = global read "COD内部交互全局.vi" "配置文件ini"() -> (w1029:string)
            n547 = call <vilib>:"Application Directory.vi"() -> ("Application Directory"=w1028:path)
            n548 = Build Path(base path=w1028, name or relative path=w1029) -> (appended path=w1027:path)
          }
          frame True {
            n549 = global read "CODMN外部API.vi" "配置文件 path"() -> (w1030:path)
          }
        }
        n550 = Concatenate Strings(w974, w973) -> (w971:string)
        n551 = call <vilib>:"Open Config Data.vi"("configuration file path"=w957) -> ("error out"=w953:errorcluster, "refnum"=w954:T6)  [unwired: 8 in, 1 out]
        n552 = Bundle By Name(cluster=cluster{"命令":string} {"命令"=""} ("元素"), "命令"="CODMn读取公式" ("名称（未命名）")) -> (w941:cluster{"命令":string})
        n553 = call-poly <vilib>:"Write Key.vi"("section"="标线选择", "error in (no error)"=w953, "value"="选用水样", "key"="选用水样", "refnum"=w954) -> ("error out"=w950:errorcluster, "refnum out"=w951:T6)  [unwired: 4 in, 1 out]
        n554 = call-poly <vilib>:"Read Key.vi"("section"=w971, "error in (no error)"=w950, "key"="浓度1", "refnum"=w951) -> ("error out"=w997:errorcluster, "value"=w995:dbl, "refnum out"=w996:T6)  [unwired: 4 in, 1 out]
        n555 = Enqueue Element(queue=w940, element=w941, error in (no error)=w939) -> ()  [unwired: 1 in, 3 out]
        n556 = local write "浓度1"(w995) -> ()
        n557 = call-poly <vilib>:"Read Key.vi"("section"=w971, "error in (no error)"=w997, "key"="浓度2", "refnum"=w996) -> ("error out"=w1011:errorcluster, "value"=w998:dbl, "refnum out"=w1010:T6)  [unwired: 4 in, 1 out]
        n558 = local write "浓度2"(w998) -> ()
        n559 = call-poly <vilib>:"Read Key.vi"("section"=w971, "error in (no error)"=w1011, "key"="浓度3", "refnum"=w1010) -> ("error out"=w1012:errorcluster, "value"=w1000:dbl, "refnum out"=w1009:T6)  [unwired: 4 in, 1 out]
        n560 = local write "浓度3"(w1000) -> ()
        n561 = call-poly <vilib>:"Read Key.vi"("section"=w971, "error in (no error)"=w1012, "key"="泵滴定数1", "refnum"=w1009) -> ("error out"=w1013:errorcluster, "value"=w1002:dbl, "refnum out"=w1008:T6)  [unwired: 4 in, 1 out]
        n562 = local write "泵滴定数1"(w1002) -> ()
        n563 = call-poly <vilib>:"Read Key.vi"("section"=w971, "error in (no error)"=w1013, "key"="泵滴定数2", "refnum"=w1008) -> ("error out"=w1007:errorcluster, "value"=w1005:dbl, "refnum out"=w1014:T6)  [unwired: 4 in, 1 out]
        n564 = local write "泵滴定数2"(w1005) -> ()
        n565 = call-poly <vilib>:"Read Key.vi"("section"=w971, "error in (no error)"=w1007, "key"="泵滴定数3", "refnum"=w1014) -> ("error out"=w1019:errorcluster, "value"=w1018:dbl, "refnum out"=w1015:T6)  [unwired: 4 in, 1 out]
        n566 = local write "泵滴定数3"(w1018) -> ()
        n567 = call-poly <vilib>:"Read Key.vi"("section"=w971, "error in (no error)"=w1019, "key"="浓度4", "refnum"=w1015) -> ("error out"=w1020:errorcluster, "value"=w966:dbl, "refnum out"=w1016:T6)  [unwired: 4 in, 1 out]
        n568 = local write "浓度4"(w966) -> ()
        n569 = call-poly <vilib>:"Read Key.vi"("section"=w971, "error in (no error)"=w1020, "key"="浓度5", "refnum"=w1016) -> ("error out"=w969:errorcluster, "value"=w965:dbl, "refnum out"=w970:T6)  [unwired: 4 in, 1 out]
        n570 = local write "浓度5"(w965) -> ()
        n571 = call-poly <vilib>:"Read Key.vi"("section"=w971, "error in (no error)"=w969, "key"="泵滴定数4", "refnum"=w970) -> ("error out"=w1021:errorcluster, "value"=w964:dbl, "refnum out"=w1017:T6)  [unwired: 4 in, 1 out]
        n572 = local write "泵滴定数4"(w964) -> ()
        n573 = call-poly <vilib>:"Read Key.vi"("section"=w971, "error in (no error)"=w1021, "key"="泵滴定数5", "refnum"=w1017) -> ("error out"=w967:errorcluster, "value"=w963:dbl, "refnum out"=w968:T6)  [unwired: 4 in, 1 out]
        n574 = local write "泵滴定数5"(w963) -> ()
        n575 = call-poly <vilib>:"Read Key.vi"("section"=w971, "error in (no error)"=w967, "key"="当前选用的校准", "refnum"=w968) -> ("error out"=w991:errorcluster, "refnum out"=w992:T6)  [unwired: 4 in, 2 out]
        n576 = call-poly <vilib>:"Read Key.vi"("section"=w971, "error in (no error)"=w991, "key"="启用1", "refnum"=w992) -> ("error out"=w988:errorcluster, "value"=w977:bool, "refnum out"=w989:T6)  [unwired: 4 in, 1 out]
        n577 = local write "启用1"(w977) -> ()
        n578 = call-poly <vilib>:"Read Key.vi"("section"=w971, "error in (no error)"=w988, "key"="启用2", "refnum"=w989) -> ("error out"=w986:errorcluster, "value"=w976:bool, "refnum out"=w987:T6)  [unwired: 4 in, 1 out]
        n579 = local write "启用2"(w976) -> ()
        n580 = call-poly <vilib>:"Read Key.vi"("section"=w971, "error in (no error)"=w986, "key"="启用3", "refnum"=w987) -> ("error out"=w984:errorcluster, "value"=w975:bool, "refnum out"=w985:T6)  [unwired: 4 in, 1 out]
        n581 = local write "启用3"(w975) -> ()
        n582 = call-poly <vilib>:"Read Key.vi"("section"=w971, "error in (no error)"=w984, "key"="启用4", "refnum"=w985) -> ("error out"=w982:errorcluster, "value"=w960:bool, "refnum out"=w983:T6)  [unwired: 4 in, 1 out]
        n583 = local write "启用4"(w960) -> ()
        n584 = call-poly <vilib>:"Read Key.vi"("section"=w971, "error in (no error)"=w982, "key"="启用5", "refnum"=w983) -> ("error out"=w961:errorcluster, "value"=w959:bool, "refnum out"=w962:T6)  [unwired: 4 in, 1 out]
        n585 = local write "启用5"(w959) -> ()
        n586 = call <vilib>:"Close Config Data.vi"("error in (no error)"=w961, "refnum"=w962) -> ("error out"=w944:errorcluster, "file path"=w945:path)  [unwired: 8 in]
        n587 = Open/Create/Replace File(file path (use dialog)=w945, error in=w944) -> (refnum out=w947:refnum<file>, error out=w946:errorcluster)  [unwired: 4 in, 1 out]
        n588 = Flush File(refnum=w947, error in=w946) -> (refnum out=w948:refnum<file>, error out=w949:errorcluster)
        n589 = Close File(refnum=w948, error in=w949) -> ()  [unwired: 2 out]
      }
      event "量程选择": Value Change {
        w1052 = "量程选择" ("section")
        n590 = event-data() -> ()  [unwired: 1 in, 6 out]
        n591 = local read "选用水样"() -> (w1070:enum16{"葡萄糖", "草酸钠"})
        n592 = property on="窗格" class="Pane"("Origin"=T4 {"Horizontal"=0, "Vertical"=1300} ("原点")) -> ()  [unwired: 2 in, 2 out]
        n593 = Bundle By Name(cluster=cluster{"命令":string} {"命令"=""} ("元素"), "命令"="CODMn读取公式" ("名称（未命名）")) -> (w1038:cluster{"命令":string})
        n594 = case shown="\"葡萄糖\", 默认" w1070 {
          tunnel: ["葡萄糖标线" ("section") "草酸钠标线" ("section")] -> w1069
          frame "葡萄糖", Default {
          }
          frame "草酸钠" {
          }
        }
        n595 = global read "CODMN外部API.vi" "ping"() -> (w1054:bool)
        n596 = case shown="\"0-2量程\"" "量程选择" {
          tunnel: ["低量程" "高量程" "0-2量程"] -> w1067
          frame "低量程", Default {
          }
          frame "高量程" {
          }
          frame "0-2量程" {
          }
        }
        n597 = Enqueue Element(queue=w1037, element=w1038, error in (no error)=w1036) -> ()  [unwired: 1 in, 3 out]
        n598 = case shown="假" w1054 {
          tunnel: [w1123 w1126] -> w1053
          frame False {
            n599 = global read "COD内部交互全局.vi" "配置文件ini"() -> (w1125:string)
            n600 = call <vilib>:"Application Directory.vi"() -> ("Application Directory"=w1124:path)
            n601 = Build Path(base path=w1124, name or relative path=w1125) -> (appended path=w1123:path)
          }
          frame True {
            n602 = global read "CODMN外部API.vi" "配置文件 path"() -> (w1126:path)
          }
        }
        n603 = Concatenate Strings(w1069, w1067) -> (w1068:string)
        n604 = call <vilib>:"Open Config Data.vi"("configuration file path"=w1053) -> ("error out"=w1051:errorcluster, "refnum"=w1050:T6)  [unwired: 8 in, 1 out]
        n605 = call-poly <vilib>:"Write Key.vi"("section"=w1052, "error in (no error)"=w1051, "value"="量程选择", "key"=w1052, "refnum"=w1050) -> ("error out"=w1047:errorcluster, "refnum out"=w1049:T6)  [unwired: 4 in, 1 out]
        n606 = call-poly <vilib>:"Read Key.vi"("section"=w1068, "error in (no error)"=w1047, "key"="浓度1", "refnum"=w1049) -> ("error out"=w1093:errorcluster, "value"=w1091:dbl, "refnum out"=w1092:T6)  [unwired: 4 in, 1 out]
        n607 = local write "浓度1"(w1091) -> ()
        n608 = call-poly <vilib>:"Read Key.vi"("section"=w1068, "error in (no error)"=w1093, "key"="浓度2", "refnum"=w1092) -> ("error out"=w1107:errorcluster, "value"=w1094:dbl, "refnum out"=w1106:T6)  [unwired: 4 in, 1 out]
        n609 = local write "浓度2"(w1094) -> ()
        n610 = call-poly <vilib>:"Read Key.vi"("section"=w1068, "error in (no error)"=w1107, "key"="浓度3", "refnum"=w1106) -> ("error out"=w1108:errorcluster, "value"=w1096:dbl, "refnum out"=w1105:T6)  [unwired: 4 in, 1 out]
        n611 = local write "浓度3"(w1096) -> ()
        n612 = call-poly <vilib>:"Read Key.vi"("section"=w1068, "error in (no error)"=w1108, "key"="泵滴定数1", "refnum"=w1105) -> ("error out"=w1109:errorcluster, "value"=w1098:dbl, "refnum out"=w1104:T6)  [unwired: 4 in, 1 out]
        n613 = local write "泵滴定数1"(w1098) -> ()
        n614 = call-poly <vilib>:"Read Key.vi"("section"=w1068, "error in (no error)"=w1109, "key"="泵滴定数2", "refnum"=w1104) -> ("error out"=w1103:errorcluster, "value"=w1101:dbl, "refnum out"=w1110:T6)  [unwired: 4 in, 1 out]
        n615 = local write "泵滴定数2"(w1101) -> ()
        n616 = call-poly <vilib>:"Read Key.vi"("section"=w1068, "error in (no error)"=w1103, "key"="泵滴定数3", "refnum"=w1110) -> ("error out"=w1115:errorcluster, "value"=w1114:dbl, "refnum out"=w1111:T6)  [unwired: 4 in, 1 out]
        n617 = local write "泵滴定数3"(w1114) -> ()
        n618 = call-poly <vilib>:"Read Key.vi"("section"=w1068, "error in (no error)"=w1115, "key"="浓度4", "refnum"=w1111) -> ("error out"=w1116:errorcluster, "value"=w1058:dbl, "refnum out"=w1112:T6)  [unwired: 4 in, 1 out]
        n619 = local write "浓度4"(w1058) -> ()
        n620 = call-poly <vilib>:"Read Key.vi"("section"=w1068, "error in (no error)"=w1116, "key"="浓度5", "refnum"=w1112) -> ("error out"=w1065:errorcluster, "value"=w1057:dbl, "refnum out"=w1066:T6)  [unwired: 4 in, 1 out]
        n621 = local write "浓度5"(w1057) -> ()
        n622 = call-poly <vilib>:"Read Key.vi"("section"=w1068, "error in (no error)"=w1065, "key"="泵滴定数4", "refnum"=w1066) -> ("error out"=w1117:errorcluster, "value"=w1056:dbl, "refnum out"=w1113:T6)  [unwired: 4 in, 1 out]
        n623 = local write "泵滴定数4"(w1056) -> ()
        n624 = call-poly <vilib>:"Read Key.vi"("section"=w1068, "error in (no error)"=w1117, "key"="泵滴定数5", "refnum"=w1113) -> ("error out"=w1063:errorcluster, "value"=w1055:dbl, "refnum out"=w1064:T6)  [unwired: 4 in, 1 out]
        n625 = local write "泵滴定数5"(w1055) -> ()
        n626 = call-poly <vilib>:"Read Key.vi"("section"=w1068, "error in (no error)"=w1063, "key"="当前选用的校准", "refnum"=w1064) -> ("error out"=w1087:errorcluster, "refnum out"=w1088:T6)  [unwired: 4 in, 2 out]
        n627 = call-poly <vilib>:"Read Key.vi"("section"=w1068, "error in (no error)"=w1087, "key"="启用1", "refnum"=w1088) -> ("error out"=w1084:errorcluster, "value"=w1073:bool, "refnum out"=w1085:T6)  [unwired: 4 in, 1 out]
        n628 = local write "启用1"(w1073) -> ()
        n629 = call-poly <vilib>:"Read Key.vi"("section"=w1068, "error in (no error)"=w1084, "key"="启用2", "refnum"=w1085) -> ("error out"=w1082:errorcluster, "value"=w1072:bool, "refnum out"=w1083:T6)  [unwired: 4 in, 1 out]
        n630 = local write "启用2"(w1072) -> ()
        n631 = call-poly <vilib>:"Read Key.vi"("section"=w1068, "error in (no error)"=w1082, "key"="启用3", "refnum"=w1083) -> ("error out"=w1080:errorcluster, "value"=w1071:bool, "refnum out"=w1081:T6)  [unwired: 4 in, 1 out]
        n632 = local write "启用3"(w1071) -> ()
        n633 = call-poly <vilib>:"Read Key.vi"("section"=w1068, "error in (no error)"=w1080, "key"="启用4", "refnum"=w1081) -> ("error out"=w1078:errorcluster, "value"=w1060:bool, "refnum out"=w1079:T6)  [unwired: 4 in, 1 out]
        n634 = local write "启用4"(w1060) -> ()
        n635 = call-poly <vilib>:"Read Key.vi"("section"=w1068, "error in (no error)"=w1078, "key"="启用5", "refnum"=w1079) -> ("error out"=w1061:errorcluster, "value"=w1059:bool, "refnum out"=w1062:T6)  [unwired: 4 in, 1 out]
        n636 = local write "启用5"(w1059) -> ()
        n637 = call <vilib>:"Close Config Data.vi"("error in (no error)"=w1061, "refnum"=w1062) -> ("error out"=w1041:errorcluster, "file path"=w1042:path)  [unwired: 8 in]
        n638 = Open/Create/Replace File(file path (use dialog)=w1042, error in=w1041) -> (refnum out=w1044:refnum<file>, error out=w1043:errorcluster)  [unwired: 4 in, 1 out]
        n639 = Flush File(refnum=w1044, error in=w1043) -> (refnum out=w1045:refnum<file>, error out=w1046:errorcluster)
        n640 = Close File(refnum=w1045, error in=w1046) -> ()  [unwired: 2 out]
      }
      event "返回": Value Change {
        w1153 = "CODMn" ("section")
        n641 = event-data() -> ()  [unwired: 1 in, 6 out]
        n642 = property on="窗格" class="Pane"("Origin"=T4 {"Horizontal"=0, "Vertical"=0} ("原点")) -> ()  [unwired: 2 in, 2 out]
        n643 = global read "CODMN外部API.vi" "ping"() -> (w1139:bool)
        n644 = case shown="假" w1139 {
          tunnel: [w1204 w1207] -> w1138
          frame False {
            n645 = global read "COD内部交互全局.vi" "配置文件ini"() -> (w1206:string)
            n646 = call <vilib>:"Application Directory.vi"() -> ("Application Directory"=w1205:path)
            n647 = Build Path(base path=w1205, name or relative path=w1206) -> (appended path=w1204:path)
          }
          frame True {
            n648 = global read "CODMN外部API.vi" "配置文件 path"() -> (w1207:path)
          }
        }
        n649 = call <vilib>:"Open Config Data.vi"("configuration file path"=w1138) -> ("error out"=w1202:errorcluster, "refnum"=w1203:T6)  [unwired: 8 in, 1 out]
        n650 = local read "浓度1"() -> (w1200:dbl)
        n651 = call-poly <vilib>:"Write Key.vi"("section"=w1153, "error in (no error)"=w1202, "value"=w1200, "key"="浓度1", "refnum"=w1203) -> ("error out"=w1199:errorcluster, "refnum out"=w1198:T6)  [unwired: 4 in, 1 out]
        n652 = local read "浓度2"() -> (w1184:dbl)
        n653 = call-poly <vilib>:"Write Key.vi"("section"=w1153, "error in (no error)"=w1199, "value"=w1184, "key"="浓度2", "refnum"=w1198) -> ("error out"=w1197:errorcluster, "refnum out"=w1196:T6)  [unwired: 4 in, 1 out]
        n654 = local read "浓度3"() -> (w1180:dbl)
        n655 = local read "泵滴定数1"() -> (w1178:dbl)
        n656 = call-poly <vilib>:"Write Key.vi"("section"=w1153, "error in (no error)"=w1197, "value"=w1180, "key"="浓度3", "refnum"=w1196) -> ("error out"=w1195:errorcluster, "refnum out"=w1194:T6)  [unwired: 4 in, 1 out]
        n657 = local read "泵滴定数2"() -> (w1176:dbl)
        n658 = call-poly <vilib>:"Write Key.vi"("section"=w1153, "error in (no error)"=w1195, "value"=w1178, "key"="泵滴定数1", "refnum"=w1194) -> ("error out"=w1193:errorcluster, "refnum out"=w1192:T6)  [unwired: 4 in, 1 out]
        n659 = local read "泵滴定数3"() -> (w1174:dbl)
        n660 = call-poly <vilib>:"Write Key.vi"("section"=w1153, "error in (no error)"=w1193, "value"=w1176, "key"="泵滴定数2", "refnum"=w1192) -> ("error out"=w1191:errorcluster, "refnum out"=w1190:T6)  [unwired: 4 in, 1 out]
        n661 = call-poly <vilib>:"Write Key.vi"("section"=w1153, "error in (no error)"=w1191, "value"=w1174, "key"="泵滴定数3", "refnum"=w1190) -> ("error out"=w1189:errorcluster, "refnum out"=w1188:T6)  [unwired: 4 in, 1 out]
        n662 = local read "浓度4"() -> (w1141:dbl)
        n663 = call-poly <vilib>:"Write Key.vi"("section"=w1153, "error in (no error)"=w1189, "value"=w1141, "key"="浓度4", "refnum"=w1188) -> ("error out"=w1182:errorcluster, "refnum out"=w1183:T6)  [unwired: 4 in, 1 out]
        n664 = local read "浓度5"() -> (w1140:dbl)
        n665 = local read "泵滴定数4"() -> (w1142:dbl)
        n666 = call-poly <vilib>:"Write Key.vi"("section"=w1153, "error in (no error)"=w1182, "value"=w1140, "key"="浓度5", "refnum"=w1183) -> ("error out"=w1150:errorcluster, "refnum out"=w1151:T6)  [unwired: 4 in, 1 out]
        n667 = local read "泵滴定数5"() -> (w1143:dbl)
        n668 = call-poly <vilib>:"Write Key.vi"("section"=w1153, "error in (no error)"=w1150, "value"=w1142, "key"="泵滴定数4", "refnum"=w1151) -> ("error out"=w1187:errorcluster, "refnum out"=w1186:T6)  [unwired: 4 in, 1 out]
        n669 = call-poly <vilib>:"Write Key.vi"("section"=w1153, "error in (no error)"=w1187, "value"=w1143, "key"="泵滴定数5", "refnum"=w1186) -> ("error out"=w1148:errorcluster, "refnum out"=w1149:T6)  [unwired: 4 in, 1 out]
        n670 = local read "启用1"() -> (w1162:bool)
        n671 = call-poly <vilib>:"Write Key.vi"("section"=w1153, "error in (no error)"=w1148, "value"=w1162, "key"="启用1", "refnum"=w1149) -> ("error out"=w1158:errorcluster, "refnum out"=w1161:T6)  [unwired: 4 in, 1 out]
        n672 = local read "启用2"() -> (w1159:bool)
        n673 = call-poly <vilib>:"Write Key.vi"("section"=w1153, "error in (no error)"=w1158, "value"=w1159, "key"="启用2", "refnum"=w1161) -> ("error out"=w1169:errorcluster, "refnum out"=w1168:T6)  [unwired: 4 in, 1 out]
        n674 = local read "启用3"() -> (w1157:bool)
        n675 = call-poly <vilib>:"Write Key.vi"("section"=w1153, "error in (no error)"=w1169, "value"=w1157, "key"="启用3", "refnum"=w1168) -> ("error out"=w1167:errorcluster, "refnum out"=w1166:T6)  [unwired: 4 in, 1 out]
        n676 = local read "启用4"() -> (w1145:bool)
        n677 = call-poly <vilib>:"Write Key.vi"("section"=w1153, "error in (no error)"=w1167, "value"=w1145, "key"="启用4", "refnum"=w1166) -> ("error out"=w1165:errorcluster, "refnum out"=w1164:T6)  [unwired: 4 in, 1 out]
        n678 = local read "启用5"() -> (w1144:bool)
        n679 = call-poly <vilib>:"Write Key.vi"("section"=w1153, "error in (no error)"=w1165, "value"=w1144, "key"="启用5", "refnum"=w1164) -> ("error out"=w1146:errorcluster, "refnum out"=w1147:T6)  [unwired: 4 in, 1 out]
        n680 = call <vilib>:"Close Config Data.vi"("error in (no error)"=w1146, "refnum"=w1147) -> ("error out"=w1132:errorcluster, "file path"=w1133:path)  [unwired: 8 in]
        n681 = Open/Create/Replace File(file path (use dialog)=w1133, error in=w1132) -> (refnum out=w1135:refnum<file>, error out=w1134:errorcluster)  [unwired: 4 in, 1 out]
        n682 = Flush File(refnum=w1135, error in=w1134) -> (refnum out=w1136:refnum<file>, error out=w1137:errorcluster)
        n683 = Close File(refnum=w1136, error in=w1137) -> ()  [unwired: 2 out]
      }
      event "关闭", "关闭 2", "关闭 3", "关闭 4": Value Change {
        n684 = event-data() -> ()  [unwired: 1 in, 6 out]
        n685 = property on="窗格" class="Pane"("Origin"=T4 {"Horizontal"=0, "Vertical"=0} ("原点")) -> ()  [unwired: 2 in, 2 out]
      }
      event Application Instance Close {
        n686 = event-data() -> ()  [unwired: 1 in, 4 out]
      }
      event "时间校准": Value Change {
        n687 = event-data() -> ()  [unwired: 1 in, 6 out]
        n688 = Get Date/Time In Seconds() -> (seconds since 1Jan1904=w1217:timestamp)
        n689 = Build Array(w1217) -> (w1216:timestamp[])
        n690 = call "DateToHex.vi"("DATE"=w1216) -> ("数组"=w1214:u16[])  [unwired: 10 in]
        n691 = Insert Into Array(array=u16[] [1] ("values"), index=1 ("索引"), new element=w1214) -> (w1210:u16[])
        n692 = call "CODMnMB_api.vi"("STEP"=enum16{"open", "read", "write", "close"}."write", "values"=w1210, "starting address"=u16 4612) -> ("error out"=w1209:errorcluster)  [unwired: 6 in, 2 out]
        n693 = call <vilib>:"Clear Errors.vi"("error in (no error)"=w1209) -> ()  [unwired: 5 in, 2 out]
      }
      event "故障清除": Value Change {
        n694 = event-data() -> ()  [unwired: 1 in, 6 out]
        n695 = call "CODMnMB_api.vi"("STEP"=enum16{"open", "read", "write", "close"}."write", "values"=u16[] [1], "starting address"=u16 4611) -> ()  [unwired: 6 in, 3 out]
      }
      event "仪器参数": Value Change {
        n696 = event-data() -> ()  [unwired: 1 in, 6 out]
        n697 = global read "CODMn断电保存全局变量.vi" "CODMn仪器参数"() -> (w1221:T16)
        n698 = call "仪器参数设置.vi"("氨氮仪器参数"=w1221) -> ("仪器参数设置输出"=w1222:T17)  [unwired: 10 in]
        n699 = Unbundle By Name(w1222) -> ("确定"=w1223:bool)
        n700 = case shown="真" w1223 {
          tunnel: w1222 -> [_ w1225]
          tunnel: w1221 -> [_ w1224]
          frame False {
          }
          frame True {
            n701 = flat-sequence {
              tunnel: w1225 -> [w1242]
              tunnel: w1224 -> [w1241]
              frame #0 {
                n702 = Unbundle By Name(w1242) -> ("测量量程"=w1240:dbl, "测量精度"=w1239:dbl, "测量间隔"=w1238:dbl, "消解温度"=w1237:dbl, "消解时长"=w1236:dbl, "空白校准时间"=w1235:timestamp, "曲线截距"=w1234:dbl, "曲线斜率"=w1233:dbl, "测量检出限"=w1232:dbl, "测量信号值"=w1231:dbl, "线性相关系数"=w1230:dbl, "二次多项式系数"=w1229:dbl, "标样校准时间"=w1228:timestamp, "稀释倍数"=w1227:dbl)
                n703 = Bundle By Name(cluster=w1241, "测量量程"=w1240, "测量精度"=w1239, "测量间隔"=w1238, "消解温度"=w1237, "消解时长"=w1236, "空白校准时间"=w1235, "曲线截距"=w1234, "曲线斜率"=w1233, "测量检出限"=w1232, "测量信号值"=w1231, "线性相关系数"=w1230, "二次多项式系数"=w1229, "标样校准时间"=w1228, "稀释倍数"=w1227) -> (w1226:T16)
                n704 = global write "CODMn断电保存全局变量.vi" "CODMn仪器参数"(w1226) -> ()
              }
              frame #1 {
                n705 = call "配置文件保存.vi"() -> ()  [unwired: 12 in]
              }
            }
          }
        }
      }
      event "远程自动校准浓度", "远程校准量程": Value Change {
        n706 = event-data() -> ()  [unwired: 1 in, 6 out]
        n707 = flat-sequence {
          frame #0 {
            n708 = global write "CODMn断电保存全局变量.vi" "远程校准量程"("远程校准量程") -> ()
            n709 = global write "CODMn断电保存全局变量.vi" "远程自动校准浓度"("远程自动校准浓度") -> ()
          }
          frame #1 {
            n710 = call "配置文件保存.vi"() -> ()  [unwired: 12 in]
          }
        }
      }
      event "测量模式(公式)": Value Change {
        n711 = event-data() -> ()  [unwired: 1 in, 6 out]
        n712 = flat-sequence {
          tunnel: w1246 -> [w1248]
          tunnel: w1245 -> [w1247]
          frame #0 {
            n713 = Bundle By Name(cluster=cluster{"命令":string} {"命令"=""} ("元素"), "命令"="CODMn读取公式" ("名称（未命名）")) -> (w1249:cluster{"命令":string})
            n714 = global write "CODMn断电保存全局变量.vi" "测量模式(公式)"("测量模式(公式)") -> ()
            n715 = Enqueue Element(queue=w1248, element=w1249, error in (no error)=w1247) -> ()  [unwired: 1 in, 3 out]
          }
          frame #1 {
            n716 = call "配置文件保存.vi"() -> ()  [unwired: 12 in]
          }
        }
      }
      event "跨度量程选择", "跨度液浓度", "零点核查量程选择", "零点核查浓度", "标样浓度", "标样核查量程选择", "加标回收量程：": Value Change {
        n717 = event-data() -> ()  [unwired: 1 in, 6 out]
        n718 = flat-sequence {
          frame #0 {
            n719 = global write "CODMn断电保存全局变量.vi" "标样浓度"("标样浓度") -> ()
            n720 = global write "CODMn断电保存全局变量.vi" "零点核查浓度"("零点核查浓度") -> ()
            n721 = global write "CODMn断电保存全局变量.vi" "跨度液浓度"("跨度液浓度") -> ()
            n722 = global write "CODMn断电保存全局变量.vi" "CODMn跨度量程选择"("跨度量程选择") -> ()
            n723 = global write "CODMn断电保存全局变量.vi" "加标回收量程选择"("加标回收量程：") -> ()
            n724 = global write "CODMn断电保存全局变量.vi" "标样核查量程选择"("标样核查量程选择") -> ()
            n725 = global write "CODMn断电保存全局变量.vi" "零点核查量程选择"("零点核查量程选择") -> ()
          }
          frame #1 {
            n726 = call "配置文件保存.vi"() -> ()  [unwired: 12 in]
          }
        }
      }
      event "校准1", "校准2", "校准3", "校准4", "校准5": Value Change {
        n727 = event-data() -> ()  [unwired: 1 in, 6 out]
        n728 = flat-sequence {
          tunnel: w1263 -> [w1272]
          tunnel: [w1272] -> w1265
          tunnel: w1260 -> [w1271]
          tunnel: [w1271] -> w1262
          tunnel: w1265 -> [w1308]
          tunnel: [w1308] -> w1264
          tunnel: w1262 -> [w1307]
          tunnel: [w1307] -> w1261
          tunnel: w1264 -> [w1335]
          tunnel: w1261 -> [w1334]
          frame #0 {
            n729 = Build Array("校准1", "校准2", "校准3", "校准4", "校准5") -> (w1275:bool[])
            n730 = for {
              tunnel: w1275 -> [w1290] mode=indexing
              tunnel: [w1282] -> w1266
              i -> [w1283]
              n731 = case shown="4" w1283 {
                tunnel: ["浓度1" "浓度2" "浓度3" "浓度4" "浓度5"] -> w1286
                frame 0, Default {
                }
                frame 1 {
                }
                frame 2 {
                }
                frame 3 {
                }
                frame 4 {
                }
              }
              n732 = Multiply(x=w1286, y=100.0) -> (x*y=w1284:dbl)
              n733 = Insert Into Array(array=u16[] [] ("values"), index=0 ("索引"), new element=w1284) -> (w1287:u16[])
              n734 = case shown="真" w1290 {
                tunnel: w1287 -> [_ w1299]
                tunnel: w1283 -> [_ w1301]
                tunnel: [_ w1296] -> w1282
                frame False {
                }
                frame True {
                  n735 = Increment(x=w1301) -> (x+1=w1297:i32)
                  n736 = global write "COD内部交互全局.vi" "当前校准"(w1297) -> ()
                  n737 = call "CODMnMB_api.vi"("STEP"=enum16{"open", "read", "write", "close"}."write", "values"=w1299, "starting address"=u16 4274) -> ("error out"=w1296:errorcluster)  [unwired: 6 in, 2 out]
                }
              }
            }
            n738 = local read "量程选择"() -> (w1268:enum16{"低量程", "高量程", "0-2量程"})
            n739 = case shown="\"高量程\"" w1268 {
              tunnel: [u16[] [0] ("values") u16[] [1] ("values") u16[] [0] ("values")] -> w1267
              frame "低量程", Default {
              }
              frame "高量程" {
              }
              frame "0-2量程" {
              }
            }
            n740 = call "CODMnMB_api.vi"("STEP"=enum16{"open", "read", "write", "close"}."write", "Error in"=w1266, "values"=w1267, "starting address"=u16 4276) -> ()  [unwired: 5 in, 3 out]
          }
          frame #1 {
            n741 = global read "COD内部交互全局.vi" "当前校准"() -> (w1309:i32)
            n742 = case shown="5" w1309 {
              tunnel: [w1317 w1318 w1319 w1320 w1321] -> w1305
              frame 1, Default {
                n743 = local read "浓度1"() -> (w1317:dbl)
              }
              frame 2 {
                n744 = local read "浓度2"() -> (w1318:dbl)
              }
              frame 3 {
                n745 = local read "浓度3"() -> (w1319:dbl)
              }
              frame 4 {
                n746 = local read "浓度4"() -> (w1320:dbl)
              }
              frame 5 {
                n747 = local read "浓度5"() -> (w1321:dbl)
              }
            }
            n748 = Number To Decimal String(number=w1305) -> (decimal integer string=w1304:string)  [unwired: 1 in]
            n749 = Concatenate Strings("仪器校准中!\n当前校准浓度为:", w1304, "mg/L" ("字符串")) -> (w1302:string)
            n750 = Not Equal To 0?(x=w1305) -> (x != 0?=w1313:bool)
            n751 = global write "COD内部交互全局.vi" "校准内容显示"(w1302) -> ()
            n752 = case shown="真" w1313 {
              tunnel: [u16 8 ("address") u16 9 ("address")] -> w1316
              tunnel: ["校零" ("测量模式") "校标" ("测量模式")] -> _
              frame False {
              }
              frame True {
              }
            }
            n753 = Insert Into Array(array=u16[] [] ("values"), index=0 ("索引"), new element=w1316) -> (w1310:u16[])
            n754 = call "CODMnMB_api.vi"("STEP"=enum16{"open", "read", "write", "close"}."write", "values"=w1310, "starting address"=u16 4608 ("address")) -> ()  [unwired: 6 in, 3 out]
          }
          frame #2 {
            n755 = local read "选用水样"() -> (w1343:enum16{"葡萄糖", "草酸钠"})
            n756 = global read "CODMN外部API.vi" "ping"() -> (w1333:bool)
            n757 = case shown="假" w1333 {
              tunnel: [w1351 w1354] -> w1332
              frame False {
                n758 = global read "COD内部交互全局.vi" "配置文件ini"() -> (w1353:string)
                n759 = call <vilib>:"Application Directory.vi"() -> ("Application Directory"=w1352:path)
                n760 = Build Path(base path=w1352, name or relative path=w1353) -> (appended path=w1351:path)
              }
              frame True {
                n761 = global read "CODMN外部API.vi" "配置文件 path"() -> (w1354:path)
              }
            }
            n762 = local read "量程选择"() -> (w1342:enum16{"低量程", "高量程", "0-2量程"})
            n763 = case shown="\"葡萄糖\", 默认" w1343 {
              tunnel: ["葡萄糖标线" ("section") "草酸钠标线" ("section")] -> w1344
              frame "葡萄糖", Default {
              }
              frame "草酸钠" {
              }
            }
            n764 = Bundle By Name(cluster=cluster{"命令":string} {"命令"=""} ("元素"), "命令"="CODMn读取参数" ("名称（未命名）")) -> (w1339:cluster{"命令":string})
            n765 = case shown="\"0-2量程\"" w1342 {
              tunnel: ["低量程" "高量程" "0-2量程"] -> w1345
              frame "低量程", Default {
              }
              frame "高量程" {
              }
              frame "0-2量程" {
              }
            }
            n766 = global read "COD内部交互全局.vi" "当前校准"() -> (w1340:i32)
            n767 = Enqueue Element(queue=w1335, element=w1339, timeout in ms (-1)=1000 ("超时毫秒(-1)"), error in (no error)=w1334) -> ()  [unwired: 3 out]
            n768 = Concatenate Strings(w1344, w1345) -> (w1341:string)
            n769 = call <vilib>:"Open Config Data.vi"("configuration file path"=w1332) -> ("error out"=w1349:errorcluster, "refnum"=w1350:T6)  [unwired: 8 in, 1 out]
            n770 = call-poly <vilib>:"Write Key.vi"("section"=w1341, "error in (no error)"=w1349, "value"=w1340, "key"="当前选用的校准" ("section"), "refnum"=w1350) -> ("error out"=w1346:errorcluster, "refnum out"=w1347:T6)  [unwired: 4 in, 1 out]
            n771 = call <vilib>:"Close Config Data.vi"("error in (no error)"=w1346, "refnum"=w1347) -> ("error out"=w1326:errorcluster, "file path"=w1327:path)  [unwired: 8 in]
            n772 = Open/Create/Replace File(file path (use dialog)=w1327, error in=w1326) -> (refnum out=w1329:refnum<file>, error out=w1328:errorcluster)  [unwired: 4 in, 1 out]
            n773 = Flush File(refnum=w1329, error in=w1328) -> (refnum out=w1330:refnum<file>, error out=w1331:errorcluster)
            n774 = Close File(refnum=w1330, error in=w1331) -> ()  [unwired: 2 out]
          }
        }
      }
      event "水样量程选择:", "低切高阈值:", "高切低阈值:": Value Change {
        n775 = event-data() -> ()  [unwired: 1 in, 6 out]
        n776 = flat-sequence {
          frame #0 {
            n777 = global write "CODMn断电保存全局变量.vi" "高切低阈值:"("高切低阈值:") -> ()
            n778 = global write "CODMn断电保存全局变量.vi" "自动切换量程:"("水样量程选择:") -> ()
            n779 = global write "CODMn断电保存全局变量.vi" "低切高阈值:"("低切高阈值:") -> ()
          }
          frame #1 {
            n780 = call "配置文件保存.vi"() -> ()  [unwired: 12 in]
          }
        }
      }
      event "模型": Value Change {
        n781 = event-data() -> ()  [unwired: 1 in, 6 out]
        n782 = global read "CODMN外部API.vi" "ping"() -> (w1370:bool)
        n783 = case shown="假" w1370 {
          tunnel: [w1378 w1381] -> w1369
          frame False {
            n784 = global read "COD内部交互全局.vi" "配置文件ini"() -> (w1380:string)
            n785 = call <vilib>:"Application Directory.vi"() -> ("Application Directory"=w1379:path)
            n786 = Build Path(base path=w1379, name or relative path=w1380) -> (appended path=w1378:path)
          }
          frame True {
            n787 = global read "CODMN外部API.vi" "配置文件 path"() -> (w1381:path)
          }
        }
        n788 = call <vilib>:"Open Config Data.vi"("configuration file path"=w1369) -> ("error out"=w1376:errorcluster, "refnum"=w1377:T6)  [unwired: 8 in, 1 out]
        n789 = local read "模型"() -> (w1371:enum32{"线性", "多项式"})
        n790 = call-poly <vilib>:"Write Key.vi"("section"="CODMn模型选择" ("key"), "error in (no error)"=w1376, "value"=w1371, "key"="线性和多项式", "refnum"=w1377) -> ("error out"=w1372:errorcluster, "refnum out"=w1373:T6)  [unwired: 4 in, 1 out]
        n791 = call <vilib>:"Close Config Data.vi"("error in (no error)"=w1372, "refnum"=w1373) -> ("error out"=w1363:errorcluster, "file path"=w1364:path)  [unwired: 8 in]
        n792 = Open/Create/Replace File(file path (use dialog)=w1364, error in=w1363) -> (refnum out=w1366:refnum<file>, error out=w1365:errorcluster)  [unwired: 4 in, 1 out]
        n793 = Flush File(refnum=w1366, error in=w1365) -> (refnum out=w1367:refnum<file>, error out=w1368:errorcluster)
        n794 = Close File(refnum=w1367, error in=w1368) -> ()  [unwired: 2 out]
      }
      event "浓度1", "浓度2", "浓度3", "泵滴定数1", "泵滴定数2", "泵滴定数3", "启用1", "启用2", "启用3", "浓度4", "浓度5", "泵滴定数4", "泵滴定数5", "启用4", "启用5": Value Change {
        n795 = event-data() -> ()  [unwired: 1 in, 6 out]
        n796 = local read "选用水样"() -> (w1405:enum16{"葡萄糖", "草酸钠"})
        n797 = local read "量程选择"() -> (w1404:enum16{"低量程", "高量程", "0-2量程"})
        n798 = case shown="\"葡萄糖\", 默认" w1405 {
          tunnel: ["葡萄糖标线" ("section") "草酸钠标线" ("section")] -> w1411
          frame "葡萄糖", Default {
          }
          frame "草酸钠" {
          }
        }
        n799 = case shown="\"0-2量程\"" w1404 {
          tunnel: ["低量程" "高量程" "0-2量程"] -> w1402
          frame "低量程", Default {
          }
          frame "高量程" {
          }
          frame "0-2量程" {
          }
        }
        n800 = global read "CODMN外部API.vi" "ping"() -> (w1389:bool)
        n801 = case shown="假" w1389 {
          tunnel: [w1462 w1465] -> w1388
          frame False {
            n802 = global read "COD内部交互全局.vi" "配置文件ini"() -> (w1464:string)
            n803 = call <vilib>:"Application Directory.vi"() -> ("Application Directory"=w1463:path)
            n804 = Build Path(base path=w1463, name or relative path=w1464) -> (appended path=w1462:path)
          }
          frame True {
            n805 = global read "CODMN外部API.vi" "配置文件 path"() -> (w1465:path)
          }
        }
        n806 = Concatenate Strings(w1411, w1402) -> (w1403:string)
        n807 = call <vilib>:"Open Config Data.vi"("configuration file path"=w1388) -> ("error out"=w1460:errorcluster, "refnum"=w1461:T6)  [unwired: 8 in, 1 out]
        n808 = local read "浓度1"() -> (w1458:dbl)
        n809 = call-poly <vilib>:"Write Key.vi"("section"=w1403, "error in (no error)"=w1460, "value"=w1458, "key"="浓度1", "refnum"=w1461) -> ("error out"=w1457:errorcluster, "refnum out"=w1456:T6)  [unwired: 4 in, 1 out]
        n810 = local read "浓度2"() -> (w1442:dbl)
        n811 = call-poly <vilib>:"Write Key.vi"("section"=w1403, "error in (no error)"=w1457, "value"=w1442, "key"="浓度2", "refnum"=w1456) -> ("error out"=w1455:errorcluster, "refnum out"=w1454:T6)  [unwired: 4 in, 1 out]
        n812 = local read "浓度3"() -> (w1438:dbl)
        n813 = local read "泵滴定数1"() -> (w1436:dbl)
        n814 = call-poly <vilib>:"Write Key.vi"("section"=w1403, "error in (no error)"=w1455, "value"=w1438, "key"="浓度3", "refnum"=w1454) -> ("error out"=w1453:errorcluster, "refnum out"=w1452:T6)  [unwired: 4 in, 1 out]
        n815 = local read "泵滴定数2"() -> (w1434:dbl)
        n816 = call-poly <vilib>:"Write Key.vi"("section"=w1403, "error in (no error)"=w1453, "value"=w1436, "key"="泵滴定数1", "refnum"=w1452) -> ("error out"=w1451:errorcluster, "refnum out"=w1450:T6)  [unwired: 4 in, 1 out]
        n817 = local read "泵滴定数3"() -> (w1432:dbl)
        n818 = call-poly <vilib>:"Write Key.vi"("section"=w1403, "error in (no error)"=w1451, "value"=w1434, "key"="泵滴定数2", "refnum"=w1450) -> ("error out"=w1449:errorcluster, "refnum out"=w1448:T6)  [unwired: 4 in, 1 out]
        n819 = call-poly <vilib>:"Write Key.vi"("section"=w1403, "error in (no error)"=w1449, "value"=w1432, "key"="泵滴定数3", "refnum"=w1448) -> ("error out"=w1447:errorcluster, "refnum out"=w1446:T6)  [unwired: 4 in, 1 out]
        n820 = local read "浓度4"() -> (w1401:dbl)
        n821 = call-poly <vilib>:"Write Key.vi"("section"=w1403, "error in (no error)"=w1447, "value"=w1401, "key"="浓度4", "refnum"=w1446) -> ("error out"=w1440:errorcluster, "refnum out"=w1441:T6)  [unwired: 4 in, 1 out]
        n822 = local read "浓度5"() -> (w1400:dbl)
        n823 = local read "泵滴定数4"() -> (w1397:dbl)
        n824 = call-poly <vilib>:"Write Key.vi"("section"=w1403, "error in (no error)"=w1440, "value"=w1400, "key"="浓度5", "refnum"=w1441) -> ("error out"=w1398:errorcluster, "refnum out"=w1399:T6)  [unwired: 4 in, 1 out]
        n825 = local read "泵滴定数5"() -> (w1396:dbl)
        n826 = call-poly <vilib>:"Write Key.vi"("section"=w1403, "error in (no error)"=w1398, "value"=w1397, "key"="泵滴定数4", "refnum"=w1399) -> ("error out"=w1445:errorcluster, "refnum out"=w1444:T6)  [unwired: 4 in, 1 out]
        n827 = call-poly <vilib>:"Write Key.vi"("section"=w1403, "error in (no error)"=w1445, "value"=w1396, "key"="泵滴定数5", "refnum"=w1444) -> ("error out"=w1394:errorcluster, "refnum out"=w1395:T6)  [unwired: 4 in, 1 out]
        n828 = local read "启用1"() -> (w1420:bool)
        n829 = call-poly <vilib>:"Write Key.vi"("section"=w1403, "error in (no error)"=w1394, "value"=w1420, "key"="启用1", "refnum"=w1395) -> ("error out"=w1416:errorcluster, "refnum out"=w1419:T6)  [unwired: 4 in, 1 out]
        n830 = local read "启用2"() -> (w1417:bool)
        n831 = call-poly <vilib>:"Write Key.vi"("section"=w1403, "error in (no error)"=w1416, "value"=w1417, "key"="启用2", "refnum"=w1419) -> ("error out"=w1427:errorcluster, "refnum out"=w1426:T6)  [unwired: 4 in, 1 out]
        n832 = local read "启用3"() -> (w1415:bool)
        n833 = call-poly <vilib>:"Write Key.vi"("section"=w1403, "error in (no error)"=w1427, "value"=w1415, "key"="启用3", "refnum"=w1426) -> ("error out"=w1425:errorcluster, "refnum out"=w1424:T6)  [unwired: 4 in, 1 out]
        n834 = local read "启用4"() -> (w1390:bool)
        n835 = call-poly <vilib>:"Write Key.vi"("section"=w1403, "error in (no error)"=w1425, "value"=w1390, "key"="启用4", "refnum"=w1424) -> ("error out"=w1423:errorcluster, "refnum out"=w1422:T6)  [unwired: 4 in, 1 out]
        n836 = local read "启用5"() -> (w1391:bool)
        n837 = local read "选用水样"() -> (w1410:enum16{"葡萄糖", "草酸钠"})
        n838 = call-poly <vilib>:"Write Key.vi"("section"=w1403, "error in (no error)"=w1423, "value"=w1391, "key"="启用5", "refnum"=w1422) -> ("error out"=w1392:errorcluster, "refnum out"=w1393:T6)  [unwired: 4 in, 1 out]
        n839 = call-poly <vilib>:"Write Key.vi"("section"="标线选择", "error in (no error)"=w1392, "value"=w1410, "key"="选用水样", "refnum"=w1393) -> ("error out"=w1407:errorcluster, "refnum out"=w1408:T6)  [unwired: 4 in, 1 out]
        n840 = call <vilib>:"Close Config Data.vi"("error in (no error)"=w1407, "refnum"=w1408) -> ("error out"=w1382:errorcluster, "file path"=w1383:path)  [unwired: 8 in]
        n841 = Open/Create/Replace File(file path (use dialog)=w1383, error in=w1382) -> (refnum out=w1385:refnum<file>, error out=w1384:errorcluster)  [unwired: 4 in, 1 out]
        n842 = Flush File(refnum=w1385, error in=w1384) -> (refnum out=w1386:refnum<file>, error out=w1387:errorcluster)
        n843 = Close File(refnum=w1386, error in=w1387) -> ()  [unwired: 2 out]
      }
      event "读取": Value Change {
        (unwired) u16 94 ("number of holding registers")
        (unwired) u16 4616 ("starting address")
        n844 = event-data() -> ()  [unwired: 1 in, 6 out]
        n845 = Bundle By Name(cluster=cluster{"命令":string} {"命令"=""} ("元素"), "命令"="CODMn读取公式" ("名称（未命名）")) -> (w1471:cluster{"命令":string})
        n846 = Enqueue Element(queue=w1475, element=w1471, error in (no error)=w1474) -> ()  [unwired: 1 in, 3 out]
      }
      event "写入": Mouse Down {
        n847 = event-data() -> ()  [unwired: 1 in, 8 out]
        n848 = call <vilib>:"Three Button Dialog.vi"("Allow user to close window? (TRUE)"=FALSE, "Center Button Text (\"No\")"="一键写入所有公式" ("F按钮名称（“取消”）"), "Left Button Text (\"Yes\")"="写入当前公式" ("T按钮名称（“确定”）"), "message"="即将将左侧拟合公式写入仪器\n请选择写入当前模式和量程还是一键写入所有模式量程！" ("消息")) -> ("Which Button?"=w1476:T18)  [unwired: 7 in]
        n849 = case shown="\"Window Close\"" w1476 {
          frame "Left Button", Default {
            n850 = local read "测量模式(公式)"() -> (w1482:u16)
            n851 = local read "量程选择"() -> (w1481:enum16{"低量程", "高量程", "0-2量程"})
            n852 = local read "模型"() -> (w1492:enum32{"线性", "多项式"})
            n853 = case shown="\"线性\", 默认" w1492 {
              tunnel: [w1535 w1578] -> w1490
              tunnel: [w1534 w1577] -> w1489
              tunnel: w1482 -> [w1533 _]
              tunnel: w1481 -> [w1532 _]
              frame "线性", Default {
                (unwired) "线性" ("table输入")
                n854 = case shown="1" w1533 {
                  tunnel: [u16 4626 ("starting address") w1542 w1547 w1552 w1557 w1562 w1567 w1572] -> w1535
                  tunnel: w1532 -> [_ w1541 _ _ _ _ _ _]
                  frame 0, Default {
                  }
                  frame 1 {
                    n855 = case shown="\"低量程\", 默认" w1541 {
                      tunnel: [u16 4626 ("starting address") u16 4632 ("starting address") u16 4638 ("starting address")] -> w1542
                      frame "低量程", Default {
                      }
                      frame "高量程" {
                      }
                      frame "0-2量程" {
                      }
                    }
                  }
                  frame 2 {
                    n856 = local read "量程选择"() -> (w1546:enum16{"低量程", "高量程", "0-2量程"})
                    n857 = case shown="\"低量程\", 默认" w1546 {
                      tunnel: [u16 4638 ("starting address") u16 4644 ("starting address") u16 4638 ("starting address")] -> w1547
                      frame "低量程", Default {
                      }
                      frame "高量程" {
                      }
                      frame "0-2量程" {
                      }
                    }
                  }
                  frame 3 {
                    n858 = local read "量程选择"() -> (w1551:enum16{"低量程", "高量程", "0-2量程"})
                    n859 = case shown="\"低量程\", 默认" w1551 {
                      tunnel: [u16 4650 ("starting address") u16 4656 ("starting address") u16 4638 ("starting address")] -> w1552
                      frame "低量程", Default {
                      }
                      frame "高量程" {
                      }
                      frame "0-2量程" {
                      }
                    }
                  }
                  frame 4 {
                    n860 = local read "量程选择"() -> (w1556:enum16{"低量程", "高量程", "0-2量程"})
                    n861 = case shown="\"低量程\", 默认" w1556 {
                      tunnel: [u16 4662 ("starting address") u16 4668 ("starting address") u16 4638 ("starting address")] -> w1557
                      frame "低量程", Default {
                      }
                      frame "高量程" {
                      }
                      frame "0-2量程" {
                      }
                    }
                  }
                  frame 5 {
                    n862 = local read "量程选择"() -> (w1561:enum16{"低量程", "高量程", "0-2量程"})
                    n863 = case shown="\"低量程\", 默认" w1561 {
                      tunnel: [u16 4674 ("starting address") u16 4680 ("starting address") u16 4638 ("starting address")] -> w1562
                      frame "低量程", Default {
                      }
                      frame "高量程" {
                      }
                      frame "0-2量程" {
                      }
                    }
                  }
                  frame 6 {
                    n864 = local read "量程选择"() -> (w1566:enum16{"低量程", "高量程", "0-2量程"})
                    n865 = case shown="\"低量程\", 默认" w1566 {
                      tunnel: [u16 4686 ("starting address") u16 4692 ("starting address") u16 4638 ("starting address")] -> w1567
                      frame "低量程", Default {
                      }
                      frame "高量程" {
                      }
                      frame "0-2量程" {
                      }
                    }
                  }
                  frame 7 {
                    n866 = local read "量程选择"() -> (w1571:enum16{"低量程", "高量程", "0-2量程"})
                    n867 = case shown="\"低量程\", 默认" w1571 {
                      tunnel: [u16 4698 ("starting address") u16 4704 ("starting address") u16 4638 ("starting address")] -> w1572
                      frame "低量程", Default {
                      }
                      frame "高量程" {
                      }
                      frame "0-2量程" {
                      }
                    }
                  }
                }
                n868 = local read "K"() -> (w1539:dbl)
                n869 = local read "b"() -> (w1538:dbl)
                n870 = Build Array(w1539, w1538, 0.0 ("元素")) -> (w1537:dbl[])
                n871 = call "浮点转CDAB整形cod.vi"("浮点数"=w1537) -> ("CDAB整形输出"=w1534:u16[])  [unwired: 10 in]
              }
              frame "多项式" {
                (unwired) "多项式" ("table输入")
                # "b,k,c"
                n872 = local read "多项式系数"() -> (w1583:dbl[])
                n873 = local read "测量模式(公式)"() -> (w1579:u16)
                n874 = Index Array(array=w1583) -> (element #1=w1581:dbl, element #2=w1576:dbl, element #3=w1580:dbl)  [unwired: 3 in]
                n875 = case shown="1" w1579 {
                  tunnel: [u16 4626 ("starting address") w1586 w1591 w1596 w1601 w1606 w1611 w1616] -> w1578
                  frame 0, Default {
                  }
                  frame 1 {
                    n876 = local read "量程选择"() -> (w1585:enum16{"低量程", "高量程", "0-2量程"})
                    n877 = case shown="\"低量程\", 默认" w1585 {
                      tunnel: [u16 4626 ("starting address") u16 4632 ("starting address") u16 4638 ("starting address")] -> w1586
                      frame "低量程", Default {
                      }
                      frame "高量程" {
                      }
                      frame "0-2量程" {
                      }
                    }
                  }
                  frame 2 {
                    n878 = local read "量程选择"() -> (w1590:enum16{"低量程", "高量程", "0-2量程"})
                    n879 = case shown="\"低量程\", 默认" w1590 {
                      tunnel: [u16 4638 ("starting address") u16 4644 ("starting address") u16 4638 ("starting address")] -> w1591
                      frame "低量程", Default {
                      }
                      frame "高量程" {
                      }
                      frame "0-2量程" {
                      }
                    }
                  }
                  frame 3 {
                    n880 = local read "量程选择"() -> (w1595:enum16{"低量程", "高量程", "0-2量程"})
                    n881 = case shown="\"低量程\", 默认" w1595 {
                      tunnel: [u16 4650 ("starting address") u16 4656 ("starting address") u16 4638 ("starting address")] -> w1596
                      frame "低量程", Default {
                      }
                      frame "高量程" {
                      }
                      frame "0-2量程" {
                      }
                    }
                  }
                  frame 4 {
                    n882 = local read "量程选择"() -> (w1600:enum16{"低量程", "高量程", "0-2量程"})
                    n883 = case shown="\"低量程\", 默认" w1600 {
                      tunnel: [u16 4662 ("starting address") u16 4668 ("starting address") u16 4638 ("starting address")] -> w1601
                      frame "低量程", Default {
                      }
                      frame "高量程" {
                      }
                      frame "0-2量程" {
                      }
                    }
                  }
                  frame 5 {
                    n884 = local read "量程选择"() -> (w1605:enum16{"低量程", "高量程", "0-2量程"})
                    n885 = case shown="\"低量程\", 默认" w1605 {
                      tunnel: [u16 4674 ("starting address") u16 4680 ("starting address") u16 4638 ("starting address")] -> w1606
                      frame "低量程", Default {
                      }
                      frame "高量程" {
                      }
                      frame "0-2量程" {
                      }
                    }
                  }
                  frame 6 {
                    n886 = local read "量程选择"() -> (w1610:enum16{"低量程", "高量程", "0-2量程"})
                    n887 = case shown="\"低量程\", 默认" w1610 {
                      tunnel: [u16 4686 ("starting address") u16 4692 ("starting address") u16 4638 ("starting address")] -> w1611
                      frame "低量程", Default {
                      }
                      frame "高量程" {
                      }
                      frame "0-2量程" {
                      }
                    }
                  }
                  frame 7 {
                    n888 = local read "量程选择"() -> (w1615:enum16{"低量程", "高量程", "0-2量程"})
                    n889 = case shown="\"低量程\", 默认" w1615 {
                      tunnel: [u16 4698 ("starting address") u16 4704 ("starting address") u16 4638 ("starting address")] -> w1616
                      frame "低量程", Default {
                      }
                      frame "高量程" {
                      }
                      frame "0-2量程" {
                      }
                    }
                  }
                }
                n890 = Build Array(w1576, w1581, w1580) -> (w1582:dbl[])
                n891 = call "浮点转CDAB整形cod.vi"("浮点数"=w1582) -> ("CDAB整形输出"=w1577:u16[])  [unwired: 10 in]
              }
            }
            n892 = local read "多项式系数"() -> (w1486:dbl[])
            n893 = call "CODMnMB_api.vi"("STEP"=enum16{"open", "read", "write", "close"}."write", "values"=w1489, "starting address"=w1490) -> ("error out"=w1488:errorcluster)  [unwired: 6 in, 2 out]
            n894 = Index Array(array=w1486) -> (element #1=w1485:dbl, element #2=w1484:dbl, element #3=w1483:dbl)  [unwired: 3 in]
            n895 = case shown="无错误" w1488 {
              tunnel: ["写入成功！" "写入失败！"] -> w1487
              tunnel: w1485 -> [w1493 _]
              tunnel: w1484 -> [w1494 _]
              tunnel: w1483 -> [w1495 _]
              tunnel: w1482 -> [w1500 _]
              tunnel: w1481 -> [w1499 _]
              frame No Error {
                w1502 = u16 1 items=["水样测试"=1, "标样核查"=2, "零点核查"=3, "跨度核查"=4, "空白测试"=5, "平行样"=6, "加标回收"=7] ("测量模式(公式)")
                n896 = Number To Fractional String(number=w1493) -> (F-format string=w1504:string)  [unwired: 3 in]
                n897 = Number To Fractional String(number=w1494) -> (F-format string=w1505:string)  [unwired: 3 in]
                n898 = Number To Fractional String(number=w1495) -> (F-format string=w1503:string)  [unwired: 3 in]
                n899 = property on="模型" class="Enum (严格)"() -> ("RingText.Text"=w1515:string)  [unwired: 2 in, 2 out]
                n900 = property on="测量模式(公式)" class="Ring (严格)"() -> ("RingText.Text"=w1514:string)  [unwired: 2 in, 2 out]
                n901 = property on="量程选择" class="Enum (严格)"() -> ("RingText.Text"=w1513:string)  [unwired: 2 in, 2 out]
                n902 = Concatenate Strings("变更后:" ("table输入"), "K:" ("字符串"), w1505, "B:" ("字符串"), w1504, "X^2:" ("字符串"), w1503) -> (w1506:string)
                n903 = Concatenate Strings(w1515, w1514, w1513, "公式改变" ("日志信息")) -> (w1507:string)
                n904 = Equal?(x=w1500, y=w1502) -> (x = y?=w1498:bool)
                n905 = Equal?(x=w1499, y=enum16{"低量程", "高量程", "0-2量程"}."低量程" ("量程选择")) -> (x = y?=w1497:bool)
                n906 = Compound Arithmetic op=AND ("复合运算")(w1498, w1497) -> (w1496:bool)
                n907 = case shown="真" w1496 {
                  tunnel: w1494 -> [_ w1528]
                  tunnel: w1493 -> [_ w1527]
                  tunnel: w1495 -> [_ w1526]
                  frame False {
                  }
                  frame True {
                    n908 = global read "CODMn断电保存全局变量.vi" "CODMn仪器参数"() -> (w1529:T16)
                    n909 = Bundle By Name(cluster=w1529, "曲线截距"=w1527, "曲线斜率"=w1528, "二次多项式系数"=w1526) -> (w1530:T16)
                    n910 = global write "CODMn断电保存全局变量.vi" "CODMn仪器参数"(w1530) -> ()
                  }
                }
                n911 = Get Date/Time In Seconds() -> (seconds since 1Jan1904=w1519:timestamp)
                n912 = Bundle(cluster=T15 {"时间标识"=timestamp(0 s since 1904-01-01), "参数"="", "日志信息"="", "流程参数"=""} ("data in"), "时间标识"=w1519, "参数"="CODMn" ("table输入"), "日志信息"=w1507, "流程参数"=w1506) -> (w1517:T15)
                n913 = call "流程日志字段定义.vi"("table输入"="操作日志", "data in"=w1517) -> ("table输出"=w1522:string, "columns"=w1523:string[], "data out"=w1524:T19)  [unwired: 7 in]
                n914 = call "插入数据.vi"("data"=w1524, "columns"=w1523, "database"="database3.mdb", "table"=w1522) -> ()  [unwired: 7 in, 1 out]
              }
              frame Error {
              }
            }
            n915 = One Button Dialog(message=w1487) -> ()  [unwired: 1 in, 1 out]
          }
          frame "Center Button" {
            n916 = local read "模型"() -> (w1622:enum32{"线性", "多项式"})
            n917 = case shown="\"线性\", 默认" w1622 {
              tunnel: [w1653 w1704] -> w1620
              frame "线性", Default {
                n918 = property on="测量模式(公式)" class="Ring (严格)"() -> ("NumItems"=w1654:u32)  [unwired: 2 in, 2 out]
                n919 = for {
                  N: w1654 -> [_]
                  tunnel: [w1655] -> w1653
                  i -> [w1660]
                  n920 = Increment(x=w1660) -> (x+1=w1659:i32)
                  n921 = local read "K"() -> (w1664:dbl)
                  n922 = local read "b"() -> (w1665:dbl)
                  n923 = case shown="1" w1659 {
                    tunnel: [u16 4626 ("starting address") w1670 w1675 w1680 w1685 w1690 w1695 w1700] -> w1657
                    frame 0, Default {
                    }
                    frame 1 {
                      n924 = local read "量程选择"() -> (w1669:enum16{"低量程", "高量程", "0-2量程"})
                      n925 = case shown="\"低量程\", 默认" w1669 {
                        tunnel: [u16 4626 ("starting address") u16 4632 ("starting address") u16 4638 ("starting address")] -> w1670
                        frame "低量程", Default {
                        }
                        frame "高量程" {
                        }
                        frame "0-2量程" {
                        }
                      }
                    }
                    frame 2 {
                      n926 = local read "量程选择"() -> (w1674:enum16{"低量程", "高量程", "0-2量程"})
                      n927 = case shown="\"低量程\", 默认" w1674 {
                        tunnel: [u16 4638 ("starting address") u16 4644 ("starting address") u16 4638 ("starting address")] -> w1675
                        frame "低量程", Default {
                        }
                        frame "高量程" {
                        }
                        frame "0-2量程" {
                        }
                      }
                    }
                    frame 3 {
                      n928 = local read "量程选择"() -> (w1679:enum16{"低量程", "高量程", "0-2量程"})
                      n929 = case shown="\"低量程\", 默认" w1679 {
                        tunnel: [u16 4650 ("starting address") u16 4656 ("starting address") u16 4638 ("starting address")] -> w1680
                        frame "低量程", Default {
                        }
                        frame "高量程" {
                        }
                        frame "0-2量程" {
                        }
                      }
                    }
                    frame 4 {
                      n930 = local read "量程选择"() -> (w1684:enum16{"低量程", "高量程", "0-2量程"})
                      n931 = case shown="\"高量程\"" w1684 {
                        tunnel: [u16 4662 ("starting address") u16 4668 ("starting address") u16 4638 ("starting address")] -> w1685
                        frame "低量程", Default {
                        }
                        frame "高量程" {
                        }
                        frame "0-2量程" {
                        }
                      }
                    }
                    frame 5 {
                      n932 = local read "量程选择"() -> (w1689:enum16{"低量程", "高量程", "0-2量程"})
                      n933 = case shown="\"低量程\", 默认" w1689 {
                        tunnel: [u16 4674 ("starting address") u16 4680 ("starting address") u16 4638 ("starting address")] -> w1690
                        frame "低量程", Default {
                        }
                        frame "高量程" {
                        }
                        frame "0-2量程" {
                        }
                      }
                    }
                    frame 6 {
                      n934 = local read "量程选择"() -> (w1694:enum16{"低量程", "高量程", "0-2量程"})
                      n935 = case shown="\"低量程\", 默认" w1694 {
                        tunnel: [u16 4686 ("starting address") u16 4692 ("starting address") u16 4638 ("starting address")] -> w1695
                        frame "低量程", Default {
                        }
                        frame "高量程" {
                        }
                        frame "0-2量程" {
                        }
                      }
                    }
                    frame 7 {
                      n936 = local read "量程选择"() -> (w1699:enum16{"低量程", "高量程", "0-2量程"})
                      n937 = case shown="\"低量程\", 默认" w1699 {
                        tunnel: [u16 4698 ("starting address") u16 4704 ("starting address") u16 4638 ("starting address")] -> w1700
                        frame "低量程", Default {
                        }
                        frame "高量程" {
                        }
                        frame "0-2量程" {
                        }
                      }
                    }
                  }
                  n938 = Build Array(w1664, w1665, 0.0 ("元素")) -> (w1666:dbl[])
                  n939 = call "浮点转CDAB整形cod.vi"("浮点数"=w1666) -> ("CDAB整形输出"=w1663:u16[])  [unwired: 10 in]
                  n940 = Insert Into Array(array=u16[] [], index=0 ("索引"), new element=w1663) -> (w1656:u16[])
                  n941 = call "CODMnMB_api.vi"("STEP"=enum16{"open", "read", "write", "close"}."write", "values"=w1656, "starting address"=w1657) -> ("error out"=w1655:errorcluster)  [unwired: 6 in, 2 out]
                }
              }
              frame "多项式" {
                # "b,k,c"
                n942 = property on="测量模式(公式)" class="Ring (严格)"() -> ("NumItems"=w1705:u32)  [unwired: 2 in, 2 out]
                n943 = for {
                  N: w1705 -> [_]
                  tunnel: [w1706] -> w1704
                  i -> [w1711]
                  n944 = Increment(x=w1711) -> (x+1=w1710:i32)
                  n945 = local read "多项式系数"() -> (w1715:dbl[])
                  n946 = case shown="2" w1710 {
                    tunnel: [u16 4626 ("starting address") w1722 w1727 w1732 w1737 w1742 w1747 w1752] -> w1707
                    frame 0, Default {
                    }
                    frame 1 {
                      n947 = local read "量程选择"() -> (w1721:enum16{"低量程", "高量程", "0-2量程"})
                      n948 = case shown="\"低量程\", 默认" w1721 {
                        tunnel: [u16 4626 ("starting address") u16 4632 ("starting address") u16 4638 ("starting address")] -> w1722
                        frame "低量程", Default {
                        }
                        frame "高量程" {
                        }
                        frame "0-2量程" {
                        }
                      }
                    }
                    frame 2 {
                      n949 = local read "量程选择"() -> (w1726:enum16{"低量程", "高量程", "0-2量程"})
                      n950 = case shown="\"低量程\", 默认" w1726 {
                        tunnel: [u16 4638 ("starting address") u16 4644 ("starting address") u16 4638 ("starting address")] -> w1727
                        frame "低量程", Default {
                        }
                        frame "高量程" {
                        }
                        frame "0-2量程" {
                        }
                      }
                    }
                    frame 3 {
                      n951 = local read "量程选择"() -> (w1731:enum16{"低量程", "高量程", "0-2量程"})
                      n952 = case shown="\"低量程\", 默认" w1731 {
                        tunnel: [u16 4650 ("starting address") u16 4656 ("starting address") u16 4638 ("starting address")] -> w1732
                        frame "低量程", Default {
                        }
                        frame "高量程" {
                        }
                        frame "0-2量程" {
                        }
                      }
                    }
                    frame 4 {
                      n953 = local read "量程选择"() -> (w1736:enum16{"低量程", "高量程", "0-2量程"})
                      n954 = case shown="\"低量程\", 默认" w1736 {
                        tunnel: [u16 4662 ("starting address") u16 4668 ("starting address") u16 4638 ("starting address")] -> w1737
                        frame "低量程", Default {
                        }
                        frame "高量程" {
                        }
                        frame "0-2量程" {
                        }
                      }
                    }
                    frame 5 {
                      n955 = local read "量程选择"() -> (w1741:enum16{"低量程", "高量程", "0-2量程"})
                      n956 = case shown="\"低量程\", 默认" w1741 {
                        tunnel: [u16 4674 ("starting address") u16 4680 ("starting address") u16 4638 ("starting address")] -> w1742
                        frame "低量程", Default {
                        }
                        frame "高量程" {
                        }
                        frame "0-2量程" {
                        }
                      }
                    }
                    frame 6 {
                      n957 = local read "量程选择"() -> (w1746:enum16{"低量程", "高量程", "0-2量程"})
                      n958 = case shown="\"低量程\", 默认" w1746 {
                        tunnel: [u16 4686 ("starting address") u16 4692 ("starting address") u16 4638 ("starting address")] -> w1747
                        frame "低量程", Default {
                        }
                        frame "高量程" {
                        }
                        frame "0-2量程" {
                        }
                      }
                    }
                    frame 7 {
                      n959 = local read "量程选择"() -> (w1751:enum16{"低量程", "高量程", "0-2量程"})
                      n960 = case shown="\"低量程\", 默认" w1751 {
                        tunnel: [u16 4698 ("starting address") u16 4704 ("starting address") u16 4638 ("starting address")] -> w1752
                        frame "低量程", Default {
                        }
                        frame "高量程" {
                        }
                        frame "0-2量程" {
                        }
                      }
                    }
                  }
                  n961 = Index Array(array=w1715) -> (element #1=w1718:dbl, element #2=w1717:dbl, element #3=w1719:dbl)  [unwired: 3 in]
                  n962 = Build Array(w1717, w1718, w1719) -> (w1716:dbl[])
                  n963 = call "浮点转CDAB整形cod.vi"("浮点数"=w1716) -> ("CDAB整形输出"=w1714:u16[])  [unwired: 10 in]
                  n964 = Insert Into Array(array=u16[] [], index=0 ("索引"), new element=w1714) -> (w1708:u16[])
                  n965 = call "CODMnMB_api.vi"("STEP"=enum16{"open", "read", "write", "close"}."write", "values"=w1708, "starting address"=w1707) -> ("error out"=w1706:errorcluster)  [unwired: 6 in, 2 out]
                }
              }
            }
            n966 = case shown="无错误" w1620 {
              tunnel: ["写入成功！" "写入失败！"] -> w1621
              frame No Error {
                n967 = local read "多项式系数"() -> (w1628:dbl[])
                n968 = Index Array(array=w1628) -> (element #1=w1625:dbl, element #2=w1624:dbl, element #3=w1623:dbl)  [unwired: 3 in]
                n969 = Number To Fractional String(number=w1625) -> (F-format string=w1631:string)  [unwired: 3 in]
                n970 = Number To Fractional String(number=w1624) -> (F-format string=w1632:string)  [unwired: 3 in]
                n971 = Number To Fractional String(number=w1623) -> (F-format string=w1630:string)  [unwired: 3 in]
                n972 = property on="模型" class="Enum (严格)"() -> ("RingText.Text"=w1641:string)  [unwired: 2 in, 2 out]
                n973 = property on="量程选择" class="Enum (严格)"() -> ("RingText.Text"=w1640:string)  [unwired: 2 in, 2 out]
                n974 = Concatenate Strings("变更后:" ("table输入"), "K:" ("字符串"), w1632, "B:" ("字符串"), w1631, "X^2:" ("字符串"), w1630) -> (w1633:string)
                n975 = global read "CODMn断电保存全局变量.vi" "CODMn仪器参数"() -> (w1626:T16)
                n976 = Concatenate Strings(w1641, "【一键写入全部模式】" ("日志信息"), w1640, "公式改变" ("日志信息")) -> (w1634:string)
                n977 = Get Date/Time In Seconds() -> (seconds since 1Jan1904=w1645:timestamp)
                n978 = Bundle By Name(cluster=w1626, "曲线截距"=w1625, "曲线斜率"=w1624, "二次多项式系数"=w1623) -> (w1627:T16)
                n979 = Bundle(cluster=T15 {"时间标识"=timestamp(0 s since 1904-01-01), "参数"="", "日志信息"="", "流程参数"=""} ("data in"), "时间标识"=w1645, "参数"="CODMn" ("table输入"), "日志信息"=w1634, "流程参数"=w1633) -> (w1643:T15)
                n980 = global write "CODMn断电保存全局变量.vi" "CODMn仪器参数"(w1627) -> ()
                n981 = call "流程日志字段定义.vi"("table输入"="操作日志", "data in"=w1643) -> ("table输出"=w1648:string, "columns"=w1649:string[], "data out"=w1650:T19)  [unwired: 7 in]
                n982 = call "插入数据.vi"("data"=w1650, "columns"=w1649, "database"="database3.mdb", "table"=w1648) -> ()  [unwired: 7 in, 1 out]
              }
              frame Error {
              }
            }
            n983 = One Button Dialog(message=w1621) -> ()  [unwired: 1 in, 1 out]
          }
          frame "Right Button" {
          }
          frame "Window Close" {
          }
        }
      }
      event "一键写入": Value Change {
        n984 = event-data() -> ()  [unwired: 1 in, 6 out]
        n985 = Two Button Dialog(message="确认是否写入公式，写入会覆盖原有公式！" ("消息")) -> (T button?=w1756:bool)  [unwired: 2 in]
        n986 = case shown="真" w1756 {
          frame False {
          }
          frame True {
            n987 = local read "模型"() -> (w1760:enum32{"线性", "多项式"})
            n988 = case shown="\"线性\", 默认" w1760 {
              tunnel: [w1791 w1842] -> w1758
              frame "线性", Default {
                n989 = property on="测量模式(公式)" class="Ring (严格)"() -> ("NumItems"=w1792:u32)  [unwired: 2 in, 2 out]
                n990 = for {
                  N: w1792 -> [_]
                  tunnel: [w1793] -> w1791
                  i -> [w1798]
                  n991 = Increment(x=w1798) -> (x+1=w1797:i32)
                  n992 = local read "K"() -> (w1802:dbl)
                  n993 = local read "b"() -> (w1803:dbl)
                  n994 = case shown="1" w1797 {
                    tunnel: [u16 4626 ("starting address") w1808 w1813 w1818 w1823 w1828 w1833 w1838] -> w1795
                    frame 0, Default {
                    }
                    frame 1 {
                      n995 = local read "量程选择"() -> (w1807:enum16{"低量程", "高量程", "0-2量程"})
                      n996 = case shown="\"低量程\", 默认" w1807 {
                        tunnel: [u16 4626 ("starting address") u16 4632 ("starting address") u16 4638 ("starting address")] -> w1808
                        frame "低量程", Default {
                        }
                        frame "高量程" {
                        }
                        frame "0-2量程" {
                        }
                      }
                    }
                    frame 2 {
                      n997 = local read "量程选择"() -> (w1812:enum16{"低量程", "高量程", "0-2量程"})
                      n998 = case shown="\"低量程\", 默认" w1812 {
                        tunnel: [u16 4638 ("starting address") u16 4644 ("starting address") u16 4638 ("starting address")] -> w1813
                        frame "低量程", Default {
                        }
                        frame "高量程" {
                        }
                        frame "0-2量程" {
                        }
                      }
                    }
                    frame 3 {
                      n999 = local read "量程选择"() -> (w1817:enum16{"低量程", "高量程", "0-2量程"})
                      n1000 = case shown="\"低量程\", 默认" w1817 {
                        tunnel: [u16 4650 ("starting address") u16 4656 ("starting address") u16 4638 ("starting address")] -> w1818
                        frame "低量程", Default {
                        }
                        frame "高量程" {
                        }
                        frame "0-2量程" {
                        }
                      }
                    }
                    frame 4 {
                      n1001 = local read "量程选择"() -> (w1822:enum16{"低量程", "高量程", "0-2量程"})
                      n1002 = case shown="\"高量程\"" w1822 {
                        tunnel: [u16 4662 ("starting address") u16 4668 ("starting address") u16 4638 ("starting address")] -> w1823
                        frame "低量程", Default {
                        }
                        frame "高量程" {
                        }
                        frame "0-2量程" {
                        }
                      }
                    }
                    frame 5 {
                      n1003 = local read "量程选择"() -> (w1827:enum16{"低量程", "高量程", "0-2量程"})
                      n1004 = case shown="\"低量程\", 默认" w1827 {
                        tunnel: [u16 4674 ("starting address") u16 4680 ("starting address") u16 4638 ("starting address")] -> w1828
                        frame "低量程", Default {
                        }
                        frame "高量程" {
                        }
                        frame "0-2量程" {
                        }
                      }
                    }
                    frame 6 {
                      n1005 = local read "量程选择"() -> (w1832:enum16{"低量程", "高量程", "0-2量程"})
                      n1006 = case shown="\"低量程\", 默认" w1832 {
                        tunnel: [u16 4686 ("starting address") u16 4692 ("starting address") u16 4638 ("starting address")] -> w1833
                        frame "低量程", Default {
                        }
                        frame "高量程" {
                        }
                        frame "0-2量程" {
                        }
                      }
                    }
                    frame 7 {
                      n1007 = local read "量程选择"() -> (w1837:enum16{"低量程", "高量程", "0-2量程"})
                      n1008 = case shown="\"低量程\", 默认" w1837 {
                        tunnel: [u16 4698 ("starting address") u16 4704 ("starting address") u16 4638 ("starting address")] -> w1838
                        frame "低量程", Default {
                        }
                        frame "高量程" {
                        }
                        frame "0-2量程" {
                        }
                      }
                    }
                  }
                  n1009 = Build Array(w1802, w1803, 0.0 ("元素")) -> (w1804:dbl[])
                  n1010 = call "浮点转CDAB整形cod.vi"("浮点数"=w1804) -> ("CDAB整形输出"=w1801:u16[])  [unwired: 10 in]
                  n1011 = Insert Into Array(array=u16[] [], index=0 ("索引"), new element=w1801) -> (w1794:u16[])
                  n1012 = call "CODMnMB_api.vi"("STEP"=enum16{"open", "read", "write", "close"}."write", "values"=w1794, "starting address"=w1795) -> ("error out"=w1793:errorcluster)  [unwired: 6 in, 2 out]
                }
              }
              frame "多项式" {
                # "b,k,c"
                n1013 = property on="测量模式(公式)" class="Ring (严格)"() -> ("NumItems"=w1843:u32)  [unwired: 2 in, 2 out]
                n1014 = for {
                  N: w1843 -> [_]
                  tunnel: [w1844] -> w1842
                  i -> [w1849]
                  n1015 = Increment(x=w1849) -> (x+1=w1848:i32)
                  n1016 = local read "多项式系数"() -> (w1853:dbl[])
                  n1017 = case shown="2" w1848 {
                    tunnel: [u16 4626 ("starting address") w1860 w1865 w1870 w1875 w1880 w1885 w1890] -> w1845
                    frame 0, Default {
                    }
                    frame 1 {
                      n1018 = local read "量程选择"() -> (w1859:enum16{"低量程", "高量程", "0-2量程"})
                      n1019 = case shown="\"低量程\", 默认" w1859 {
                        tunnel: [u16 4626 ("starting address") u16 4632 ("starting address") u16 4638 ("starting address")] -> w1860
                        frame "低量程", Default {
                        }
                        frame "高量程" {
                        }
                        frame "0-2量程" {
                        }
                      }
                    }
                    frame 2 {
                      n1020 = local read "量程选择"() -> (w1864:enum16{"低量程", "高量程", "0-2量程"})
                      n1021 = case shown="\"低量程\", 默认" w1864 {
                        tunnel: [u16 4638 ("starting address") u16 4644 ("starting address") u16 4638 ("starting address")] -> w1865
                        frame "低量程", Default {
                        }
                        frame "高量程" {
                        }
                        frame "0-2量程" {
                        }
                      }
                    }
                    frame 3 {
                      n1022 = local read "量程选择"() -> (w1869:enum16{"低量程", "高量程", "0-2量程"})
                      n1023 = case shown="\"低量程\", 默认" w1869 {
                        tunnel: [u16 4650 ("starting address") u16 4656 ("starting address") u16 4638 ("starting address")] -> w1870
                        frame "低量程", Default {
                        }
                        frame "高量程" {
                        }
                        frame "0-2量程" {
                        }
                      }
                    }
                    frame 4 {
                      n1024 = local read "量程选择"() -> (w1874:enum16{"低量程", "高量程", "0-2量程"})
                      n1025 = case shown="\"低量程\", 默认" w1874 {
                        tunnel: [u16 4662 ("starting address") u16 4668 ("starting address") u16 4638 ("starting address")] -> w1875
                        frame "低量程", Default {
                        }
                        frame "高量程" {
                        }
                        frame "0-2量程" {
                        }
                      }
                    }
                    frame 5 {
                      n1026 = local read "量程选择"() -> (w1879:enum16{"低量程", "高量程", "0-2量程"})
                      n1027 = case shown="\"低量程\", 默认" w1879 {
                        tunnel: [u16 4674 ("starting address") u16 4680 ("starting address") u16 4638 ("starting address")] -> w1880
                        frame "低量程", Default {
                        }
                        frame "高量程" {
                        }
                        frame "0-2量程" {
                        }
                      }
                    }
                    frame 6 {
                      n1028 = local read "量程选择"() -> (w1884:enum16{"低量程", "高量程", "0-2量程"})
                      n1029 = case shown="\"低量程\", 默认" w1884 {
                        tunnel: [u16 4686 ("starting address") u16 4692 ("starting address") u16 4638 ("starting address")] -> w1885
                        frame "低量程", Default {
                        }
                        frame "高量程" {
                        }
                        frame "0-2量程" {
                        }
                      }
                    }
                    frame 7 {
                      n1030 = local read "量程选择"() -> (w1889:enum16{"低量程", "高量程", "0-2量程"})
                      n1031 = case shown="\"低量程\", 默认" w1889 {
                        tunnel: [u16 4698 ("starting address") u16 4704 ("starting address") u16 4638 ("starting address")] -> w1890
                        frame "低量程", Default {
                        }
                        frame "高量程" {
                        }
                        frame "0-2量程" {
                        }
                      }
                    }
                  }
                  n1032 = Index Array(array=w1853) -> (element #1=w1856:dbl, element #2=w1855:dbl, element #3=w1857:dbl)  [unwired: 3 in]
                  n1033 = Build Array(w1855, w1856, w1857) -> (w1854:dbl[])
                  n1034 = call "浮点转CDAB整形cod.vi"("浮点数"=w1854) -> ("CDAB整形输出"=w1852:u16[])  [unwired: 10 in]
                  n1035 = Insert Into Array(array=u16[] [], index=0 ("索引"), new element=w1852) -> (w1846:u16[])
                  n1036 = call "CODMnMB_api.vi"("STEP"=enum16{"open", "read", "write", "close"}."write", "values"=w1846, "starting address"=w1845) -> ("error out"=w1844:errorcluster)  [unwired: 6 in, 2 out]
                }
              }
            }
            n1037 = case shown="无错误" w1758 {
              tunnel: ["写入成功！" "写入失败！"] -> w1759
              frame No Error {
                n1038 = local read "多项式系数"() -> (w1766:dbl[])
                n1039 = Index Array(array=w1766) -> (element #1=w1763:dbl, element #2=w1762:dbl, element #3=w1761:dbl)  [unwired: 3 in]
                n1040 = Number To Fractional String(number=w1763) -> (F-format string=w1769:string)  [unwired: 3 in]
                n1041 = Number To Fractional String(number=w1762) -> (F-format string=w1770:string)  [unwired: 3 in]
                n1042 = Number To Fractional String(number=w1761) -> (F-format string=w1768:string)  [unwired: 3 in]
                n1043 = property on="模型" class="Enum (严格)"() -> ("RingText.Text"=w1779:string)  [unwired: 2 in, 2 out]
                n1044 = property on="量程选择" class="Enum (严格)"() -> ("RingText.Text"=w1778:string)  [unwired: 2 in, 2 out]
                n1045 = Concatenate Strings("变更后:" ("table输入"), "K:" ("字符串"), w1770, "B:" ("字符串"), w1769, "X^2:" ("字符串"), w1768) -> (w1771:string)
                n1046 = global read "CODMn断电保存全局变量.vi" "CODMn仪器参数"() -> (w1764:T16)
                n1047 = Concatenate Strings(w1779, "【一键写入全部模式】" ("日志信息"), w1778, "公式改变" ("日志信息")) -> (w1772:string)
                n1048 = Get Date/Time In Seconds() -> (seconds since 1Jan1904=w1783:timestamp)
                n1049 = Bundle By Name(cluster=w1764, "曲线截距"=w1763, "曲线斜率"=w1762, "二次多项式系数"=w1761) -> (w1765:T16)
                n1050 = Bundle(cluster=T15 {"时间标识"=timestamp(0 s since 1904-01-01), "参数"="", "日志信息"="", "流程参数"=""} ("data in"), "时间标识"=w1783, "参数"="CODMn" ("table输入"), "日志信息"=w1772, "流程参数"=w1771) -> (w1781:T15)
                n1051 = global write "CODMn断电保存全局变量.vi" "CODMn仪器参数"(w1765) -> ()
                n1052 = call "流程日志字段定义.vi"("table输入"="操作日志", "data in"=w1781) -> ("table输出"=w1786:string, "columns"=w1787:string[], "data out"=w1788:T19)  [unwired: 7 in]
                n1053 = call "插入数据.vi"("data"=w1788, "columns"=w1787, "database"="database3.mdb", "table"=w1786) -> ()  [unwired: 7 in, 1 out]
              }
              frame Error {
              }
            }
            n1054 = One Button Dialog(message=w1759) -> ()  [unwired: 1 in, 1 out]
          }
        }
      }
      event "滴定曲线", "温度曲线": Value Change {
        n1055 = event-data() -> ("CtlRef"=w1895:refnum<vi>)  [unwired: 1 in, 5 out]
        n1056 = property class="Bool"(reference=w1895) -> ("Label.Text"=w1894:string)  [unwired: 1 in, 2 out]
        n1057 = case shown="\"温度曲线\", 默认" w1894 {
          tunnel: [T4 {"Horizontal"=0, "Vertical"=4000} ("原点") T4 {"Horizontal"=0, "Vertical"=3200} ("原点")] -> w1896
          frame "温度曲线", Default {
          }
          frame "滴定曲线" {
          }
        }
        n1058 = property on="窗格" class="Pane"("Origin"=w1896) -> ()  [unwired: 2 in, 2 out]
      }
      event "历史波形", "历史波形 2": Value Change {
        n1059 = event-data() -> ("CtlRef"=w1900:refnum<vi>)  [unwired: 1 in, 5 out]
        n1060 = property class="Bool (严格)"(reference=w1900) -> ("Label.Text"=w1899:string)  [unwired: 1 in, 2 out]
        n1061 = case shown="\"历史波形2\"" w1899 {
          frame "历史波形2" {
            n1062 = call-poly <vilib>:"Read Waveforms from File.vi"() -> ("error out"=w1901:errorcluster, "first waveform in record"=w1902:waveform(dbl))  [unwired: 6 in, 2 out]
            n1063 = case shown="无错误" w1901 {
              tunnel: w1902 -> [w1905 _]
              frame No Error {
                n1064 = Unbundle By Name(w1905) -> ("t0"=w1903:timestamp, "Y"=w1904:dbl[])  [unwired: 2 out]
                n1065 = global write "COD内部交互全局.vi" "温度波形时间"(w1903) -> ()
                n1066 = global write "COD内部交互全局.vi" "时间温度曲线"(w1904) -> ()
                n1067 = global write "COD内部交互全局.vi" "时间-温度"(w1904) -> ()
              }
              frame Error {
                n1068 = One Button Dialog(message="打开失败" ("消息")) -> ()  [unwired: 1 in, 1 out]
              }
            }
          }
          frame "历史波形", Default {
            n1069 = call-poly <vilib>:"Read Waveforms from File.vi"() -> ("error out"=w1907:errorcluster, "first waveform in record"=w1908:waveform(dbl))  [unwired: 6 in, 2 out]
            n1070 = case shown="无错误" w1907 {
              tunnel: w1908 -> [w1911 _]
              frame No Error {
                n1071 = Unbundle By Name(w1911) -> ("t0"=w1909:timestamp, "Y"=w1910:dbl[])  [unwired: 2 out]
                n1072 = global write "COD内部交互全局.vi" "波形时间"(w1909) -> ()
                n1073 = global write "COD内部交互全局.vi" "ORP滴定曲线"(w1910) -> ()
                n1074 = global write "COD内部交互全局.vi" "滴定数-ORP值"(w1910) -> ()
              }
              frame Error {
                n1075 = One Button Dialog(message="打开失败" ("消息")) -> ()  [unwired: 1 in, 1 out]
              }
            }
          }
        }
      }
      event "释放串口": Value Change {
        n1076 = event-data() -> ()  [unwired: 1 in, 6 out]
        n1077 = Two Button Dialog(message="确认是否释放串口，释放串口将导致通信失败！" ("消息")) -> (T button?=w1913:bool)  [unwired: 2 in]
        n1078 = case shown="真" w1913 {
          tunnel: w1916 -> [_ w1918]
          tunnel: w1915 -> [_ w1917]
          frame False {
          }
          frame True {
            n1079 = Bundle By Name(cluster=cluster{"命令":string} {"命令"=""} ("元素"), "命令"="停用模块" ("名称（未命名）")) -> (w1919:cluster{"命令":string})
            n1080 = Enqueue Element(queue=w1918, element=w1919, error in (no error)=w1917) -> ()  [unwired: 1 in, 3 out]
          }
        }
      }
      event "打开串口": Value Change {
        n1081 = event-data() -> ()  [unwired: 1 in, 6 out]
        n1082 = flat-sequence {
          tunnel: w1923 -> [w1931]
          tunnel: w1922 -> [w1930]
          frame #0 {
            n1083 = global read "CODMn断电保存全局变量.vi" "VISA resource name"() -> (w1934:refnum<visa-resource-name>)
            n1084 = global read "CODMn断电保存全局变量.vi" "MB通信方式选择"() -> (w1927:enum16{"串口", "TCP"})
            n1085 = global read "CODMn断电保存全局变量.vi" "PORT"() -> (w1925:string)
            n1086 = global read "CODMn断电保存全局变量.vi" "IP"() -> (w1926:string)
            n1087 = call "串口配置.vi"("PORT"=w1925, "IP"=w1926, "MB通信方式选择"=w1927, "请选择串口:"=w1934) -> ("PORT 2"=w1928:string, "IP 2"=w1929:string, "确认 2"=w1932:bool, "VISA资源名称 2"=w1933:refnum<visa-resource-name>, "MB通信方式选择 2"=w1924:enum16{"串口", "TCP"})  [unwired: 3 in]
            n1088 = case shown="真" w1932 {
              tunnel: w1933 -> [_ w1943]
              tunnel: w1931 -> [_ w1939]
              tunnel: w1930 -> [_ w1938]
              tunnel: w1929 -> [_ w1937]
              tunnel: w1928 -> [_ w1936]
              tunnel: w1924 -> [_ w1935]
              frame False {
              }
              frame True {
                n1089 = global write "CODMn断电保存全局变量.vi" "IP"(w1937) -> ()
                n1090 = global write "CODMn断电保存全局变量.vi" "PORT"(w1936) -> ()
                n1091 = global write "CODMn断电保存全局变量.vi" "VISA resource name"(w1943) -> ()
                n1092 = global write "CODMn断电保存全局变量.vi" "MB通信方式选择"(w1935) -> ()
                n1093 = Bundle By Name(cluster=cluster{"命令":string} {"命令"=""} ("元素"), "命令"="启用模块" ("名称（未命名）")) -> (w1940:cluster{"命令":string})
                n1094 = Enqueue Element(queue=w1939, element=w1940, error in (no error)=w1938) -> ()  [unwired: 1 in, 3 out]
              }
            }
          }
          frame #1 {
            n1095 = call "配置文件保存.vi"() -> ()  [unwired: 12 in]
          }
        }
      }
      event "更新程序": Value Change {
        n1096 = event-data() -> ("CtlRef"=w1946:refnum<vi>, "NewVal"=w1947:bool)  [unwired: 1 in, 4 out]
        n1097 = case shown="真" w1947 {
          tunnel: w1946 -> [_ w1956]
          tunnel: w1945 -> [w1949 w1955]
          tunnel: w1944 -> [w1948 w1954]
          frame False {
            n1098 = Bundle By Name(cluster=cluster{"命令":string} {"命令"=""} ("元素"), "命令"="启用模块" ("名称（未命名）")) -> (w1950:cluster{"命令":string})
            n1099 = Enqueue Element(queue=w1949, element=w1950, error in (no error)=w1948) -> ()  [unwired: 1 in, 3 out]
          }
          frame True {
            n1100 = Two Button Dialog(message="警告，非专业人士请勿进行此操作！！！\n请确认是否继续？" ("消息")) -> (T button?=w1958:bool)  [unwired: 2 in]
            n1101 = case shown="真" w1958 {
              tunnel: w1956 -> [w1974 _]
              tunnel: w1955 -> [_ w1982]
              tunnel: w1954 -> [_ w1981]
              tunnel: [errorcluster {"status"=TRUE, "code"=0, "source"=""} ("error out") w1975] -> w1953
              frame False {
                n1102 = property class="Bool (严格)"(reference=w1974, "Value"=FALSE ("释放串口")) -> ()  [unwired: 1 in, 2 out]
              }
              frame True {
                n1103 = Bundle By Name(cluster=cluster{"命令":string} {"命令"=""} ("元素"), "命令"="CODMn程序更新" ("名称（未命名）")) -> (w1985:cluster{"命令":string})
                n1104 = Enqueue Element(queue=w1982, element=w1985, error in (no error)=w1981) -> (queue out=w1980:refnum<queue>, error out=w1979:errorcluster)  [unwired: 1 in, 1 out]
                n1105 = Bundle By Name(cluster=cluster{"命令":string} {"命令"=""} ("元素"), "命令"="停用模块" ("名称（未命名）")) -> (w1976:cluster{"命令":string})
                n1106 = Enqueue Element(queue=w1980, element=w1976, error in (no error)=w1979) -> (error out=w1975:errorcluster)  [unwired: 1 in, 2 out]
              }
            }
            n1107 = case shown="无错误" w1953 {
              frame No Error {
                n1108 = call "文件对话框"("start path"=path "D:/SRC") -> ("selected path"=w1961:path, "cancelled"=w1959:bool)  [unwired: 11 in, 2 out]
                n1109 = case shown="假" w1959 {
                  tunnel: w1961 -> [w1966 _]
                  frame False {
                    n1110 = Path To String(path=w1966) -> (string=w1963:string)
                    n1111 = Format Into String(format string="  - \"%s\"" ("格式字符串"), initial string="\"C:\\Program Files\\Fatek\\WinProladder\\WProlad.exe\"" ("command line"), w1963) -> (resulting string=w1964:string)  [unwired: 1 in, 1 out]
                    n1112 = call <vilib>:"System Exec.vi"("command line"=w1964) -> ("error out"=w1967:errorcluster)  [unwired: 7 in, 3 out]
                    n1113 = case shown="错误" w1967 {
                      tunnel: w1963 -> [_ w1970]
                      frame No Error {
                      }
                      frame Error {
                        n1114 = Format Into String(format string="  - \"%s\"" ("格式字符串"), initial string="\"C:\\Program Files (x86)\\Fatek\\WinProladder\\WProlad.exe\"" ("command line"), w1970) -> (resulting string=w1968:string)  [unwired: 1 in, 1 out]
                        n1115 = call <vilib>:"System Exec.vi"("command line"=w1968) -> ()  [unwired: 7 in, 4 out]
                      }
                    }
                  }
                  frame True {
                  }
                }
              }
              frame Error {
              }
            }
          }
        }
      }
      event "序列号变更": Value Change {
        n1116 = event-data() -> ()  [unwired: 1 in, 6 out]
        n1117 = local read "CODMn序列号"() -> (w1989:string)
        n1118 = call "序列号写入.vi"("序列号:"=w1989) -> ("确认 2"=w1986:bool, "序列号输出"=w1990:string)  [unwired: 9 in]
        n1119 = case shown="真" w1986 {
          tunnel: w1990 -> [_ w1996]
          tunnel: w1988 -> [_ w1992]
          tunnel: w1987 -> [_ w1991]
          frame False {
          }
          frame True {
            n1120 = global write "COD内部交互全局.vi" "序列号:"(w1996) -> ()
            n1121 = Bundle By Name(cluster=cluster{"命令":string} {"命令"=""} ("元素"), "命令"="CODMn序列号写入" ("名称（未命名）")) -> (w1993:cluster{"命令":string})
            n1122 = Enqueue Element(queue=w1992, element=w1993, error in (no error)=w1991) -> ()  [unwired: 1 in, 3 out]
          }
        }
      }
      event Timeout {
        n1123 = event-data() -> ()  [unwired: 1 in, 3 out]
      }
    }
  }
  n1124 = while {
    stop <- FALSE stop-if-true
    n1125 = global read "COD内部交互全局.vi" "待机"() -> (w1998:bool)
    n1126 = Wait (ms)(milliseconds to wait=u32 1000 ("等待时间（毫秒）")) -> ()  [unwired: 1 out]
    n1127 = case shown="假" w1998 {
      tunnel: [w2015 T9."Enabled" ("禁用")] -> w2000
      tunnel: [w2014 _] -> w1999
      frame False {
        # "运行中"
        n1128 = local read "校标标记"() -> (w2013:bool)
        n1129 = local read "校零标记"() -> (w2012:bool)
        n1130 = Or(x=w2013, y=w2012) -> (x .or. y?=w2016:bool)
        n1131 = case shown="真" w2016 {
          tunnel: [T9."Enabled" ("禁用") T9."Disabled and Grayed Out" ("禁用")] -> w2015
          tunnel: [_ TRUE] -> w2014
          frame False {
          }
          frame True {
          }
        }
      }
      frame True {
      }
    }
    n1132 = control-ref of="量程选择"() -> (w2006:refnum<vi>)
    n1133 = property on="校准内容显示" class="Str"("Visible"=w1999) -> ()  [unwired: 2 in, 2 out]
    n1134 = control-ref of="选用水样"() -> (w2007:refnum<vi>)
    n1135 = control-ref of="校准5"() -> (w2001:refnum<vi>)
    n1136 = control-ref of="校准4"() -> (w2002:refnum<vi>)
    n1137 = control-ref of="校准3"() -> (w2003:refnum<vi>)
    n1138 = control-ref of="校准2"() -> (w2004:refnum<vi>)
    n1139 = control-ref of="校准1"() -> (w2005:refnum<vi>)
    n1140 = Build Array(w2001, w2002, w2003, w2004, w2005, w2007, w2006) -> (w2008:refnum<vi>[])
    n1141 = for {
      tunnel: w2008 -> [w2011] mode=indexing
      tunnel: w2000 -> [w2010]
      n1142 = property class="Ctl"(reference=w2011, "DisabledEnum"=w2010) -> ()  [unwired: 1 in, 2 out]
    }
  }
  n1143 = while {
    stop <- FALSE stop-if-true
    # "数字键盘输入"
    n1144 = event shown="[23] \"泵滴定数1\": 鼠标按下" {
      selector: _ -> [_ _ _ _ _ _ _ _ _ _ _ _ _ _ _ _ _ _ _ _ _ _ _ _ _ _ _ _ _ _]
      dyn-events: _ -> [_ _ _ _ _ _ _ _ _ _ _ _ _ _ _ _ _ _ _ _ _ _ _ _ _ _ _ _ _ _]
      timeout: _ -> [_ _ _ _ _ _ _ _ _ _ _ _ _ _ _ _ _ _ _ _ _ _ _ _ _ _ _ _ _ _]
      event Timeout {
        n1145 = event-data() -> ()  [unwired: 1 in, 3 out]
      }
      event "温度": Mouse Down {
        n1146 = event-data() -> ()  [unwired: 1 in, 8 out]
        n1147 = local read "温度"() -> (w2023:dbl)
        n1148 = call "数字键盘.vi"("OldNumber"=w2023) -> ("NewNumber"=w2022:sgl)
        n1149 = local write "温度"(w2022) -> ()
      }
      event "恒温时间": Mouse Down {
        n1150 = event-data() -> ()  [unwired: 1 in, 8 out]
        n1151 = local read "恒温时间"() -> (w2024:dbl)
        n1152 = call "数字键盘.vi"("OldNumber"=w2024) -> ("NewNumber"=w2025:sgl)
        n1153 = local write "恒温时间"(w2025) -> ()
      }
      event "标准液浓度": Mouse Down {
        n1154 = event-data() -> ()  [unwired: 1 in, 8 out]
        n1155 = local read "标准液浓度"() -> (w2027:dbl)
        n1156 = call "数字键盘.vi"("OldNumber"=w2027) -> ("NewNumber"=w2026:sgl)
        n1157 = local write "标准液浓度"(w2026) -> ()
      }
      event "氢氧化钠：": Mouse Down {
        n1158 = event-data() -> ()  [unwired: 1 in, 8 out]
        n1159 = local read "氢氧化钠："() -> (w2028:dbl)
        n1160 = call "数字键盘.vi"("OldNumber"=w2028) -> ("NewNumber"=w2029:sgl)
        n1161 = local write "氢氧化钠："(w2029) -> ()
      }
      event "水样：": Mouse Down {
        n1162 = event-data() -> ()  [unwired: 1 in, 8 out]
        n1163 = local read "水样："() -> (w2030:dbl)
        n1164 = call "数字键盘.vi"("OldNumber"=w2030) -> ("NewNumber"=w2031:sgl)
        n1165 = local write "水样："(w2031) -> ()
      }
      event "蒸馏水：": Mouse Down {
        n1166 = event-data() -> ()  [unwired: 1 in, 8 out]
        n1167 = local read "蒸馏水："() -> (w2032:dbl)
        n1168 = call "数字键盘.vi"("OldNumber"=w2032) -> ("NewNumber"=w2033:sgl)
        n1169 = local write "蒸馏水："(w2033) -> ()
      }
      event "标液：": Mouse Down {
        n1170 = event-data() -> ()  [unwired: 1 in, 8 out]
        n1171 = local read "标液："() -> (w2034:dbl)
        n1172 = call "数字键盘.vi"("OldNumber"=w2034) -> ("NewNumber"=w2035:sgl)
        n1173 = local write "标液："(w2035) -> ()
      }
      event "零点核查样：": Mouse Down {
        n1174 = event-data() -> ()  [unwired: 1 in, 8 out]
        n1175 = local read "零点核查样："() -> (w2036:dbl)
        n1176 = call "数字键盘.vi"("OldNumber"=w2036) -> ("NewNumber"=w2037:sgl)
        n1177 = local write "零点核查样："(w2037) -> ()
      }
      event "加标回收样：": Mouse Down {
        n1178 = event-data() -> ()  [unwired: 1 in, 8 out]
        n1179 = local read "加标回收样："() -> (w2038:dbl)
        n1180 = call "数字键盘.vi"("OldNumber"=w2038) -> ("NewNumber"=w2039:sgl)
        n1181 = local write "加标回收样："(w2039) -> ()
      }
      event "草酸钠": Mouse Down {
        n1182 = event-data() -> ()  [unwired: 1 in, 8 out]
        n1183 = local read "草酸钠"() -> (w2040:dbl)
        n1184 = call "数字键盘.vi"("OldNumber"=w2040) -> ("NewNumber"=w2041:sgl)
        n1185 = local write "草酸钠"(w2041) -> ()
      }
      event "高锰酸钾": Mouse Down {
        n1186 = event-data() -> ()  [unwired: 1 in, 8 out]
        n1187 = local read "高锰酸钾"() -> (w2042:dbl)
        n1188 = call "数字键盘.vi"("OldNumber"=w2042) -> ("NewNumber"=w2043:sgl)
        n1189 = local write "高锰酸钾"(w2043) -> ()
      }
      event "硫酸": Mouse Down {
        n1190 = event-data() -> ()  [unwired: 1 in, 8 out]
        n1191 = local read "硫酸"() -> (w2044:dbl)
        n1192 = call "数字键盘.vi"("OldNumber"=w2044) -> ("NewNumber"=w2045:sgl)
        n1193 = local write "硫酸"(w2045) -> ()
      }
      event "零点泵计量数 2": Mouse Down {
        n1194 = event-data() -> ()  [unwired: 1 in, 8 out]
        n1195 = local read "零点泵计量数 2"() -> (w2046:dbl)
        n1196 = call "数字键盘.vi"("OldNumber"=w2046) -> ("NewNumber"=w2047:sgl)
        n1197 = local write "零点泵计量数 2"(w2047) -> ()
      }
      event "标度泵计量数 2": Mouse Down {
        n1198 = event-data() -> ()  [unwired: 1 in, 8 out]
        n1199 = local read "标度泵计量数 2"() -> (w2048:dbl)
        n1200 = call "数字键盘.vi"("OldNumber"=w2048) -> ("NewNumber"=w2049:sgl)
        n1201 = local write "标度泵计量数 2"(w2049) -> ()
      }
      event "高量程稀释倍数:": Mouse Down {
        n1202 = event-data() -> ()  [unwired: 1 in, 8 out]
        n1203 = local read "高量程稀释倍数:"() -> (w2051:i8)
        n1204 = call "数字键盘.vi"("OldNumber"=w2051) -> ("NewNumber"=w2050:sgl)
        n1205 = local write "高量程稀释倍数:"(w2050) -> ()
      }
      event "低量程稀释倍数:": Mouse Down {
        n1206 = event-data() -> ()  [unwired: 1 in, 8 out]
        n1207 = local read "低量程稀释倍数:"() -> (w2053:i8)
        n1208 = call "数字键盘.vi"("OldNumber"=w2053) -> ("NewNumber"=w2052:sgl)
        n1209 = local write "低量程稀释倍数:"(w2052) -> ()
      }
      event "浓度1": Mouse Down {
        n1210 = event-data() -> ()  [unwired: 1 in, 8 out]
        n1211 = local read "浓度1"() -> (w2055:dbl)
        n1212 = call "数字键盘.vi"("OldNumber"=w2055) -> ("NewNumber"=w2054:sgl)
        n1213 = property on="浓度1" class="DigNum (严格)"("Val(Sgnl)"=w2054) -> ()  [unwired: 2 in, 2 out]
      }
      event "浓度2": Mouse Down {
        n1214 = event-data() -> ()  [unwired: 1 in, 8 out]
        n1215 = local read "浓度2"() -> (w2057:dbl)
        n1216 = call "数字键盘.vi"("OldNumber"=w2057) -> ("NewNumber"=w2056:sgl)
        n1217 = property on="浓度2" class="DigNum (严格)"("Val(Sgnl)"=w2056) -> ()  [unwired: 2 in, 2 out]
      }
      event "浓度3": Mouse Down {
        n1218 = event-data() -> ()  [unwired: 1 in, 8 out]
        n1219 = local read "浓度3"() -> (w2059:dbl)
        n1220 = call "数字键盘.vi"("OldNumber"=w2059) -> ("NewNumber"=w2058:sgl)
        n1221 = property on="浓度3" class="DigNum (严格)"("Val(Sgnl)"=w2058) -> ()  [unwired: 2 in, 2 out]
      }
      event "浓度4": Mouse Down {
        n1222 = event-data() -> ()  [unwired: 1 in, 8 out]
        n1223 = local read "浓度4"() -> (w2061:dbl)
        n1224 = call "数字键盘.vi"("OldNumber"=w2061) -> ("NewNumber"=w2060:sgl)
        n1225 = property on="浓度4" class="DigNum (严格)"("Val(Sgnl)"=w2060) -> ()  [unwired: 2 in, 2 out]
      }
      event "浓度5": Mouse Down {
        n1226 = event-data() -> ()  [unwired: 1 in, 8 out]
        n1227 = local read "浓度5"() -> (w2063:dbl)
        n1228 = call "数字键盘.vi"("OldNumber"=w2063) -> ("NewNumber"=w2062:sgl)
        n1229 = property on="浓度5" class="DigNum (严格)"("Val(Sgnl)"=w2062) -> ()  [unwired: 2 in, 2 out]
      }
      event "跨度液浓度", "零点核查浓度", "标样浓度": Mouse Down {
        n1230 = event-data() -> ("CtlRef"=w2067:refnum<vi>)  [unwired: 1 in, 7 out]
        n1231 = property class="DigNum (严格)"(reference=w2067) -> (reference out=w2064:refnum<vi>, "Value"=w2066:dbl)  [unwired: 1 in, 1 out]
        n1232 = call "数字键盘.vi"("OldNumber"=w2066) -> ("NewNumber"=w2065:sgl)
        n1233 = property class="DigNum (严格)"(reference=w2064, "Val(Sgnl)"=w2065) -> ()  [unwired: 1 in, 2 out]
      }
      event "泵滴定数1": Mouse Down {
        n1234 = event-data() -> ()  [unwired: 1 in, 8 out]
        n1235 = local read "泵滴定数1"() -> (w2069:dbl)
        n1236 = call "数字键盘.vi"("OldNumber"=w2069) -> ("NewNumber"=w2068:sgl)
        n1237 = property on="泵滴定数1" class="DigNum (严格)"("Val(Sgnl)"=w2068) -> ()  [unwired: 2 in, 2 out]
      }
      event "泵滴定数2": Mouse Down {
        n1238 = event-data() -> ()  [unwired: 1 in, 8 out]
        n1239 = local read "泵滴定数2"() -> (w2071:dbl)
        n1240 = call "数字键盘.vi"("OldNumber"=w2071) -> ("NewNumber"=w2070:sgl)
        n1241 = property on="泵滴定数2" class="DigNum (严格)"("Val(Sgnl)"=w2070) -> ()  [unwired: 2 in, 2 out]
      }
      event "泵滴定数3": Mouse Down {
        n1242 = event-data() -> ()  [unwired: 1 in, 8 out]
        n1243 = local read "泵滴定数3"() -> (w2073:dbl)
        n1244 = call "数字键盘.vi"("OldNumber"=w2073) -> ("NewNumber"=w2072:sgl)
        n1245 = property on="泵滴定数3" class="DigNum (严格)"("Val(Sgnl)"=w2072) -> ()  [unwired: 2 in, 2 out]
      }
      event "泵滴定数4": Mouse Down {
        n1246 = event-data() -> ()  [unwired: 1 in, 8 out]
        n1247 = local read "泵滴定数4"() -> (w2075:dbl)
        n1248 = call "数字键盘.vi"("OldNumber"=w2075) -> ("NewNumber"=w2074:sgl)
        n1249 = property on="泵滴定数4" class="DigNum (严格)"("Val(Sgnl)"=w2074) -> ()  [unwired: 2 in, 2 out]
      }
      event "泵滴定数5": Mouse Down {
        n1250 = event-data() -> ()  [unwired: 1 in, 8 out]
        n1251 = local read "泵滴定数5"() -> (w2077:dbl)
        n1252 = call "数字键盘.vi"("OldNumber"=w2077) -> ("NewNumber"=w2076:sgl)
        n1253 = property on="泵滴定数5" class="DigNum (严格)"("Val(Sgnl)"=w2076) -> ()  [unwired: 2 in, 2 out]
      }
      event "低切高阈值:", "高切低阈值:": Mouse Down {
        n1254 = event-data() -> ("CtlRef"=w2081:refnum<vi>)  [unwired: 1 in, 7 out]
        n1255 = property class="DigNum (严格)"(reference=w2081) -> (reference out=w2080:refnum<vi>, "Value"=w2079:dbl)  [unwired: 1 in, 1 out]
        n1256 = call "数字键盘.vi"("OldNumber"=w2079) -> ("NewNumber"=w2078:sgl)
        n1257 = property class="DigNum (严格)"(reference=w2080, "Val(Sgnl)"=w2078) -> ()  [unwired: 1 in, 2 out]
      }
      event "远程自动校准浓度": Mouse Down {
        n1258 = event-data() -> ("CtlRef"=w2082:refnum<vi>)  [unwired: 1 in, 7 out]
        n1259 = One Button Dialog(message="请输入其中一个在拟合公式中的非零浓度，用于远程校标！" ("消息")) -> (true=w2084:bool)  [unwired: 1 in]
        n1260 = case shown="真" w2084 {
          tunnel: w2082 -> [_ w2091]
          frame False {
          }
          frame True {
            n1261 = property class="DigNum (严格)"(reference=w2091) -> (reference out=w2086:refnum<vi>, "Value"=w2092:dbl)  [unwired: 1 in, 1 out]
            n1262 = global read "COD内部交互全局.vi" "启用的浓度数组"() -> (w2088:dbl[])
            n1263 = call "数字键盘.vi"("OldNumber"=w2092) -> ("NewNumber"=w2085:sgl)
            n1264 = Search 1D Array(1D array=w2088, element=w2085) -> (index of element=w2089:i32)  [unwired: 1 in]
            n1265 = Equal?(x=w2089, y=-1) -> (x = y?=w2087:bool)
            n1266 = case shown="真" w2087 {
              tunnel: w2086 -> [w2094 _]
              tunnel: w2085 -> [w2093 _]
              frame False {
                n1267 = property class="DigNum (严格)"(reference=w2094, "Val(Sgnl)"=w2093) -> ()  [unwired: 1 in, 2 out]
              }
              frame True {
                n1268 = One Button Dialog(message="该浓度不属于校准浓度范围，请重新输入！" ("消息")) -> ()  [unwired: 1 in, 1 out]
              }
            }
          }
        }
      }
    }
  }
  n1269 = while {
    stop <- FALSE stop-if-true
    # "滚动显示"
    n1270 = global read "COD内部交互全局.vi" "待机"() -> (w2096:bool)
    n1271 = case shown="假" w2096 {
      frame False {
        # "运行中"
        n1272 = global read "COD内部交互全局.vi" "校准内容显示"() -> (w2099:string)
        n1273 = while {
          shift-right: [w2101] -> _
          shift-left: w2099 -> [w2106]
          stop <- w2100 stop-if-true
          (unwired) "仪器校准中!\n当前校准浓度为:3mg/L" ("校准内容显示")
          n1274 = Wait (ms)(milliseconds to wait=u32 500 ("等待时间（毫秒）")) -> ()  [unwired: 1 out]
          n1275 = Spreadsheet String To Array(delimiter (Tab)="\n" ("分隔符(Tab)"), format string="" ("格式字符串"), spreadsheet string=w2106, array type (2D Dbl)=string[] []) -> (array=w2109:string[])
          n1276 = for {
            tunnel: w2109 -> [w2117] mode=indexing
            tunnel: [w2115] -> _ mode=indexing
            shift-right: [w2113] -> w2104
            shift-left: "" ("格式字符串") -> [w2114]
            n1277 = call "字符串移位显示.vi"("字符框大小"=36, "字符串输入"=w2117) -> ("移位后字符串"=w2115:string)  [unwired: 8 in, 1 out]
            n1278 = Concatenate Strings(w2114, w2115, "\n" ("分隔符(Tab)")) -> (w2113:string)
          }
          n1279 = String Length(string=w2104) -> (length=w2103:i32)
          n1280 = Decrement(x=w2103) -> (x-1=w2102:i32)
          n1281 = String Subset(string=w2104, length (rest)=w2102) -> (substring=w2101:string)  [unwired: 1 in]
          "校准内容显示" <- w2101
          n1282 = global read "COD内部交互全局.vi" "待机"() -> (w2100:bool)
        }
      }
      frame True {
      }
    }
    n1283 = Wait (ms)(milliseconds to wait=u32 1000 ("等待时间（毫秒）")) -> ()  [unwired: 1 out]
  }
  n1284 = while {
    stop <- FALSE stop-if-true
    # "相差60秒自动校时"
    n1285 = global read "运行时序全局变量.vi" "多列列表框"() -> (w2119:i32)
    n1286 = local read "仪器时间"() -> (w2126:timestamp)
    n1287 = local read "系统时间"() -> (w2127:timestamp)
    n1288 = Wait (ms)(milliseconds to wait=u32 1000 ("等待时间（毫秒）")) -> ()  [unwired: 1 out]
    n1289 = Build Array(w2126) -> (w2125:timestamp[])
    n1290 = Build Array(w2127) -> (w2144:timestamp[])
    n1291 = Equal?(x=w2119, y=u16 5) -> (x = y?=w2121:bool)
    n1292 = call <vilib>:"Boolean Crossing PtByPt.vi"("direction"=enum16{"either", "false-true", "true-false"}."false-true", "input"=w2121) -> ("crossing"=w2118:bool)  [unwired: 1 in]
    n1293 = call "DateToHex.vi"("DATE"=w2125) -> ("数组"=w2138:u16[])  [unwired: 10 in]
    n1294 = call "DateToHex.vi"("DATE"=w2144) -> ("数组"=w2143:u16[])  [unwired: 10 in]
    n1295 = case shown="真" w2118 {
      frame False {
      }
      frame True {
        # "校准结束后自动更新曲线泵滴定数"
        n1296 = global read "COD测量模式全局.vi" "测量模式文字实时"() -> (w2145:string)
        n1297 = global read "COD测量模式全局.vi" "测量模式文字实时"() -> (w2150:string)
        n1298 = global read "CODMN外部API.vi" "远程反控校准CODMn"() -> (w2149:bool)
        n1299 = global read "COD内部交互全局.vi" "高锰酸钾"() -> (w2153:dbl)
        n1300 = Equal?(x=w2145, y="校零") -> (x = y?=w2146:bool)
        n1301 = Equal?(x=w2150, y="校标") -> (x = y?=w2152:bool)
        n1302 = Or(x=w2146, y=w2152) -> (x .or. y?=w2148:bool)
        n1303 = case shown="真" w2148 {
          tunnel: w2153 -> [_ w2160]
          tunnel: w2145 -> [_ w2157]
          frame False {
          }
          frame True {
            w2184 = "量程选择" ("section")
            n1304 = global read "CODMN外部API.vi" "ping"() -> (w2195:bool)
            n1305 = case shown="\"校零\"" w2157 {
              tunnel: ["标样校准时间：" "空白校准时间："] -> w2163
              frame "校标", Default {
              }
              frame "校零" {
              }
            }
            n1306 = case shown="假" w2195 {
              tunnel: [w2204 w2207] -> w2196
              frame False {
                n1307 = global read "COD内部交互全局.vi" "配置文件ini"() -> (w2206:string)
                n1308 = call <vilib>:"Application Directory.vi"() -> ("Application Directory"=w2205:path)
                n1309 = Build Path(base path=w2205, name or relative path=w2206) -> (appended path=w2204:path)
              }
              frame True {
                n1310 = global read "CODMN外部API.vi" "配置文件 path"() -> (w2207:path)
              }
            }
            n1311 = Number To Fractional String(number=w2160) -> (F-format string=w2165:string)  [unwired: 3 in]
            n1312 = call <vilib>:"Open Config Data.vi"("configuration file path"=w2196) -> ("error out"=w2183:errorcluster, "refnum"=w2182:T6)  [unwired: 8 in, 1 out]
            n1313 = Get Date/Time In Seconds() -> (seconds since 1Jan1904=w2161:timestamp)
            n1314 = Format Date/Time String(time format string (%c)="%Y/%m/%d %H:%M:%S" ("时间格式字符串(%c)"), seconds (now)=w2161) -> (date/time string=w2162:string)  [unwired: 1 in]
            n1315 = call-poly <vilib>:"Read Key.vi"("section"="标线选择", "error in (no error)"=w2183, "key"="选用水样", "refnum"=w2182) -> ("error out"=w2185:errorcluster, "value"=w2178:i32, "refnum out"=w2186:T6)  [unwired: 4 in, 1 out]
            n1316 = local write "选用水样"(w2178) -> ()
            n1317 = call-poly <vilib>:"Read Key.vi"("section"=w2184, "error in (no error)"=w2185, "key"=w2184, "refnum"=w2186) -> ("error out"=w2179:errorcluster, "value"=w2181:i32, "refnum out"=w2180:T6)  [unwired: 4 in, 1 out]
            n1318 = case shown="1" w2178 {
              tunnel: ["葡萄糖标线" ("section") "草酸钠标线" ("section")] -> w2193
              frame 0, Default {
              }
              frame 1 {
              }
            }
            n1319 = local write "量程选择"(w2181) -> ()
            n1320 = case shown="2" w2181 {
              tunnel: ["低量程" "高量程" "0-2量程"] -> w2192
              frame 0, Default {
              }
              frame 1 {
              }
              frame 2 {
              }
            }
            n1321 = Concatenate Strings(w2193, w2192) -> (w2194:string)
            n1322 = call-poly <vilib>:"Read Key.vi"("section"=w2194, "error in (no error)"=w2179, "key"="当前选用的校准" ("section"), "refnum"=w2180) -> ("error out"=w2191:errorcluster, "value"=w2156:i32, "refnum out"=w2190:T6)  [unwired: 4 in, 1 out]
            n1323 = call <vilib>:"Close Config Data.vi"("error in (no error)"=w2191, "refnum"=w2190) -> ()  [unwired: 8 in, 2 out]
            n1324 = case shown="2" w2156 {
              tunnel: [w2197 w2198 w2199 w2200 w2201] -> w2155
              frame 1, Default {
                n1325 = local read "浓度1"() -> (w2197:dbl)
              }
              frame 2 {
                n1326 = local read "浓度2"() -> (w2198:dbl)
              }
              frame 3 {
                n1327 = local read "浓度3"() -> (w2199:dbl)
              }
              frame 4 {
                n1328 = local read "浓度4"() -> (w2200:dbl)
              }
              frame 5 {
                n1329 = local read "浓度5"() -> (w2201:dbl)
              }
            }
            n1330 = Number To Fractional String(number=w2155) -> (F-format string=w2167:string)  [unwired: 3 in]
            n1331 = Concatenate Strings("信息：校准结果：\n", "校准浓度：", w2167, "滴定数：", w2165, w2163, w2162) -> (w2159:string)
            n1332 = Bundle(cluster=T15 {"时间标识"=timestamp(0 s since 1904-01-01), "参数"="", "日志信息"="", "流程参数"=""} ("data in"), "时间标识"=w2161, "参数"="CODMn" ("table输入"), "日志信息"=w2159, "流程参数"="" ("table输入")) -> (w2171:T15)
            n1333 = call "流程日志字段定义.vi"("table输入"="校准记录", "data in"=w2171) -> ("table输出"=w2175:string, "columns"=w2176:string[], "data out"=w2177:T19)  [unwired: 7 in]
            n1334 = call "插入数据.vi"("data"=w2177, "columns"=w2176, "database"="database3.mdb", "table"=w2175) -> ()  [unwired: 7 in, 1 out]
            n1335 = global write "COD内部交互全局.vi" "当前校准"(w2156) -> ()
            n1336 = case shown="1, 默认" w2156 {
              tunnel: w2160 -> [w2213 w2214 w2215 w2216 w2217]
              frame 1, Default {
                n1337 = property on="泵滴定数1" class="DigNum (严格)"("Val(Sgnl)"=w2213) -> ()  [unwired: 2 in, 2 out]
              }
              frame 2 {
                n1338 = property on="泵滴定数2" class="DigNum (严格)"("Val(Sgnl)"=w2214) -> ()  [unwired: 2 in, 2 out]
              }
              frame 3 {
                n1339 = property on="泵滴定数3" class="DigNum (严格)"("Val(Sgnl)"=w2215) -> ()  [unwired: 2 in, 2 out]
              }
              frame 4 {
                n1340 = property on="泵滴定数4" class="DigNum (严格)"("Val(Sgnl)"=w2216) -> ()  [unwired: 2 in, 2 out]
              }
              frame 5 {
                n1341 = property on="泵滴定数5" class="DigNum (严格)"("Val(Sgnl)"=w2217) -> ()  [unwired: 2 in, 2 out]
              }
            }
          }
        }
        n1342 = case shown="真" w2149 {
          frame False {
          }
          frame True {
            # "校准完自动写入公式"
            n1343 = global write "CODMN外部API.vi" "远程反控校准CODMn"(FALSE ("远程反控校准CODMn")) -> ()
          }
        }
      }
    }
    n1344 = Index Array(array=w2138, index=2 ("索引")) -> (element=w2140:u16)
    n1345 = Index Array(array=w2143, index=2 ("索引")) -> (element=w2141:u16)
    n1346 = Split Number(x=w2140) -> (hi(x)=w2134:u8)  [unwired: 1 out]
    n1347 = Split Number(x=w2141) -> (hi(x)=w2137:u8)  [unwired: 1 out]
    n1348 = To Byte Integer(number=w2134) -> (8bit integer=w2133:i8)
    n1349 = To Byte Integer(number=w2137) -> (8bit integer=w2136:i8)
    n1350 = Subtract(x=w2133, y=w2136) -> (x-y=w2135:i8)
    n1351 = Absolute Value(x=w2135) -> (abs(x)=w2132:i8)
    n1352 = local read "通讯状态"() -> (w2129:bool)
    n1353 = Greater Or Equal?(x=w2132, y=i8 5) -> (x >= y?=w2130:bool)
    n1354 = And(x=w2130, y=w2129) -> (x .and. y?=w2128:bool)
    n1355 = case shown="真" w2128 {
      frame False {
      }
      frame True {
        # "相差60秒时间自动校准"
        n1356 = flat-sequence {
          frame #0 {
            n1357 = property on="时间校准" class="Bool (严格)"("Val(Sgnl)"=TRUE ("值(信号)")) -> ()  [unwired: 2 in, 2 out]
          }
          frame #1 {
            n1358 = Wait (ms)(milliseconds to wait=u32 500 ("等待时间（毫秒）")) -> ()  [unwired: 1 out]
          }
          frame #2 {
            n1359 = property on="时间校准" class="Bool (严格)"("Val(Sgnl)"=FALSE ("值(信号)")) -> ()  [unwired: 2 in, 2 out]
          }
        }
      }
    }
  }
  n1360 = while {
    stop <- FALSE stop-if-true
    w2254 = T20 0 items=["最小二乘", "最小绝对残差", "Bisquare"] ("method")
    # "计算线性、多项式公式、远程校准"
    n1361 = local read "浓度1"() -> (w2227:dbl)
    n1362 = local read "浓度2"() -> (w2256:dbl)
    n1363 = local read "浓度3"() -> (w2257:dbl)
    n1364 = local read "浓度4"() -> (w2249:dbl)
    n1365 = local read "浓度5"() -> (w2248:dbl)
    n1366 = Build Array("泵滴定数1", "泵滴定数2", "泵滴定数3", "泵滴定数4", "泵滴定数5") -> (w2255:dbl[])
    n1367 = Build Array(w2227, w2256, w2257, w2249, w2248) -> (w2223:dbl[])
    n1368 = Build Array("启用1", "启用2", "启用3", "启用4", "启用5") -> (w2226:bool[])
    n1369 = global read "CODMN外部API.vi" "远程反控校准CODMn"() -> (w2224:bool)
    n1370 = call "将启用的浓度作为新的浓度数组.vi"("启用布尔数组"=w2226, "输入浓度数组"=w2223) -> ("启用的浓度数组"=w2225:dbl[])  [unwired: 13 in]
    n1371 = Unbundle By Name("方程系数") -> ("K"=w2235:dbl, "b"=w2234:dbl, "X^2"=w2233:dbl)
    n1372 = case shown="\"多项式\"" "模型" {
      tunnel: w2235 -> [w2266 w2269]
      tunnel: w2234 -> [w2265 w2270]
      tunnel: w2233 -> [_ w2268]
      frame "线性", Default {
        "K" <- w2266
        "b" <- w2265
      }
      frame "多项式" {
        n1373 = Build Array(w2270, w2269, w2268) -> (→"多项式系数":dbl[])
      }
    }
    n1374 = call "线性公式CODMn用.vi"("标液浓度"=w2223, "监测浓度"=w2255, "启用"=w2226, "method"=w2254, "模型"="模型", "精度"=6) -> ("拟合方程"=w2241:string, "r^2"=→"r^2":dbl, "slope"=w2239:dbl, "intercept"=w2240:dbl, "XY图"=→"XY图":cluster{"X Values":dbl[], "Y Values":dbl[]}[], "Polynomial Coefficients"=w2250:dbl[])  [unwired: 8 in]
    "拟合公式" <- w2241
    n1375 = call <vilib>:"Boolean Crossing PtByPt.vi"("direction"=enum16{"either", "false-true", "true-false"}."false-true", "input"=w2224) -> ("crossing"=w2222:bool)  [unwired: 1 in]
    n1376 = case shown="真" w2222 {
      tunnel: w2223 -> [_ w2260]
      frame False {
      }
      frame True {
        n1377 = global read "CODMn断电保存全局变量.vi" "远程自动校准浓度"() -> (w2261:dbl)
        n1378 = Search 1D Array(1D array=w2260, element=w2261) -> (index of element=w2262:i32)  [unwired: 1 in]
        n1379 = case shown="0, 默认" w2262 {
          selector: w2262 -> [_ w2264]
          frame -1 {
          }
          frame 0, Default {
            n1380 = Increment(x=w2264) -> (x+1=w2263:i32)
            n1381 = global write "COD内部交互全局.vi" "当前校准"(w2263) -> ()
          }
        }
      }
    }
    n1382 = feedback #3(w2241) -> (w2242:string)
    n1383 = feedback-in #3(w2241) -> ()
    n1384 = Not Equal?(x=w2241, y=w2242) -> (x != y?=w2238:bool)
    n1385 = global write "COD内部交互全局.vi" "启用的浓度数组"(w2225) -> ()
    n1386 = case shown="真" w2238 {
      tunnel: w2250 -> [_ w2274]
      tunnel: w2240 -> [_ w2275]
      tunnel: w2239 -> [_ w2276]
      frame False {
      }
      frame True {
        # "当公式发生改变时赋值到右侧公式"
        n1387 = local read "模型"() -> (w2277:enum32{"线性", "多项式"})
        n1388 = case shown="\"多项式\"" w2277 {
          tunnel: [w2282 w2284] -> w2272
          tunnel: w2276 -> [w2282 _]
          tunnel: w2275 -> [w2281 _]
          tunnel: [w2281 w2285] -> w2273
          tunnel: w2274 -> [_ w2286]
          tunnel: [0.0 ("数值") w2283] -> w2271
          frame "线性", Default {
          }
          frame "多项式" {
            # "B,K,X^2"
            n1389 = Index Array(array=w2286) -> (element #1=w2285:dbl, element #2=w2284:dbl, element #3=w2283:dbl)  [unwired: 3 in]
          }
        }
        n1390 = Bundle By Name(cluster=cluster{"K":dbl, "b":dbl, "X^2":dbl} {"K"=0.0, "b"=0.0, "X^2"=0.0} ("方程系数"), "K"=w2272, "b"=w2273, "X^2"=w2271) -> (w2278:cluster{"K":dbl, "b":dbl, "X^2":dbl})
        n1391 = local write "方程系数"(w2278) -> ()
      }
    }
    n1392 = Wait (ms)(milliseconds to wait=u32 1000 ("等待时间（毫秒）")) -> ()  [unwired: 1 out]
  }
  n1393 = property class="VI"(reference=w6, error in=w3) -> ("Name"=w7:string)  [unwired: 2 out]
  n1394 = Open VI Reference(type specifier VI Refnum (for type only)=refnum<vi> refnum, vi path=w7, options=128 ("选项")) -> (vi reference=w9:refnum<vi>, error out=w11:errorcluster)  [unwired: 3 in]
  n1395 = call-by-ref "?"(reference=w9, error in=w11) -> (reference out=w13:refnum<vi>, error out=w12:errorcluster)  [unwired: 12 in]
  n1396 = Close Reference(reference=w13, error in (no error)=w12) -> ()  [unwired: 1 out]
